vi "Results_file_Plotter.vi"(2 "flushAll":bool) -> ()   [LabVIEW 2022 SP3]
uses:
  Anemometry/Anemometry Sub Vis/Data_plotting_vis/Plotter_Mode.ctl
  Anemometry/Anemometry Sub Vis/Data_plotting_vis/Data_File_Type.ctl
  subVIs/PlotProperty.ctl
  <vilib>/Math Plots/3D Math Plots/3D Surface/3D Surface XCtrl/3D Surface.xctl
  <vilib>/Math Plots/3D Math Plots/3D Stem/3D Stem XCtrl/3D Stem.xctl
  Anemometry/Anemometry Sub Vis/File/Setup_Filetype.ctl
  Anemometry/Anemometry Sub Vis/Controls/Global_mode.ctl
  Anemometry/Anemometry Sub Vis/Data_plotting_vis/Error_bars_index.ctl
  Anemometry/Anemometry Sub Vis/Data_plotting_vis/All_Setup.ctl
  <vilib>/Utility/miscctls.llb/LVBoundsTypeDef.ctl
  35570bf4-7d7d-495b-8c89-e9310c8e2c93.vi
  f4d116b7-bb04-d342-9616-30c9bd5cd225.vi
  50b9f45c-b768-454c-9e58-04e6880f7924.vi
  443f2c7a-355d-e746-9bc2-19f18202945d.vi
  c22539af-4616-b947-8dc9-59d74accf1f9.vi
  <vilib>/Utility/error.llb/Trim Whitespace One-Sided.vi
  Anemometry/Anemometry Sub Vis/Globals/Constants_global.vi
  Anemometry/Anemometry Sub Vis/Data_plotting_vis/Results_plotter_Global.vi
  <vilib>/picture/3D Picture Control/Helpers/Set Light (no reference).vi
  <vilib>/picture/3D Picture Control/Object/Add Object (reference).vi
  subVIs/Plot_Values_Global.vi
  <vilib>/Math Plots/3D Math Plots/3D Stem/3D Stem Datatype/Public/Plot Helper (Matrix).vi
  <vilib>/Analysis/1siggen.llb/Ramp Pattern by Delta.vi
  <vilib>/Math Plots/3D Math Plots/3D Surface/3D Surface Datatype/Public/Plot Helper (Matrix).vi
  Instance           1 28Saved   Results_file_Plotter .vi
  subVIs/RFP_Table_Global.vi
  Anemometry/Anemometry Sub Vis/Globals/Meas_global.vi
  Anemometry/Anemometry Sub Vis/Globals/Plug_in_data_global.vi
  Anemometry/Anemometry Sub Vis/Globals/Trav_pos_global.vi
  <vilib>/picture/3D Picture Control/NI_3D Picture Control.lvlib
  <vilib>/Math Plots/3D Math Plots/3D Surface/3D Surface Datatype/3D Surface Datatype.lvclass
  <vilib>/Math Plots/3D Math Plots/3D Stem/3D Stem Datatype/3D Stem Datatype.lvclass
  f03f3b4b-6808-4e33-b687-4131ee4846c6.vi
  <vilib>/Analysis/NI_AALBase.lvlib
  <vilib>/Analysis/NI_AALPro.lvlib
panel:
  out "whereNext 3":string="Time to save setup?"
  out "whereNext 2":string="Time to save setup?"
  out "Time to Save Setup?":bool
  out "closePressed":bool=TRUE
  out "Template Last Mod":timestamp
  out "Index when last displayed":i32
  in  "Tab Control":T1(tab)
  in  "revealDataFiles":bool
  in  "Template":path=path ""
  in  "flushFiles":bool
  in  "Result files to read":path[](array[path])
  in  "Add results file":bool
  in  "File Types to Read":T2
  in  "SearchX":string
  in  "SearchY":string
  in  "Show Results Space Analysis":bool
  in  "Show Plot Space Analysis":bool
  in  "Multi Ordinate":i32[](listbox)
  in  "Absisca":u16(ring) items=["3818592258.491 3818596078.981 3818596814.909", "Camserver Camserver Camserver", "2025-01-01 09 04 2025-01-01 10", "Current File", "Current File 1st Folder level", "Current File 2nd Folder level", "Current File 3rd Folder level", "Current File 4th Folder level", "Current File Number", "Current Filepath", "Template File Used"]
  in  "revealOutputFile":bool
  in  "openJobDir":bool
  in  "Job Directory":path
  in  "Save Averaged rows":bool
  in  "Save Surface Fit":bool
  in  "Output Filename":path
  in  "Save Data in Rows":bool
  in  "Save Plot data":bool
  in  "Header":string
  in  "Process Point":bool
  in  "Kill Point":bool
  out "dataTable":string[][](table)
  in  "ShowPix":bool
  in  "picMode":enum32{"Scrub", "Jump"}(radio)=enum."Jump"
  in  "Post Process Plotted Data":bool
  in  "...using routine":string(combo)
  in  "Calculate new metadata":bool
  in  "Add /Edit metadata":bool
  in  "Delete Plotted data from file":bool
  in  "Raw DF in Orig Pos?":bool
  in  "Edit Raw Data Files?":bool
  in  "Point ID":u16(ring) items=["None", "3818592258.491 3818596078.981 3818596814.909", "Camserver Camserver Camserver", "2025-01-01 09 04 2025-01-01 10", "Current File", "Current File 1st Folder level", "Current File 2nd Folder level", "Current File 3rd Folder level", "Current File 4th Folder level", "Current File Number", "Current Filepath", "Template File Used"]
  in  "Won":bool=TRUE
  in  "Von":bool=TRUE
  in  "Uon":bool=TRUE
  in  "Zon":bool=TRUE
  in  "Yon":bool=TRUE
  in  "Xon":bool=TRUE
  in  "W Ch Name":u16(ring) items=["None", "3818592258.491 3818596078.981 3818596814.909", "Camserver Camserver Camserver", "2025-01-01 09 04 2025-01-01 10", "Current File", "Current File 1st Folder level", "Current File 2nd Folder level", "Current File 3rd Folder level", "Current File 4th Folder level", "Current File Number", "Current Filepath", "Template File Used"]
  in  "V Ch Name":u16(ring) items=["None", "3818592258.491 3818596078.981 3818596814.909", "Camserver Camserver Camserver", "2025-01-01 09 04 2025-01-01 10", "Current File", "Current File 1st Folder level", "Current File 2nd Folder level", "Current File 3rd Folder level", "Current File 4th Folder level", "Current File Number", "Current Filepath", "Template File Used"]
  in  "U Ch Name":u16(ring) items=["None", "3818592258.491 3818596078.981 3818596814.909", "Camserver Camserver Camserver", "2025-01-01 09 04 2025-01-01 10", "Current File", "Current File 1st Folder level", "Current File 2nd Folder level", "Current File 3rd Folder level", "Current File 4th Folder level", "Current File Number", "Current Filepath", "Template File Used"]
  in  "stl Filename":u16(ring) items=["None", "3818592258.491 3818596078.981 3818596814.909", "Camserver Camserver Camserver", "2025-01-01 09 04 2025-01-01 10", "Current File", "Current File 1st Folder level", "Current File 2nd Folder level", "Current File 3rd Folder level", "Current File 4th Folder level", "Current File Number", "Current Filepath", "Template File Used"]
  in  "Coord System":u16(ring) items=["None", "3818592258.491 3818596078.981 3818596814.909", "Camserver Camserver Camserver", "2025-01-01 09 04 2025-01-01 10", "Current File", "Current File 1st Folder level", "Current File 2nd Folder level", "Current File 3rd Folder level", "Current File 4th Folder level", "Current File Number", "Current Filepath", "Template File Used"]
  in  "Wind Direction":u16(ring) items=["None", "3818592258.491 3818596078.981 3818596814.909", "Camserver Camserver Camserver", "2025-01-01 09 04 2025-01-01 10", "Current File", "Current File 1st Folder level", "Current File 2nd Folder level", "Current File 3rd Folder level", "Current File 4th Folder level", "Current File Number", "Current Filepath", "Template File Used"]
  in  "X Ch Name":u16(ring) items=["None", "3818592258.491 3818596078.981 3818596814.909", "Camserver Camserver Camserver", "2025-01-01 09 04 2025-01-01 10", "Current File", "Current File 1st Folder level", "Current File 2nd Folder level", "Current File 3rd Folder level", "Current File 4th Folder level", "Current File Number", "Current Filepath", "Template File Used"]
  in  "Y Ch Name":u16(ring) items=["None", "3818592258.491 3818596078.981 3818596814.909", "Camserver Camserver Camserver", "2025-01-01 09 04 2025-01-01 10", "Current File", "Current File 1st Folder level", "Current File 2nd Folder level", "Current File 3rd Folder level", "Current File 4th Folder level", "Current File Number", "Current Filepath", "Template File Used"]
  in  "Z Ch Name":u16(ring) items=["None", "3818592258.491 3818596078.981 3818596814.909", "Camserver Camserver Camserver", "2025-01-01 09 04 2025-01-01 10", "Current File", "Current File 1st Folder level", "Current File 2nd Folder level", "Current File 3rd Folder level", "Current File 4th Folder level", "Current File Number", "Current Filepath", "Template File Used"]
  in  "exportSetup":bool
  in  "importSetup":bool
  in  "Save Setup":bool
  in  "loadSetup":bool
  out "setupOrINI":path
  out "loadingSetup":bool
  out "importingSetup":bool
  in  "Add Inlet Temperature offset":bool
  in  "Plot EnFlo Tunnel Display":bool
  in  "Choose\nPlug ins":bool
  in  "Reload Interval (s)":dbl=200.0 min=10.0 step=20.0
  in  "Save Setup Interval (s)":dbl=600.0
  out "Uadvec":dbl
  in  "Per Block Plug Ins Extra":string[](array[string])
  in  "Max no of filter options":i32=2000
  in  "Additional Y Values":dbl[](array[numeric]) format="%.2f"
  in  "Additional X Values":dbl[](array[numeric]) format="%.2f"
  in  "notSelectors?":bool
  in  "graphBackground":u32(colorbox)=16777222
  in  "axes":T3(ring)
  in  "brewSelect":i32 min=0 max=3 step=1
  in  "seriesColours":enum32{"Item 0", "Item 1"}(radio)
  in  "SeriesColouring":T5={"PlotVariable"=enum."Symbol", "YellowSelector"=enum."Colour", "RedSelector"=enum."Shade"}
  in  "InterpolationStyle":T6(ring)=enum."Line"
  in  "TinyPoints?":bool
  out "-4":string="Graph Scales"
  out "-3":string="Graph Scales"
  in  "printFP":bool
  out "-2":string="Graph Scales"
  out "loop":i32
  out "-1":string="Graph Scales"
  out "reloadPending":bool
  out "nRows":i32
  out "loadTime(s)":dbl format="Load: %#_3g s"
  in  "stop":bool
  out "Current":string="Graph Scales"
  in  "Single Series":i32[](listbox)=[0]
  in  "Edit Template File":bool
  in  "Filter Bins 2":i32[](listbox)=[0]
  in  "Filter 5":u16(ring)
  in  "Filter 4":u16(ring)
  in  "Filter 3":u16(ring)
  in  "Filter Array":u16[](array[ring])=[0, 0, 0, 0, 0, 0] items=["Don't Filter", "Data Plane", "3818592258.491 3818596078.981 3818596814.909", "Camserver Camserver Camserver", "2025-01-01 09 04 2025-01-01 10", "Current File", "Current File 1st Folder level", "Current File 2nd Folder level", "Current File 3rd Folder level", "Current File 4th Folder level", "Current File Number", "Current Filepath", "Template File Used"]
  in  "Filter Bins 1":i32[](listbox)=[0]
  in  "Create picture Vi Name":string(combo) caption="Picture VI:"
  in  "passToPictureVI":bool
  in  "Reload Files":bool
  out "underCursor":string
  in  "FOV":u8(slide)=4 min=4 max=100 scale=100.0..4.0
  in  "graphPaneTab":T7(tab)
  in  "histOn":bool
  in  "color and symbol":bool
  in  "forceX0":bool
  in  "forceY0":bool
  in  "Transpose":bool
  in  "refresh":bool
  out "Histogram":cluster{"Histogram":i32[], "Axis":dbl[]}[](graph)
  out "XY Plot":cluster{"Array":dbl[], "Array":dbl[]}[](graph)
  in  "Bkgnd Value":dbl
  out "Surface Integral":dbl format="%^_4g"
  out "Surface Average":dbl format="%^#.4g"
  in  "Plot Resolution":bool
  in  "Resolution":dbl=1.0 min=0.0 format="%.4f"
  in  "Point Size":i32(slide)=1 scale=0.0..5.0
  in  "No of Contours":i32(slide)=20 scale=0.0..20.0
  out "Surface Area":dbl format="%^_6g"
  out "Warning!":string
  out "Intensity Graph":dbl[][](graph)
  out "3D Surface":refnum<class "3D Plot Datatype.lvclass">[](xcontrol)
  out "3D Stem":refnum<class "3D Plot Datatype.lvclass">[](xcontrol)
  in  "3Dcontrols":enum32{"Vectors", "STL", "Cam"}(tab)
  in  "Key":dbl(ramp)
  out "scalar":string
  in  "vectorDims":cluster{"vectorSize":sgl, "vectorScale":dbl}={"vectorSize"=3.0, "vectorScale"=5.0} {"vectorScale" min=1.0 max=1000.0; "vectorSize" min=1 max=50 format="%#_3g"}
  in  "keySettings":T8 {"clipPercentile" min=0.0 max=100.0 step=0.1 format="%#_g%%"}
  in  "Tunnel":cluster{"colour":u32, "Alpha":sgl}={"colour"=16630148, "Alpha"=1.0} {"Alpha" min=0.2 max=1 step=0.02}
  in  "axesLength":dbl=150.0
  in  "BGcolour":u32(colorbox)=2829099
  in  "TTshift":T9={"STLscale"=1.0, "STLdTheta"=0.0, "Translation"={"dX"=0.0, "dY"=0.0, "dZ"=0.0}} {"STLdTheta" min=0.0 max=360.0 step=1.0}
  in  "Turntable":cluster{"colour":u32, "Alpha":sgl}={"colour"=32639, "Alpha"=1.0} {"Alpha" min=0.2 max=1 step=0.02}
  in  "Light State":bool
  in  "lightPos":cluster{"X":dbl, "Y":dbl, "Z":dbl}={"X"=-15000.0, "Y"=2000.0, "Z"=2000.0}
  in  "depthClipping":cluster{sgl, sgl}(slide)={0.001, 10.0} scale=0.001..20.0 scale format="%.0pm"
  in  "3D Picture":refnum<vi>(3d-picture)
  out "error out":errorcluster
  out "Array":errorcluster[](array[cluster])
  in  "Vector Plot?":bool
  in  "Dot Plot?":bool
  in  "Intensity Plot?":bool
  in  "MakeMovie":bool
  in  "3Dplotter":bool
  out "3DrawDataPath":path
  out "cursorDrag":bool
  out "RD_Folders":path[](array[path])
  out "whereNext":string="Time to save setup?"
  out "Template Changed?":bool
  in  "Results files chosen":path[](array[path])
  out "File Index":i32
  in  "Filter Bins 2 Strings":string[](array[string])
  in  "Filter Bins 1 Strings":string[](array[string])
  in  "Filters 3 onwards":string[](array[string])
  out "Edit Raw Data Header Info":bool
  out "Non-Blank Rows":bool[](array[boolean])
  out "Plotted rows only?":bool
  in  "type specifier":refnum<vi>
  in  "type specifier2":refnum<vi>
  out "Filetype":string[](array[string])
  out "Plotted Series":bool[][](array[boolean])
  out "Accept Array":bool[][](array[boolean])
  out "Chosen Path":path
  out "Cursor index":i32
  out "Selected Row":i32
  out "justCursorPt":bool
  out "Template Single Values":string[](array[string])
  out "Tolerances":dbl[](array[numeric]) format="%.2f"
  out "Mode":T10
  in  "Full_Res_Results_Folder":path
  in  "VI Refnum Calculation":refnum<vi>
  out "Index when last plotted":i32
  out "tunnelSTLbits":refnum<vi>[](array[refnum])
  out "tunnelRef":refnum<vi>
  out "TTstlBits":refnum<vi>[](array[refnum])
  out "axesRef":refnum<vi>
  out "TTref":refnum<vi>
  out "worldRef":refnum<vi>
  in  "modelColours":u32[](array[colorbox])=[8636267, 16545852, 3381759, 16761088]
  # "Space to put spare indicators for testing"
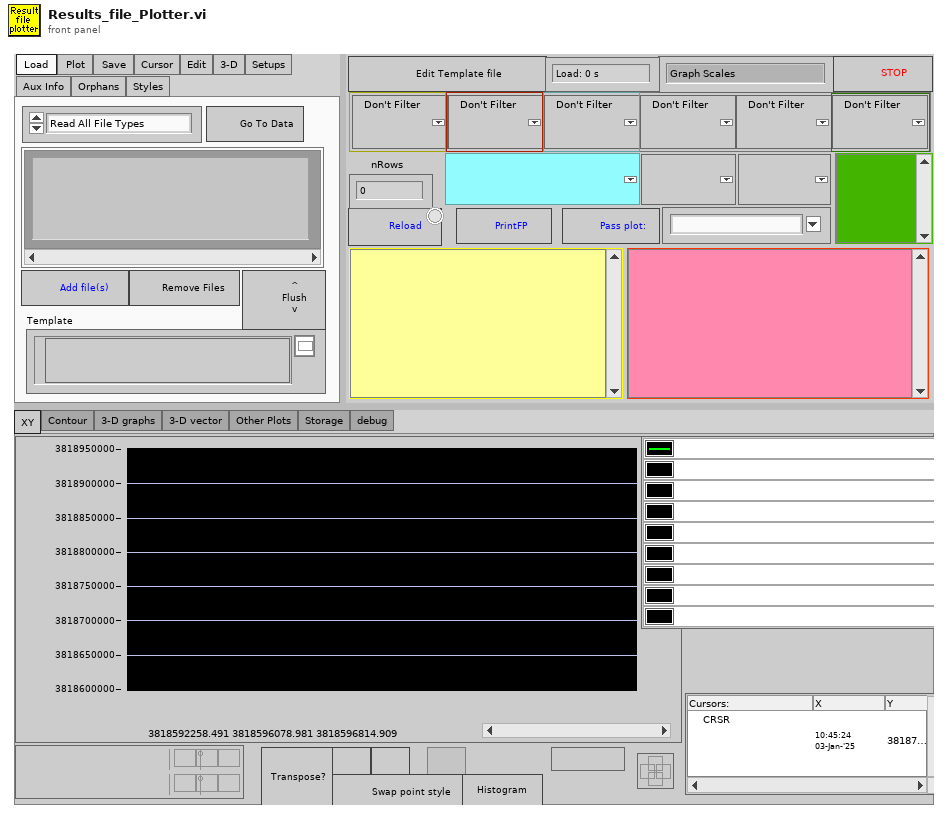
[diagram p1: front panel]
types:
  T1 = enum32{"Load ", "Plot ", "Save ", "Cursor", "Edit", "3-D", "Setups", "Aux Info", "Orphans", "Styles"}
  T2 = typedef "Data_File_Type.ctl" = enum16{"Read All File Types", "Results Files Only", "Raw Data Files Only", "Calibration Files Only", "Gas Desk Files Only", "Old Results Files Only", "Tabulated Data Files Only"}
  T3 = enum16{"X lin Y lin", "X log Y log", "X log Y lin", "X lin Y log"}
  T4 = typedef "PlotProperty.ctl" = enum16{"Colour", "Symbol", "Shade", "Size"}
  T5 = cluster{"PlotVariable":T4, "YellowSelector":T4, "RedSelector":T4}
  T6 = enum16{"Points", "StepLeft", "Line", "StepRight", "StepCentre", "StepEdge"}
  T7 = enum32{"XY", "Contour", "3-D graphs", "3-D vector", "Other Plots", "Storage", "debug"}
  T8 = cluster{"Centre Value":enum16{"Median", "Zero"}, "clipPercentile":dbl}
  T9 = cluster{"STLscale":dbl, "STLdTheta":dbl, "Translation":cluster{"dX":sgl, "dY":sgl, "dZ":sgl}}
  T10 = typedef "Plotter_Mode.ctl" = enum16{"Save file", "Delete unwanted rows", "Edit Values with constants", "Edit values per row", "Edit Raw Data file header", "Post Process Plotted Rows", "Plot EnFlo Tunnel Display", "Add Inlet Temperature Offset"}
  T11 = enum32{"XY", "Contour", "3-D graphs", "3-D vector", "Other Plots", "Storage"}
  T12 = enum16{"Zero or one", "One", "Zero or more", "One or more"}
  T13 = typedef "Global_mode.ctl" = enum16{"Read Global", "Load Global From File", "Write Global to File"}
  T14 = enum32{"Invalid", "Standard", "Closed", "Hidden", "Minimized", "Maximized"}
  T15 = enum16{"Edit Existing Template File", "Create New Template File"}
  T16 = enum16{"Show only data summary", "Show data summary", "No data summary"}
  T17 = typedef "All_Setup.ctl" = cluster{"Result files to read":path[], "Template":path, "Transpose":bool, "Additional X Values":dbl[], "Additional Y Values":dbl[], "Output Filename":path, "Create Picture Vi Name":string, "Intensity Plot?":bool, "Multi Ordinate":string[], "Abscissa String":string, "Filter Array":string[], "Filter Bins 1 Strings":string[], "Filter Bins 2 Strings":string[], "Filters 3 onwards":string[], "nRows":i32}
  T18 = typedef "Setup_Filetype.ctl" = enum16{"Measurement Setups", "Calibration Setups", "General", "Results File Plotter Setups", "Speed Calib Tweaks"}
  T19 = enum16{"Left Button", "Center Button", "Right Button", "Window Close"}
  T20 = cluster{"Filter Bins 2":i32[], "Filter Bins 1":i32[], "Point Size":i32, "color and symbol":bool, "No of Contours":i32, "Resolution":dbl, "Transpose":bool, "Absisca":u16, "Multi Ordinate":i32[], "Accept Array":bool[][], "Intensity Plot?":bool, "Additional X Values":dbl[], "Additional Y Values":dbl[], "3D Ch Selectors":i32[]}
  T21 = typedef "Error_bars_index.ctl" = cluster{"Upper":i32, "Lower":i32, "St Error":i32}
  T22 = typedef "LVPointTypeDef.ctl" = cluster{"Horizontal":i16, "Vertical":i16}
  T23 = typedef "LVRectTypeDef.ctl" = cluster{"Left":i16, "Top":i16, "Right":i16, "Bottom":i16}
  T24 = cluster{"X Max":dbl, "Y Max ":dbl, "X Scale":cluster{"Xo":dbl, "delta X":dbl}, "Y Scale":cluster{"Xo":dbl, "delta X":dbl}, "X Values":dbl[], "Y Values":dbl[], "Z Max":dbl, "Z Min":dbl}
  T25 = typedef "coordSys.ctl" = enum16{"Tunnel", "Model"}
  T26 = cluster{"coordSys":T25, "WD":dbl, "STL":string}[]
  T27 = typedef "Group_Binning.ctl" = cluster{"Index":i32, "Tolerance":dbl, "Precision":string}
  T28 = typedef "LVBoundsTypeDef.ctl" = cluster{"Width":u32, "Height":u32}
  T29 = enum8{"Enabled", "Disabled", "Disabled and Grayed Out"}
  T30 = enum16{"Normal Bin", "Opaque Bin", "Transparent Bin"}
  T31 = typedef "RFP_Plot_Metadata.ctl" = cluster{"Row Number":i32[], "Error Bars":T21, "X Label":string, "Y Label":string, "Blanks NaNs":i32[]}
  T32 = typedef "LVPoint32TypeDef.ctl" = cluster{"Horizontal":i32, "Vertical":i32}
  T33 = typedef "LVRGBAColorTypeDef.ctl" = cluster{"Red":sgl, "Green":sgl, "Blue":sgl, "Alpha":sgl}
  T34 = cluster{"Shift":bool, "Ctrl":bool, "Alt":bool, "Cmd":bool, "Opt":bool}
  T35 = enum16{"Inherit Material", "Use entire Material", "Ignore Ambient", "Ignore Diffuse", "Ignore Specular", "Ignore Emission", "Ignore Ambient and Diffuse"}
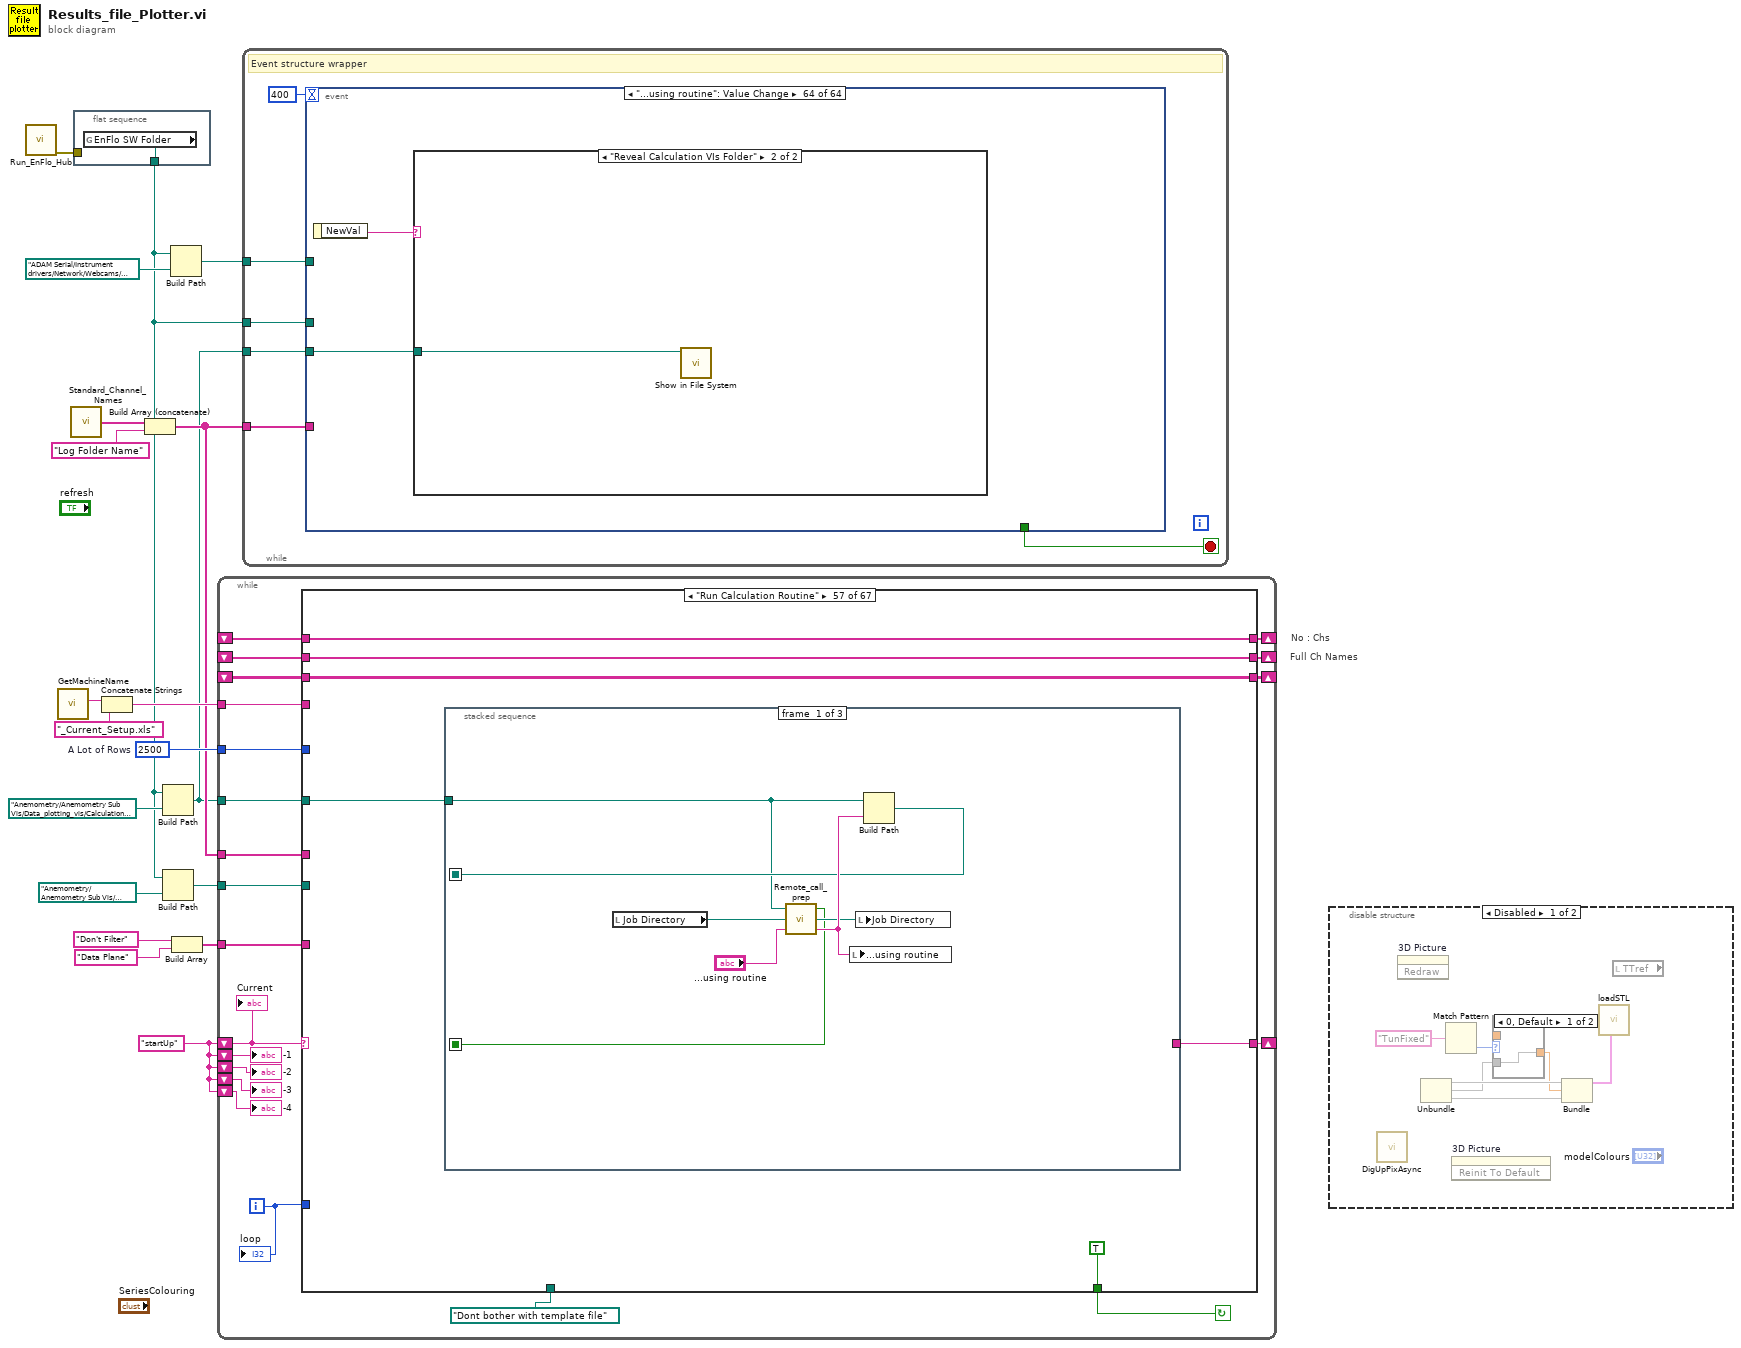
[diagram p0: block diagram]
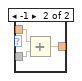
[diagram p2: hidden frame]
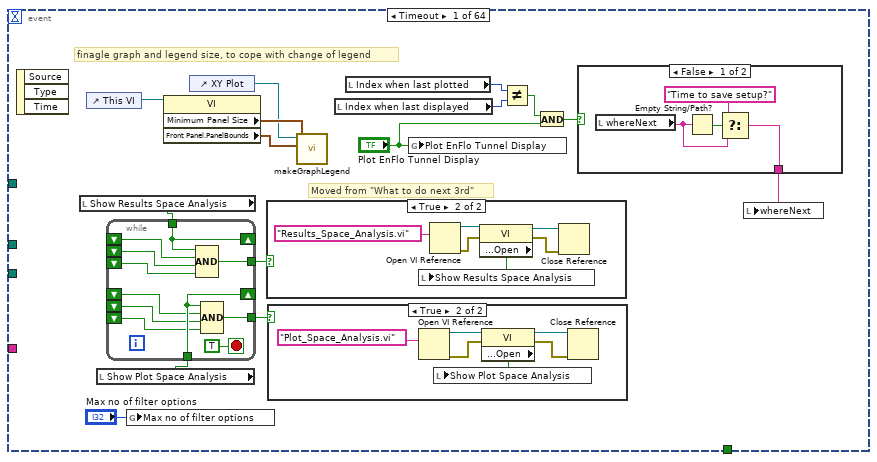
[diagram p4: hidden frame]
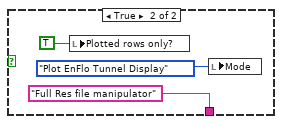
[diagram p5: hidden frame]
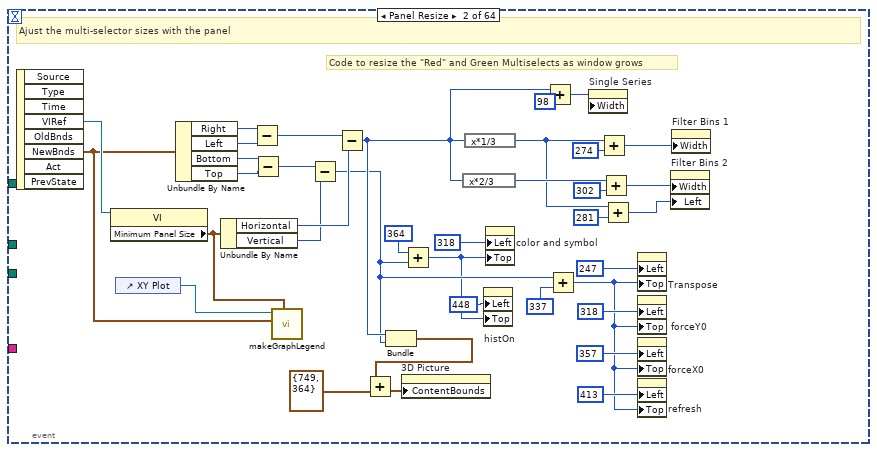
[diagram p8: hidden frame]
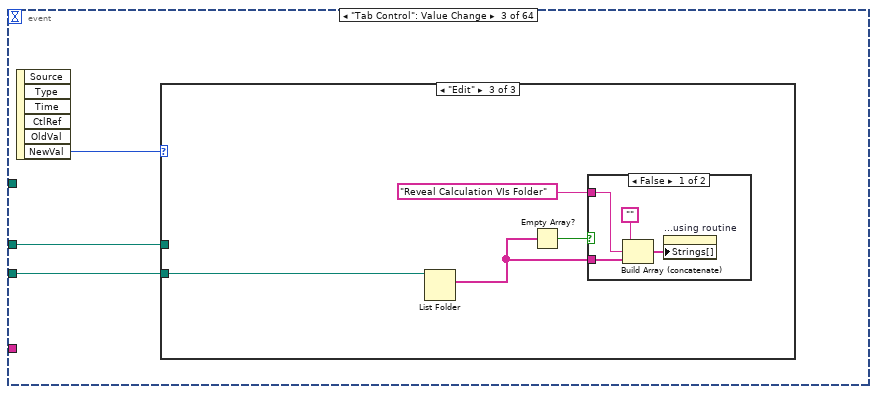
[diagram p9: hidden frame]
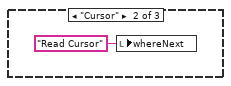
[diagram p11: hidden frame]
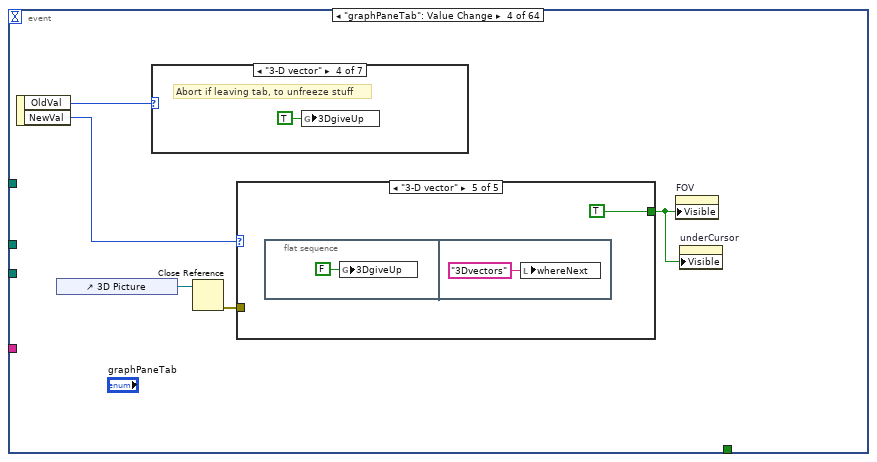
[diagram p13: hidden frame]
diagram:
  w19 = 2500  # A Lot of Rows
  w3 = "startUp"
  # "No : Chs"
  # "Full Ch Names"
  n1 = call "Run_EnFlo_Hub.vi"() -> ("Error Out"=w6:errorcluster)  [unwired: 1 in, 6 out]
  n2 = call "GetMachineName.vi"() -> ("ComputerName"=w16:string)  [unwired: 11 in]
  n3 = call "Standard_Channel_Names.vi"() -> ("Standard Ch Names"=w15:string[])  [unwired: 1 in]
  n4 = flat-sequence {
    tunnel: [w20] -> w2
    tunnel: w6 -> [_]
    frame #0 {
      n5 = global read "Constants_global.vi" "EnFlo SW Folder"() -> (w20:path)
    }
  }
  n6 = Concatenate Strings(w16, "_Current_Setup.xls" ("Setup filename")) -> (w17:string)
  n7 = Build Array (concatenate)(w15, "Log Folder Name") -> (w13:string[])
  n8 = Build Path(base path=w2, name or relative path=path "Anemometry/Anemometry Sub Vis/Data_plotting_vis/Calculation Vis") -> (appended path=w1:path)
  n9 = Build Path(base path=w2, name or relative path=path "Anemometry/Anemometry Sub Vis/Data_plotting_vis/XY Plot Vis") -> (appended path=w8:path)
  n10 = Build Path(base path=w2, name or relative path=path "ADAM Serial/Instrument drivers/Network/Webcams/RetrievePix.vi") -> (appended path=w4:path)
  n11 = Build Array("Don't Filter" ("Input Element"), "Data Plane" ("Input Element")) -> (w10:string[])
  n12 = while {
    shift-left: _ -> [w35]
    shift-right: [w36] -> _
    shift-left: w3 -> [w39]
    shift-right: [w34] -> _
    shift-left: _ -> [w37]
    shift-right: [w41] -> _
    tunnel: w19 -> [w33]
    tunnel: w17 -> [w32]
    tunnel: w13 -> [w29]
    shift-right: [w31] -> _
    shift-left: _ -> [w30]
    shift-left: w3 -> [w28]
    shift-left: w3 -> [w26]
    tunnel: w10 -> [w25]
    tunnel: w8 -> [w24]
    tunnel: w1 -> [w23]
    shift-left: w3 -> [w22]
    shift-left: w3 -> [w21]
    i -> [w27]
    stop <- w40 continue-if-true
    n13 = case shown="\"Run Calculation Routine\"" w39 {
      selector: w39 -> [_ _ _ _ _ _ _ _ _ _ _ _ _ _ _ _ _ _ _ _ _ _ _ _ _ _ _ _ _ _ _ _ _ _ _ _ _ _ _ _ _ _ _ _ _ _ _ _ _ _ _ _ _ _ _ _ _ _ _ _ _ _ _ _ _ _ w3667]
      tunnel: w37 -> [w63 w98 _ w147 w179 w217 w245 w266 w319 w335 w352 w412 w464 w497 w559 w600 w621 w642 w654 w714 w729 w776 w1079 w1151 w1200 w1227 w1240 w1275 w1303 w1450 w1478 w1563 w1895 w1912 w1919 w1937 w1947 w1953 w1973 w2040 w2122 w2145 w2169 w2219 w2266 w2285 w2305 w2519 w2535 w2556 w2637 w2781 w2829 w2842 w2851 w2909 w2927 w2968 w3072 w3123 w3544 w3554 w3616 w3632 w3637 w3658 w3672]
      tunnel: [w63 w98 w119 w147 w179 w217 w245 w263 w319 w335 w365 w423 w464 w497 w559 w600 w621 w642 w654 w714 w729 w776 w1079 w1151 w1200 w1227 w1240 w1275 w1303 w1450 w1478 w1562 w1895 w1912 w1919 w1937 w1947 w1953 w1973 w2040 w2122 w2145 w2169 w2219 w2266 w2285 w2304 w2519 w2535 w2555 w2631 w2781 w2829 w2842 w2851 w2909 w2927 w2968 w3072 w3124 w3544 w3555 w3616 w3632 w3637 w3658 w3672] -> w41
      tunnel: [w52 w72 w110 w136 w174 "Template Required?" "More files options" w267 "Load Data" "Load Data" w363 w421 w466 w495 "Load Selectors" "Perform Global Concatenate" "What is present?" "Ordinate Selector Type" "Which rows are Non-Blank?" w698 "Create Selectors" w764 w1078 w1150 "Re Plot Data?" w1225 "Prepare Filter2 strings" "Plot Data" w1301 "Add Axis names" "Analyse Plot Space" w1564 "What to do next?" ("t") "What to do next?" ("t") "What to do next?" "What to do next?" ("t") "What to do next?" ("t") w1954 w1976 "Check modification dates?" w2118 w2142 "Ordinate Selector Type" w2222 "Initialise" ("t") w2273 w2306 w2511 "Create Selectors" w2557 w2638 w2779 w2822 w2833 w2855 "Create Selectors" w2925 w2971 w3060 w3137 "Initialise" ("t") w3553 "Time to save setup?" "initialise" "Initialise" "" "Initialise"] -> w34
      tunnel: [TRUE TRUE TRUE TRUE TRUE ("T button?") TRUE TRUE TRUE TRUE TRUE w378 TRUE ("OK?") TRUE ("OK?") TRUE ("OK?") TRUE ("OK?") TRUE TRUE TRUE TRUE TRUE TRUE TRUE w1077 w1149 TRUE TRUE TRUE TRUE w1302 TRUE TRUE ("OK?") TRUE TRUE ("OK?") TRUE ("OK?") TRUE TRUE ("OK?") TRUE ("OK?") TRUE ("OK?") TRUE ("OK?") TRUE ("OK?") TRUE TRUE TRUE TRUE TRUE TRUE TRUE TRUE ("OK?") TRUE ("OK?") TRUE TRUE TRUE TRUE TRUE TRUE TRUE TRUE TRUE TRUE TRUE TRUE w3551 TRUE ("OK?") TRUE ("OK?") TRUE ("OK?") FALSE FALSE] -> w40
      tunnel: path "Dont bother with template file" ("Template File") -> [_ _ _ _ _ w212 _ _ _ _ _ _ _ _ _ _ _ _ _ _ _ _ _ _ _ _ _ _ _ _ _ _ _ _ _ _ _ _ _ _ _ _ _ _ _ _ _ _ _ _ _ _ _ _ _ _ _ _ _ _ w3539 _ _ _ _ w3657 _]
      tunnel: [w62 w97 w119 w146 w180 w216 w244 w265 w317 w333 w366 w422 w463 w498 w552 w597 w624 w643 w683 w707 w728 w770 w1080 w1152 w1199 w1224 w1233 w1270 w1300 w1447 w1465 w1559 w1896 w1913 w1917 w1938 w1948 w1970 w1977 w2042 w2121 w2144 w2168 w2220 w2267 w2284 w2299 w2520 w2537 w2551 w2634 w2789 w2830 w2843 w2866 w2910 w2928 w2972 w3073 w3125 w3545 w3557 w3617 w3633 w3638 w3659 w3669] -> w36
      tunnel: w35 -> [w62 w97 _ w146 w180 w216 w244 w264 w317 w333 w353 w410 w463 w498 w552 w597 w624 w643 w683 w707 w728 w770 w1080 w1152 w1199 w1224 w1233 w1270 w1300 w1447 w1465 w1558 w1896 w1913 w1917 w1938 w1948 w1970 w1977 w2042 w2121 w2144 w2168 w2220 w2267 w2284 w2298 w2520 w2537 w2553 w2633 w2789 w2830 w2843 w2866 w2910 w2928 w2972 w3073 w3126 w3545 w3556 w3617 w3633 w3638 w3659 w3669]
      tunnel: w27 -> [_ _ _ w135 _ _ _ _ _ _ _ _ _ _ _ _ _ _ _ _ _ w759 _ _ _ _ _ _ w1299 _ _ _ _ _ _ _ _ _ w1975 _ _ _ _ _ _ _ _ _ _ _ _ _ _ _ _ _ _ _ _ _ _ _ _ _ _ _ _]
      tunnel: w33 -> [_ _ _ _ _ _ _ _ _ _ _ _ _ _ _ _ _ _ _ _ _ _ _ _ _ _ _ _ _ _ _ _ _ _ _ _ _ _ _ _ _ w2141 _ _ _ _ _ _ _ _ _ _ _ _ _ _ _ w2967 _ w3132 _ _ _ _ _ _ _]
      tunnel: w32 -> [_ w96 _ _ _ _ _ _ _ _ _ _ _ _ _ _ _ _ _ _ _ _ _ _ _ _ _ _ _ _ _ _ _ _ _ _ _ _ _ _ _ _ _ _ _ _ _ _ _ _ _ _ _ _ _ _ _ _ _ _ _ w3552 _ _ _ _ _]
      tunnel: w29 -> [_ _ _ _ _ _ _ _ _ _ _ _ w458 _ _ _ _ _ _ _ _ _ _ _ _ _ _ _ _ _ _ _ _ _ _ _ _ _ _ _ _ _ _ _ _ _ _ _ _ _ _ _ _ _ _ _ _ _ _ _ _ _ _ _ _ _ _]
      tunnel: [w56 w95 string[][] [] w132 w171 w208 w240 w256 w315 w325 w364 w416 w461 w494 w558 w596 w616 w639 w681 w702 w724 w752 w1076 w1148 w1189 w1221 w1230 w1267 w1298 w1446 w1459 w1555 w1884 w1909 w1915 w1934 w1944 w1971 w1972 w2031 w2110 w2138 w2165 w2218 w2261 w2282 w2294 w2510 w2525 w2545 w2628 w2777 w2825 w2832 w2849 w2896 w2924 w2965 w3059 w3122 w3536 w3550 w3613 w3635 w3641 w3651 w3668] -> w31
      tunnel: w30 -> [w56 w95 _ w132 w171 w208 w240 w257 w315 w325 w367 w417 w461 w494 w558 w596 w617 w639 w681 w702 w724 w752 w1076 w1148 w1189 w1221 w1230 w1267 w1298 w1446 w1459 w1554 w1884 w1909 w1915 w1934 w1944 w1971 w1972 w2031 w2110 w2138 w2165 w2218 w2261 w2282 w2296 w2510 w2525 w2548 w2629 w2777 w2825 w2832 w2849 w2896 w2924 w2965 w3059 w3121 w3536 w3549 w3613 w3635 w3641 w3651 w3668]
      tunnel: w25 -> [_ _ _ _ _ _ _ _ _ _ _ _ _ w493 w550 w595 _ _ _ _ _ _ _ _ _ _ w1229 w1266 _ _ _ _ _ _ _ _ _ _ _ _ _ _ _ _ _ _ _ _ _ _ _ _ _ _ _ _ _ _ _ _ _ w3548 _ _ _ _ _]
      tunnel: w24 -> [_ w91 _ _ _ _ _ _ _ _ _ _ _ _ _ _ _ _ _ _ _ _ _ _ _ _ _ _ _ _ _ _ _ _ _ _ _ _ _ _ _ _ _ _ _ _ _ _ _ _ _ _ _ _ _ _ _ _ w3058 _ _ _ _ _ _ _ _]
      tunnel: w23 -> [_ w90 _ _ _ _ _ _ _ _ _ _ _ _ _ _ _ _ _ _ _ _ _ _ _ _ _ _ _ _ _ _ _ _ _ _ _ _ _ _ _ _ _ _ _ _ _ _ _ _ _ _ _ _ _ _ w2923 _ _ _ _ _ _ _ _ _ _]
      frame "What to do next?" {
        # "Should probably be Event-ified"
        n14 = local read "cursorDrag"() -> (w48:bool)
        n15 = Wait For Front Panel Activity(1:1000 ("timeout ms (-1 never timeout)"), 3:w48) -> ()  [unwired: 1 in, 1 out]
        n16 = Wait (ms)(milliseconds to wait=u32 10) -> ()  [unwired: 1 out]
        n17 = property on="XY Plot" class="XYGraph (strict)"() -> ("YScale.Maximum"=w43:dbl, "YScale.Minimum"=w42:dbl, "XScale.Maximum"=w55:dbl, "XScale.Minimum"=w54:dbl)  [unwired: 2 in, 2 out]
        n18 = call <vilib>:"Unset Busy.vi"() -> ()  [unwired: 11 in, 1 out]
        n19 = local read "whereNext"() -> (w46:string)
        n20 = global write "Results_plotter_Global.vi" "Y plot max"(w43) -> ()
        n21 = global write "Results_plotter_Global.vi" "Y plot min"(w42) -> ()
        n22 = global write "Results_plotter_Global.vi" "X plot max"(w55) -> ()
        n23 = global write "Results_plotter_Global.vi" "X plot min"(w54) -> ()
        n24 = Empty String/Path?(string/path=w46) -> (empty?=w45:bool)
        n25 = Select(t="Create Selectors", s=w45, f=w46) -> (s? t:f=w47:string)
        n26 = property on="Histogram" class="XYGraph (strict)"("YScale.Maximum"=w43, "YScale.Minimum"=w42) -> ()  [unwired: 2 in, 2 out]
        n27 = local read "Warning!"() -> (w60:string)
        n28 = global write "Results_plotter_Global.vi" "First Loop"(FALSE) -> ()
        n29 = Empty String/Path?(string/path=w60) -> (empty?=w59:bool)
        n30 = call "Synchronize Data Flow.vim"("input 4"=w47, "input 1"="") -> ("output 4"=w52:string, "output 1"=→"whereNext":string)  [unwired: 2 in, 2 out]
        n31 = Not(x=w59) -> (.not. x?=w58:bool)
        n32 = property on="Warning!" class="Str"("Blinking"=w58) -> ()  [unwired: 2 in, 2 out]
      }
      frame "startUp" {
        w92 = FALSE ("Save Plot data")
        n33 = List Folder(path=w91) -> (filenames=w89:string[])  [unwired: 3 in, 3 out]
        n34 = List Folder(path=w90) -> (filenames=w86:string[])  [unwired: 3 in, 3 out]
        n35 = Empty Array?(array=w86) -> (empty?=w87:bool)
        n36 = Empty Array?(array=w89) -> (empty?=w88:bool)
        n37 = global write "Results_plotter_Global.vi" "Setup Filename"(w96) -> ()
        n38 = case shown="False" w87 {
          tunnel: w86 -> [w102 _]
          frame False {
            n39 = Build Array (concatenate)("", w102) -> (w101:string[])
            n40 = property on="...using routine" class="CmbBox"("Strings[]"=w101) -> ()  [unwired: 2 in, 2 out]
          }
          frame True {
          }
        }
        n41 = case shown="False" w88 {
          tunnel: w89 -> [w104 _]
          frame False {
            n42 = Build Array (concatenate)("", w104) -> (w103:string[])
            n43 = property on="Create picture Vi Name" class="CmbBox"("Strings[]"=w103) -> ()  [unwired: 2 in, 2 out]
          }
          frame True {
          }
        }
        n44 = local read "Result files to read"() -> (w71:path[])
        n45 = local read "Template"() -> (w67:path)
        n46 = local write "color and symbol"(w92) -> ()
        n47 = local write "Reload Files"(w92) -> ()
        n48 = local write "Save Setup"(w92) -> ()
        n49 = local write "Vector Plot?"(w92) -> ()
        n50 = local write "Add results file"(w92) -> ()
        n51 = local write "Save Plot data"(w92) -> ()
        n52 = local write "Kill Point"(w92) -> ()
        n53 = local write "Save Data in Rows"(w92) -> ()
        n54 = local write "Process Point"(w92) -> ()
        n55 = local write "stop"(w92) -> ()
        n56 = local write "Post Process Plotted Data"(w92) -> ()
        n57 = local write "Save Averaged rows"(w92) -> ()
        n58 = local write "Delete Plotted data from file"(w92) -> ()
        n59 = local write "Add /Edit metadata"(w92) -> ()
        n60 = local write "Choose\nPlug ins"(w92) -> ()
        n61 = local read "importSetup"() -> (w79:bool)
        n62 = local read "loadSetup"() -> (w80:bool)
        n63 = Not A Number/Path/Refnum?(number/path/refnum=w67) -> (NaN/Path/Refnum?=w65:bool)
        n64 = call "Is Value Changed.vim"("value"=w67) -> ("changed or first call?"=w66:bool)
        n65 = Empty Array?(array=w71) -> (empty?=w68:bool)
        n66 = call "Is Value Changed.vim"("value"=w71) -> ("changed or first call?"=w70:bool)
        n67 = Compound Arithmetic op=AND(w66, invert w65) -> (w64:bool)
        n68 = Or(x=w79, y=w80) -> (x .or. y?=w76:bool)
        n69 = Compound Arithmetic op=AND(w70, invert w68) -> (w69:bool)
        n70 = Select(t="importSetup", s=w79, f="Choose Setup file" ("t")) -> (s? t:f=w75:string)
        n71 = local read "flushFiles"() -> (w84:bool)
        n72 = local read "flushAll"() -> (w83:bool)
        n73 = global write "Results_plotter_Global.vi" "Skip Dialog on these Channels"(string[] [] ("Skip Dialog on these Channels")) -> ()
        n74 = Select(t=w75, s=w76, f="Load setup") -> (s? t:f=w73:string)
        n75 = Compound Arithmetic op=OR(w83, w84, w69, w64) -> (w82:bool)
        n76 = Select(t="Initialise", s=w82, f=w73) -> (s? t:f=w72:string)
        n77 = global write "Results_plotter_Global.vi" "Tolerances"(dbl[] [] ("Tolerances")) -> ()
        n78 = property on="graphPaneTab" class="TabCtl (strict)"("Val(Sgnl)"=T11."XY" ("Value (Signaling)")) -> ()  [unwired: 2 in, 2 out]
      }
      frame "Initialise" {
        w108 = FALSE
        w119 = string[] [] ("Channel names")
        n79 = local read "flushAll"() -> (w106:bool)
        n80 = case shown="True" "flushFiles" {
          frame False {
          }
          frame True {
            n81 = local write "Result files to read"(path[] [] ("Result files to read")) -> ()
            n82 = local write "flushFiles"(FALSE ("Empty")) -> ()
          }
        }
        n83 = local write "closePressed"(w108) -> ()
        n84 = local write "stop"(w108) -> ()
        n85 = case shown="True" w106 {
          frame False {
          }
          frame True {
            n86 = local write "Result files to read"(path[] [] ("Result files to read")) -> ()
            n87 = local write "flushAll"(FALSE ("flush")) -> ()
            n88 = local write "Template"(path "") -> ()
          }
        }
        n89 = local write "Results files chosen"(path[] [] ("Results file choosen")) -> ()
        n90 = File/Directory Info(path="Template") -> (last mod=w114:timestamp)  [unwired: 1 in, 6 out]
        n91 = call "Load_Template_Globals.vi"("Non Blank Channels"=i32[] [] ("initialized array"), "Template-read"="Template") -> ()  [unwired: 1 in, 1 out]
        n92 = global write "Results_plotter_Global.vi" "Template"("Template") -> ()
        n93 = local write "Template Last Mod"(w114) -> ()
        n94 = call <vilib>:"Set Busy.vi"() -> ()  [unwired: 10 in, 2 out]
        n95 = local read "Edit Template File"() -> (w109:bool)
        n96 = Select(t="Edit template file", s=w109, f="Check Results file array" ("t")) -> (s? t:f=w110:string)
        "File Index" <- 0
        "reloadPending" <- w108
      }
      frame "Choose Setup file" {
        w139 = Setup_Filetype."Results File Plotter Setups" ("Setup File Type")
        n97 = local read "Job Directory"() -> (w130:path)
        n98 = Build Path(base path=w130, name or relative path=path "RFPsetups") -> (appended path=w128:path)
        n99 = call "Setup_Filepath.vi"("Setup File Type"=w139, "Filename in"="Test") -> ("Directory"=w141:path)  [unwired: 1 out]
        n100 = call "Last_Years_Setups.vi"("Setup File Type"=w139) -> ("Directory"=w140:path)
        n101 = call "List_files_in_order_of_age.vi"("Files to Hide"=string[] ["*.INI"], "wildcardPattern"="*.xls", "Folder"=w128) -> ("file names"=w129:string[])  [unwired: 8 in]
        n102 = call "List_files_in_order_of_age.vi"("Folder"=w141) -> ("file names"=w142:string[])  [unwired: 10 in]
        n103 = call "List_files_in_order_of_age.vi"("Folder"=w140) -> ("file names"=w143:string[])  [unwired: 10 in]
        n104 = Build Array (concatenate)(w129, w142, w143) -> (w145:string[])
        n105 = call "Analyse_string_array.vi"("String array"=w145) -> ("Unique strings"=w138:string[])  [unwired: 1 in, 1 out]
        n106 = Array Size(array=w138) -> (size(s)=w137:i32)
        n107 = case shown="1, Default" w137 {
          tunnel: w138 -> [_ w155]
          tunnel: [w149 w153] -> w136
          tunnel: w135 -> [_ w152]
          tunnel: "Initialise" ("t") -> [w149 w151]
          frame 0 {
          }
          frame 1, Default {
            n108 = call "Select_Strings.vi"("Available Ch names"=w155, "Message"="Please Choose a setup file", "Selector mode"=T12."One") -> ("Cancel"=w154:bool, "Selected Channel Names"=w150:string[])  [unwired: 2 in, 2 out]
            n109 = case shown="False" w154 {
              tunnel: ["Load setup" w167] -> w153
              tunnel: w152 -> [_ w165]
              tunnel: w151 -> [_ w162]
              tunnel: w150 -> [w158 _]
              frame False {
                n110 = Index Array(array=w158, index=0) -> (element=w160:string)
                n111 = global write "Results_plotter_Global.vi" "Setup Filename"(w160) -> ()
              }
              frame True {
                n112 = Less?(x=w165, y=3) -> (x < y?=w164:bool)
                n113 = Select(t=w162, s=w164, f="Time to save setup?") -> (s? t:f=w167:string)
              }
            }
          }
        }
        n114 = local write "loadSetup"(FALSE ("Load Setup")) -> ()
      }
      frame "Load setup" {
        n115 = global read "Results_plotter_Global.vi" "Setup Filename"() -> (w176:string)
        n116 = local read "Job Directory"() -> (w170:path)
        n117 = call "Read_Write_Plot_Setup.vi"("jobDirectory"=w170, "Mode"=enum16{"Load", "Save"}."Load", "Setup filename"=w176) -> ("OK?"=w175:bool, "setupLoaded"=w168:path, "Cluster 2"=w177:T17)  [unwired: 6 in]
        n118 = case shown="True" w175 {
          tunnel: w177 -> [_ w198]
          tunnel: ["Initialise" ("t") w185] -> w174
          tunnel: w168 -> [_ w182]
          frame False {
          }
          frame True {
            n119 = local write "setupOrINI"(w182) -> ()
            n120 = Unbundle By Name(w198) -> ("Result files to read"=w190:path[], "Template"=w183:path, "Transpose"=w192:bool, "Additional X Values"=w193:dbl[], "Additional Y Values"=w194:dbl[], "Output Filename"=w195:path, "Create Picture Vi Name"=w196:string, "Intensity Plot?"=w197:bool, "nRows"=w186:i32)
            n121 = Greater?(x=w186, y=8000) -> (0:w187:bool)
            n122 = Index Array(array=w190, index=0) -> (element=w189:path)
            n123 = case shown="False" w187 {
              tunnel: w186 -> [_ w206]
              tunnel: [w199 w201] -> w185
              tunnel: "Initialise" ("t") -> [w199 w200]
              frame False {
              }
              frame True {
                n124 = Format Into String(format string="Do you want to Load %d rows?", w206) -> (resulting string=w204:string)  [unwired: 2 in, 1 out]
                n125 = Two Button Dialog(message=w204) -> (T button?=w203:bool)  [unwired: 2 in]
                n126 = Select(t=w200, s=w203, f="Empty Results file array") -> (s? t:f=w201:string)
              }
            }
            n127 = local write "Chosen Path"(w189) -> ()
            n128 = local write "Result files to read"(w190) -> ()
            n129 = local write "Template"(w183) -> ()
            n130 = local write "Transpose"(w192) -> ()
            n131 = local write "Additional X Values"(w193) -> ()
            n132 = local write "Additional Y Values"(w194) -> ()
            n133 = local write "Output Filename"(w195) -> ()
            n134 = local write "Create picture Vi Name"(w196) -> ()
            n135 = local write "Intensity Plot?"(w197) -> ()
            n136 = global write "Results_plotter_Global.vi" "Template"(w183) -> ()
          }
        }
        n137 = local write "Tab Control"(T1."Load " ("Tab Control")) -> ()
        "loadingSetup" <- TRUE ("Load Setup")
      }
      frame "Check Results file array" {
        n138 = local read "Result files to read"() -> (w215:path[])
        n139 = local read "Template"() -> (w207:path)
        n140 = for {
          shift-right: [w228] -> w213
          shift-left: path[] [] -> [w227]
          tunnel: w215 -> [w226] mode=indexing
          shift-right: [w221] -> _
          shift-left: TRUE -> [w220]
          n141 = case shown="False" w220 {
            tunnel: w226 -> [w230 w232]
            tunnel: [w229 w231] -> w223
            frame False {
              n142 = call "Does_file_exist_(simple).vi"("Pathname"=w230) -> ("exists?"=w229:bool)
            }
            frame True {
              n143 = call "Check_Vol_Mounted.vi"("Filename"=w232) -> ("exists?"=w231:bool)  [unwired: 1 out]
            }
          }
          n144 = Search 1D Array(1D array=w227, element=w226) -> (index of element=w225:i32)  [unwired: 1 out]
          n145 = Less Than 0?(x=w225) -> (x < 0?=w222:bool)
          n146 = And(x=w222, y=w223) -> (x .and. y?=w224:bool)
          n147 = case shown="True" w224 {
            tunnel: w227 -> [w234 w238]
            tunnel: w226 -> [_ w237]
            tunnel: [w234 w236] -> w228
            tunnel: [FALSE w235] -> w221
            tunnel: w220 -> [_ w235]
            frame False {
            }
            frame True {
              n148 = Build Array (concatenate)(w238, w237) -> (w236:path[])
            }
          }
        }
        n149 = Equal?(x=w207, y=w212) -> (x = y?=w211:bool)
        n150 = global write "Results_plotter_Global.vi" "Template"(w207) -> ()
        n151 = case shown="True" w211 {
          frame False {
          }
          frame True {
            n152 = local write "Template"(path "") -> ()
          }
        }
        n153 = local write "Result files to read"(w213) -> ()
      }
      frame "Template Required?" {
        n154 = local read "Template"() -> (w243:path)
        n155 = call "Check_Vol_Mounted.vi"("Filename"=w243) -> ("Filename Out"=w242:path, "exists?"=w241:bool)
        n156 = case shown="True" w241 {
          tunnel: w242 -> [_ w250]
          tunnel: [path "" w249] -> w239
          frame False {
          }
          frame True {
            n157 = call "File_checker_and_finder.vi"("Promp if not found"="Please select Template file", "Filename In"=w250) -> ("Filename Out"=w249:path)  [unwired: 1 out]
          }
        }
        n158 = local write "Template"(w239) -> ()
        n159 = global write "Results_plotter_Global.vi" "Template"(w239) -> ()
      }
      frame "More files options" {
        n160 = global read "Results_plotter_Global.vi" "All Template Ch Names"() -> (w253:string[])
        n161 = local read "Result files to read"() -> (w262:path[])
        n162 = local read "Add results file"() -> (w259:bool)
        n163 = Array Size(array=w262) -> (size(s)=w261:i32)
        n164 = Equal To 0?(x=w261) -> (x = 0?=w260:bool)
        n165 = Empty Array?(array=w253) -> (empty?=w252:bool)
        n166 = Or(x=w260, y=w259) -> (x .or. y?=w258:bool)
        n167 = case shown="False" w258 {
          tunnel: ["Load Data" w270] -> w267
          frame False {
          }
          frame True {
            n168 = call <vilib>:"Three Button Dialog.vi"("Right Button Text (\"Cancel\")"="Import a Setup" ("Right Button Text (\"Cancel\")"), "Center Button Text (\"No\")"="An entire Folder" ("F button name (\"Cancel\")"), "Left Button Text (\"Yes\")"="One or more Files" ("T button name (\"OK\")"), "message"="Where is the data to come from?") -> ("Which Button?"=w275:T19)  [unwired: 7 in]
            n169 = case shown="\"Window Close\"" w275 {
              tunnel: ["Choose a Folder" "Choose Results File(s)" "importSetup" "What to do next?"] -> w270
              frame "Center Button" {
              }
              frame "Left Button", Default {
              }
              frame "Right Button" {
              }
              frame "Window Close" {
              }
            }
            n170 = local write "Add results file"(FALSE) -> ()
          }
        }
        n171 = case shown="False" w252 {
          tunnel: w266 -> [w286 w309]
          tunnel: [w285 w310] -> w265
          tunnel: w264 -> [_ w310]
          tunnel: [w281 w309] -> w263
          tunnel: w257 -> [w283 w308]
          tunnel: [w282 w308] -> w256
          tunnel: w253 -> [w281 _]
          frame False {
            n172 = for {
              tunnel: w286 -> [w307]
              tunnel: w281 -> [w306] mode=indexing
              tunnel: [w305] -> w284 mode=indexing
              n173 = Search 1D Array(1D array=w307, element=w306) -> (index of element=w305:i32)  [unwired: 1 in]
            }
            n174 = for {
              tunnel: w284 -> [w289]
              tunnel: w283 -> [w288] mode=indexing
              tunnel: [w287] -> w282 mode=indexing
              n175 = for {
                tunnel: w289 -> [w291] mode=indexing
                tunnel: w288 -> [w292]
                tunnel: [w290] -> w287 mode=indexing
                n176 = case shown="-1" w291 {
                  selector: w291 -> [w294 _]
                  tunnel: w292 -> [w295 _]
                  tunnel: [w293 ""] -> w290
                  frame Default {
                    n177 = Index Array(array=w295, index=w294) -> (element=w293:string)
                  }
                  frame -1 {
                  }
                }
              }
            }
            n178 = for {
              tunnel: w281 -> [w304] mode=indexing
              tunnel: [w301] -> w285 mode=indexing
              n179 = call "Fast_string_Replace.vi"("Replace match with:"=" ", "Input String"=w304, "matchThis"=":" ("regular expression")) -> ("Output String"=w300:string)  [unwired: 1 in, 1 out]
              n180 = call "Fast_string_Replace.vi"("Replace match with:"=" ", "Input String"=w300, "matchThis"="  " ("regular expression")) -> ("Output String"=w299:string)  [unwired: 1 in, 1 out]
              n181 = call <vilib>:"Trim Whitespace.vi"("string"=w299) -> ("trimmed string"=w301:string)  [unwired: 1 in]
            }
          }
          frame True {
          }
        }
        n182 = global read "Results_plotter_Global.vi" "Load number"() -> (w255:i32)
        n183 = Increment(x=w255) -> (x+1=w254:i32)
        n184 = global write "Results_plotter_Global.vi" "Load number"(w254) -> ()
      }
      frame "Choose Results File(s)" {
        n185 = local read "Chosen Path"() -> (w313:path)
        n186 = call "File Dialog2"("start path"=w313, "prompt"="Please Choose a one or more Results Files" ("Promp if not found")) -> ("selected paths"=w311:path[], "cancelled"=w312:bool)  [unwired: 10 in, 2 out]
        n187 = case shown="False" w312 {
          tunnel: w311 -> [w322 _]
          frame False {
            n188 = local read "Result files to read"() -> (w323:path[])
            n189 = Index Array(array=w322) -> (element=w321:path)  [unwired: 1 in]
            n190 = Build Array (concatenate)(w323, w322) -> (w324:path[])
            n191 = Strip Path(path=w321) -> (stripped path=→"Chosen Path":path)  [unwired: 1 out]
            n192 = local write "Result files to read"(w324) -> ()
          }
          frame True {
          }
        }
      }
      frame "Choose a Folder" {
        n193 = local read "Chosen Path"() -> (w327:path)
        n194 = File Dialog(7:"Please Choose the folder that contains the Results files to be plotted" ("prompt"), 11:w327) -> (3:w326:path)  [unwired: 1 in, 7 out]
        n195 = call "Get_folder_and_filenames.vi"("file path (dialog if empty)"=w326) -> ("Files"=w328:path[])  [unwired: 1 out]
        n196 = for {
          shift-right: [w346] -> w329
          shift-left: "Result files to read" -> [w345]
          tunnel: w328 -> [w343] mode=indexing
          n197 = Search 1D Array(1D array=w345, element=w343) -> (index of element=w344:i32)  [unwired: 1 out]
          n198 = Strip Path(path=w343) -> (name=w342:string)  [unwired: 1 out]
          n199 = Less Than 0?(x=w344) -> (x < 0?=w341:bool)
          n200 = call "Add_filename_suffix.vi"("Filename"=w342) -> ("Original Suffix"=w339:string)  [unwired: 1 in, 3 out]
          n201 = call "Match_Pat_Case_In.vi"("String to match"=".jpg" ("x"), "String"=w339) -> ("offset past match"=w337:i32)  [unwired: 1 in, 3 out]
          n202 = Less Than 0?(x=w337) -> (x < 0?=w336:bool)
          n203 = And(x=w341, y=w336) -> (x .and. y?=w340:bool)
          n204 = case shown="True" w340 {
            tunnel: w345 -> [w347 w350]
            tunnel: w343 -> [_ w349]
            tunnel: [w347 w348] -> w346
            frame False {
            }
            frame True {
              n205 = Build Array (concatenate)(w350, w349) -> (w348:path[])
            }
          }
        }
        n206 = local write "Chosen Path"(w326) -> ()
        n207 = local write "Result files to read"(w329) -> ()
      }
      frame "Load Data" {
        n208 = local read "Result files to read"() -> (w360:path[])
        n209 = local read "File Index"() -> (w361:i32)
        n210 = Array Subset(array=w360, index=w361) -> (w373:path[])  [unwired: 1 in]
        n211 = for {
          tunnel: "Results files chosen" -> [w408]
          tunnel: w373 -> [w406] mode=indexing
          tunnel: [w406] -> w355 mode=indexing if=w405
          n212 = Search 1D Array(1D array=w408, element=w406) -> (index of element=w407:i32)  [unwired: 1 out]
          n213 = Less Than 0?(x=w407) -> (x < 0?=w405:bool)
        }
        n214 = Array Size(array=w367) -> (size(s)=w374:i32[])
        n215 = Index Array(array=w374, index=0 ("Index")) -> (element=w377:i32)
        n216 = Array Subset(array=w360, length=w361) -> (w359:path[])  [unwired: 1 in]
        n217 = Array Size(array=w355) -> (size(s)=w354:i32)
        n218 = Build Array (concatenate)("Results files chosen", w355) -> (w357:path[])
        n219 = Build Array (concatenate)(w359, w355) -> (w351:path[])
        n220 = Greater Than 0?(x=w354) -> (x > 0?=w356:bool)
        n221 = case shown="True" w356 {
          tunnel: w377 -> [_ w396]
          tunnel: "File Types to Read" -> [_ w392]
          tunnel: w367 -> [w380 w390]
          tunnel: [w382 w389] -> w366
          tunnel: [w381 w388] -> w365
          tunnel: [w380 w387] -> w364
          tunnel: w361 -> [_ w386]
          tunnel: w355 -> [_ w385]
          tunnel: w353 -> [w382 _]
          tunnel: w352 -> [w381 _]
          frame False {
          }
          frame True {
            n222 = local read "Template"() -> (w391:path)
            n223 = local read "Filetype"() -> (w384:string[])
            n224 = call "Load RFP Data FilesPLL.vi"("File Index"=w386, "Current Row Number"=w396, "Template"=w391, "Filetype In"=w384, "File Types to Read"=w392, "Files"=w385) -> ("Filetype Out"=→"Filetype":string[], "Channel Values Out"=w395:string[][], "Ch names Out"=w388:string[], "File Index Out"=w393:i32)  [unwired: 2 in]
            n225 = for {
              tunnel: w388 -> [w404] mode=indexing
              tunnel: [w401] -> w389 mode=indexing
              n226 = call "Fast_string_Replace.vi"("Replace match with:"=" ", "Input String"=w404, "matchThis"=":" ("regular expression")) -> ("Output String"=w400:string)  [unwired: 1 in, 1 out]
              n227 = call "Fast_string_Replace.vi"("Replace match with:"=" ", "Input String"=w400, "matchThis"="  " ("regular expression")) -> ("Output String"=w399:string)  [unwired: 1 in, 1 out]
              n228 = call <vilib>:"Trim Whitespace.vi"("string"=w399) -> ("trimmed string"=w401:string)  [unwired: 1 in]
            }
            n229 = Increment(x=w393) -> (x+1=w394:i32)
            n230 = Build Array (concatenate)(w390, w395) -> (w387:string[][])
            n231 = local write "File Index"(w394) -> ()
          }
        }
        n232 = local write "Results files chosen"(w357) -> ()
        n233 = global write "Results_plotter_Global.vi" "Results files Loaded"(w351) -> ()
        n234 = local write "Result files to read"(w351) -> ()
        n235 = Array Size(array=w364) -> (size(s)=w376:i32[])
        n236 = Index Array(array=w376, index=0 ("Index")) -> (element=w362:i32)
        "nRows" <- w362
        n237 = Greater Than 0?(x=w362) -> (x > 0?=w369:bool)
        n238 = local read "stop"() -> (w379:bool)
        n239 = Select(t="Remove Empty Channels", s=w369, f="What to do next?") -> (s? t:f=w363:string)
        n240 = Not(x=w379) -> (.not. x?=w378:bool)
      }
      frame "Remove Empty Channels" {
        n241 = Array Size(array=w412) -> (size(s)=w426:i32)
        n242 = Build Array (concatenate)("None" ("Input Element"), w410) -> (w409:string[])
        n243 = for {
          N: w426 -> [_]
          tunnel: w417 -> [w450]
          tunnel: [w447] -> w425 mode=indexing if=w446
          i -> [w447]
          n244 = Index Array(array=w450, index (col)=w447) -> (element=w449:string[])  [unwired: 1 in]
          n245 = Empty String/Path?(string/path=w449) -> (empty?=w448:bool[])
          n246 = And Array Elements(Boolean array=w448) -> (logical AND=w445:bool)
          n247 = Not(x=w445) -> (.not. x?=w446:bool)
        }
        n248 = property on="Wind Direction" class="Ring (strict)"("Strings []"=w409) -> ()  [unwired: 2 in, 2 out]
        n249 = property on="Z Ch Name" class="Ring (strict)"("Strings []"=w409) -> ()  [unwired: 2 in, 2 out]
        n250 = property on="X Ch Name" class="Ring (strict)"("Strings []"=w409) -> ()  [unwired: 2 in, 2 out]
        n251 = property on="Y Ch Name" class="Ring (strict)"("Strings []"=w409) -> ()  [unwired: 2 in, 2 out]
        n252 = property on="Coord System" class="Ring (strict)"("Strings []"=w409) -> ()  [unwired: 2 in, 2 out]
        n253 = property on="stl Filename" class="Ring (strict)"("Strings []"=w409) -> ()  [unwired: 2 in, 2 out]
        n254 = property on="U Ch Name" class="Ring (strict)"("Strings []"=w409) -> ()  [unwired: 2 in, 2 out]
        n255 = property on="V Ch Name" class="Ring (strict)"("Strings []"=w409) -> ()  [unwired: 2 in, 2 out]
        n256 = property on="W Ch Name" class="Ring (strict)"("Strings []"=w409) -> ()  [unwired: 2 in, 2 out]
        n257 = property on="Point ID" class="Ring (strict)"("Strings []"=w409) -> ()  [unwired: 2 in, 2 out]
        n258 = for {
          tunnel: w410 -> [w438]
          tunnel: [w437] -> w422 mode=indexing
          tunnel: w425 -> [w436] mode=indexing
          tunnel: w412 -> [w435]
          tunnel: [w434] -> w423 mode=indexing
          n259 = Index Array(array=w438, index=w436) -> (element=w437:string)
          n260 = Index Array(array=w435, index=w436) -> (element=w434:string)
        }
        n261 = for {
          tunnel: w417 -> [w441] mode=indexing
          tunnel: w425 -> [w440]
          tunnel: [w439] -> w416 mode=indexing
          n262 = for {
            tunnel: w441 -> [w443]
            tunnel: w440 -> [w444] mode=indexing
            tunnel: [w442] -> w439 mode=indexing
            n263 = Index Array(array=w443, index=w444) -> (element=w442:string)
          }
        }
        n264 = local read "Template"() -> (w414:path)
        n265 = global write "Results_plotter_Global.vi" "Channel names"(w422) -> ()
        n266 = global write "Results_plotter_Global.vi" "Full Ch Names"(w423) -> ()
        n267 = call "Load_Template_Globals.vi"("Non Blank Channels"=w425, "Template-read"=w414) -> ("Valid Template File?"=w420:bool)  [unwired: 1 in]
        n268 = global read "Results_plotter_Global.vi" "loadStartTime"() -> (w415:timestamp)
        n269 = Get Date/Time In Seconds() -> (seconds since 1Jan1904=w419:timestamp)
        n270 = case shown="True" w420 {
          tunnel: [w429 "Load Template File"] -> w421
          tunnel: [string[] [] ("Ch names Out") w432] -> w413
          tunnel: w412 -> [_ w432]
          frame False {
            n271 = local read "loadingSetup"() -> (w428:bool)
            n272 = Select(t="Update Selectors from File", s=w428, f="Update Selectors") -> (s? t:f=w429:string)
          }
          frame True {
          }
        }
        n273 = Subtract(x=w419, y=w415) -> (x-y=→"loadTime(s)":dbl)
        n274 = global write "Results_plotter_Global.vi" "All Template Ch Names"(w413) -> ()
      }
      frame "Load Template File" {
        n275 = global read "Results_plotter_Global.vi" "All Template Ch Names"() -> (w453:string[])
        n276 = local read "Template"() -> (w457:path)
        n277 = for {
          tunnel: w457 -> [w490]
          tunnel: Global_mode."Read Global" ("Mode") -> [w489]
          tunnel: w458 -> [w488] mode=indexing
          tunnel: [w487] -> w460 mode=indexing
          tunnel: [w486] -> w455
          n278 = call "Read_Write_Template.vi"("Template File"=w490, "Mode"=w489, "Data type"=w488) -> ("Template File Out"=w486:path, "Single Value Out"=w487:string)  [unwired: 5 in, 6 out]
        }
        "Template Single Values" <- w460
        n279 = Build Array (concatenate)("None", w453) -> (w452:string[])
        n280 = global write "Results_plotter_Global.vi" "Template"(w455) -> ()
        n281 = for {
          tunnel: w452 -> [w470]
          tunnel: w460 -> [w468] mode=indexing
          i -> [w469]
          n282 = Search 1D Array(1D array=w470, element=w468) -> (index of element=w473:i32)  [unwired: 1 in]
          n283 = Greater Or Equal To 0?(x=w473) -> (x >= 0?=w474:bool)
          n284 = Select(t=w473, s=w474, f=0) -> (s? t:f=w472:i32)
          n285 = case shown="9" w469 {
            tunnel: w472 -> [w475 w476 w477 w478 w479 w480 w481 w482 w483 _]
            tunnel: w468 -> [_ _ _ _ _ _ _ _ _ w484]
            frame 0, Default {
              n286 = local write "X Ch Name"(w475) -> ()
            }
            frame 1 {
              n287 = local write "Y Ch Name"(w476) -> ()
            }
            frame 2 {
              n288 = local write "Z Ch Name"(w477) -> ()
            }
            frame 3 {
              n289 = local write "Wind Direction"(w478) -> ()
            }
            frame 4 {
              n290 = local write "Coord System"(w479) -> ()
            }
            frame 5 {
              n291 = local write "stl Filename"(w480) -> ()
            }
            frame 6 {
              n292 = local write "U Ch Name"(w481) -> ()
            }
            frame 7 {
              n293 = local write "V Ch Name"(w482) -> ()
            }
            frame 8 {
              n294 = local write "W Ch Name"(w483) -> ()
            }
            frame 9 {
              n295 = call "String_to_Pathname.vi"("Input String"=w484) -> ("path"=w485:path)
              n296 = local write "Job Directory"(w485) -> ()
            }
          }
        }
        n297 = global read "Results_plotter_Global.vi" "Tolerances"() -> (→"Tolerances":dbl[])
        n298 = local read "loadingSetup"() -> (w462:bool)
        n299 = Select(t="Update Selectors from File", s=w462, f="Update Selectors") -> (s? t:f=w466:string)
      }
      frame "Update Selectors from File" {
        n300 = local read "importingSetup"() -> (w492:bool)
        n301 = case shown="False" w492 {
          tunnel: w498 -> [w502 _]
          tunnel: [w501 "Load Selectors"] -> w495
          tunnel: w493 -> [w500 _]
          tunnel: [FALSE ("Save Setup") FALSE ("Save Setup")] -> w491
          frame False {
            n302 = global read "Results_plotter_Global.vi" "Setup Filename"() -> (w506:string)
            n303 = call "Read_Write_Plot_Setup.vi"("Mode"=enum16{"Load", "Save"}."Load", "Setup filename"=w506) -> ("OK?"=w504:bool, "Cluster 2"=w503:T17)  [unwired: 7 in, 1 out]
            n304 = case shown="True" w504 {
              tunnel: w503 -> [_ w510]
              tunnel: w502 -> [_ w511]
              tunnel: ["Update Selectors" w509] -> w501
              tunnel: w500 -> [_ w508]
              frame False {
              }
              frame True {
                n305 = stacked-sequence {
                  seq-local: [w514 _] -> [_ w534]
                  tunnel: w511 -> [w513 _]
                  tunnel: w510 -> [w515 w537]
                  tunnel: [_ "Load Selectors"] -> w509
                  tunnel: w508 -> [w512 _]
                  frame #0 {
                    n306 = Unbundle By Name(w515) -> ("Multi Ordinate"=w517:string[], "Abscissa String"=w516:string)
                    n307 = for {
                      tunnel: w513 -> [w528]
                      tunnel: [w524] -> w518 mode=indexing
                      tunnel: w517 -> [w523] mode=indexing
                      n308 = Search 1D Array(1D array=w528, element=w523) -> (index of element=w526:i32)  [unwired: 1 in]
                      n309 = Greater Or Equal To 0?(x=w526) -> (x >= 0?=w527:bool)
                      n310 = Select(t=w526, s=w527, f=0) -> (s? t:f=w524:i32)
                    }
                    n311 = Search 1D Array(1D array=w513, element=w516) -> (index of element=w521:i32)  [unwired: 1 in]
                    n312 = Greater Or Equal To 0?(x=w521) -> (x >= 0?=w522:bool)
                    n313 = Build Array (concatenate)(w512, w513) -> (w514:string[])
                    n314 = Select(t=w521, s=w522, f=0) -> (s? t:f=w519:i32)
                    n315 = local write "Absisca"(w519) -> ()
                    n316 = local write "Multi Ordinate"(w518) -> ()
                  }
                  frame #1 {
                    # "Offset for fixed first elements"
                    # "To prevent erroneous numbers of filters being loaded.\nLimited to 6, as only 6 are handled in selector case"
                    n317 = Unbundle By Name(w537) -> ("Filter Array"=w535:string[], "Filter Bins 1 Strings"=w531:string[], "Filter Bins 2 Strings"=w530:string[], "Filters 3 onwards"=w529:string[])
                    n318 = local write "Filter Bins 1 Strings"(w531) -> ()
                    n319 = local write "Filter Bins 2 Strings"(w530) -> ()
                    n320 = local write "Filters 3 onwards"(w529) -> ()
                    n321 = for {
                      N: 6 -> [_]
                      tunnel: [w540] -> w536 mode=indexing
                      tunnel: w535 -> [w539] mode=indexing
                      tunnel: w534 -> [w538]
                      n322 = Search 1D Array(1D array=w538, element=w539) -> (index of element=w542:i32)  [unwired: 1 in]
                      n323 = Greater Or Equal To 0?(x=w542) -> (x >= 0?=w543:bool)
                      n324 = Select(t=w542, s=w543, f=0) -> (s? t:f=w540:i32)
                    }
                    n325 = local write "Filter Array"(w536) -> ()
                  }
                }
              }
            }
          }
          frame True {
            n326 = local read "setupOrINI"() -> (w547:path)
            n327 = control-ref of="This VI"() -> (w546:refnum<vi>)
            n328 = call "INI-FP.vi"("Mode"=enum16{"Read", "Write"}."Read", "prompt"="", "VIreference"=w546, "INIfilepathIn"=w547) -> ()  [unwired: 6 in, 2 out]
          }
        }
        n329 = local write "loadingSetup"(w491) -> ()
        n330 = local write "importingSetup"(w491) -> ()
      }
      frame "Update Selectors" {
        n331 = Array Size(array=w552) -> (size(s)=w553:i32)
        n332 = property on="Absisca" class="Ring (strict)"() -> ("Strings []"=w551:string[])  [unwired: 2 in, 2 out]
        n333 = local read "Absisca"() -> (w554:u16)
        n334 = local read "Multi Ordinate"() -> (w567:i32[])
        n335 = local read "Filter Array"() -> (w564:u16[])
        n336 = Build Array (concatenate)(w550, w552) -> (w561:string[])
        n337 = Build Array (concatenate)(w550, w551) -> (w565:string[])
        n338 = Increment(x=w553) -> (x+1=w560:i32)
        n339 = Index Array(array=w551, index=w554) -> (element=w556:string)
        n340 = Search 1D Array(1D array=w552, element=w556) -> (index of element=w557:i32)  [unwired: 1 in]
        n341 = for {
          tunnel: w567 -> [w592] mode=indexing
          tunnel: [w590] -> w566 mode=indexing if=w591
          tunnel: w551 -> [w589]
          tunnel: w552 -> [w588]
          n342 = Index Array(array=w589, index=w592) -> (element=w593:string)
          n343 = Search 1D Array(1D array=w588, element=w593) -> (index of element=w590:i32)  [unwired: 1 in]
          n344 = Greater Or Equal To 0?(x=w590) -> (x >= 0?=w591:bool)
        }
        n345 = for {
          tunnel: w565 -> [w580]
          tunnel: w561 -> [w579]
          tunnel: w564 -> [w575] mode=indexing
          tunnel: [w578] -> w563 mode=indexing
          tunnel: w560 -> [w576]
          n346 = Index Array(array=w580, index=w575) -> (element=w581:string)
          n347 = Search 1D Array(1D array=w579, element=w581) -> (index of element=w577:i32)  [unwired: 1 in]
          n348 = case shown="Default" w577 {
            selector: w577 -> [w582 _]
            tunnel: [w582 w587] -> w578
            tunnel: w575 -> [_ w584]
            tunnel: w576 -> [_ w585]
            frame Default {
            }
            frame -1 {
              n349 = Less?(x=w584, y=w585) -> (x < y?=w586:bool)
              n350 = Select(t=w584, s=w586, f=0) -> (s? t:f=w587:i32)
            }
          }
        }
        n351 = case shown="-1" w557 {
          selector: w557 -> [w569 _]
          tunnel: [w569 w574] -> w555
          tunnel: w554 -> [_ w571]
          tunnel: w553 -> [_ w572]
          frame Default {
          }
          frame -1 {
            n352 = Less?(x=w571, y=w572) -> (x < y?=w573:bool)
            n353 = Select(t=w571, s=w573, f=0) -> (s? t:f=w574:i32)
          }
        }
        n354 = local write "Absisca"(w555) -> ()
        n355 = local write "Multi Ordinate"(w566) -> ()
        n356 = local write "Filter Array"(w563) -> ()
      }
      frame "Load Selectors" {
        n357 = Build Array (concatenate)(w595, w597) -> (w607:string[])
        n358 = local read "Tolerances"() -> (w603:dbl[])
        n359 = Search 1D Array(1D array=w600, element="Raw:Data:Filename") -> (index of element=w598:i32)  [unwired: 1 in]
        n360 = global write "Results_plotter_Global.vi" "Raw Data Filename index"(w598) -> ()
        n361 = property on="Filter on column 1:" class="Ring (strict)"("Strings []"=w607) -> ()  [unwired: 2 in, 2 out]
        n362 = property on="Multi Ordinate" class="LstBox (strict)"("Item Names"=w597) -> ()  [unwired: 2 in, 2 out]
        n363 = property on="Absisca" class="Ring (strict)"("Strings []"=w597) -> ()  [unwired: 2 in, 2 out]
        n364 = Array Size(array=w597) -> (size(s)=w605:i32)
        n365 = Array Size(array=w603) -> (size(s)=w604:i32)
        n366 = Not Equal?(x=w605, y=w604) -> (x != y?=w606:bool)
        n367 = case shown="True" w606 {
          tunnel: w605 -> [_ w615]
          tunnel: w604 -> [_ w614]
          tunnel: w603 -> [_ w611]
          frame False {
          }
          frame True {
            n368 = Subtract(x=w615, y=w614) -> (x-y=w613:i32)
            n369 = Initialize Array(1.0 ("Element Data"), w613) -> (w610:dbl[])
            n370 = Build Array (concatenate)(w611, w610) -> (w609:dbl[])
            n371 = local write "Tolerances"(w609) -> ()
          }
        }
        n372 = local write "Reload Files"(FALSE ("Reload Files")) -> ()
        n373 = global write "Results_plotter_Global.vi" "First Loop"(TRUE) -> ()
      }
      frame "Perform Global Concatenate" {
        n374 = global read "Results_plotter_Global.vi" "Maths"() -> (w623:string[])
        n375 = for {
          tunnel: w623 -> [w630] mode=indexing
          tunnel: "Concatenate" ("regular expression") -> [w632]
          tunnel: w621 -> [w629]
          shift-right: [w626] -> w616
          shift-left: w617 -> [w627]
          i -> [w628]
          n376 = Match Pattern(string=w630, regular expression=w632) -> (offset past match=w631:i32)  [unwired: 1 in, 3 out]
          n377 = case shown="Default" w631 {
            tunnel: w630 -> [w637 _]
            tunnel: w629 -> [w636 _]
            tunnel: w628 -> [w635 _]
            tunnel: w627 -> [w634 w638]
            tunnel: [w633 w638] -> w626
            frame Default {
              n378 = call "RFP_Concatenate.vi"("Output Index"=w635, "Channel Values In"=w634, "Channel Names"=w636, "Maths Equation"=w637) -> ("Channel Values Out"=w633:string[][])  [unwired: 2 in, 1 out]
            }
            frame -1 {
            }
          }
        }
        n379 = local read "Template"() -> (w619:path)
        n380 = File/Directory Info(path=w619) -> (last mod=→"Template Last Mod":timestamp)  [unwired: 1 in, 6 out]
      }
      frame "What is present?" {
        n381 = case shown="True" "Show Results Space Analysis" {
          tunnel: w643 -> [_ w647]
          tunnel: w639 -> [_ w646]
          frame False {
          }
          frame True {
            n382 = stacked-sequence {
              tunnel: w647 -> [w651]
              tunnel: w646 -> [w648]
              frame #0 {
                w649 = FALSE  # Summarise All
                n383 = call "Summarise.vi"("Channel Names"=w651, "Data"=w648, "Summarise All"=w649) -> ("Summary"=w650:string[][])  [unwired: 2 in]
                n384 = call "Results_Space_Analysis.vi"("Table"=w650) -> ()
              }
            }
          }
        }
        n385 = global write "Results_plotter_Global.vi" "New Values Row index"(i32[] [] ("New Values Row Number")) -> ()
      }
      frame "Ordinate Selector Type" {
        w655 = "Raw:Data:Filename" ("element")
        w659 = TRUE ("element")
        n386 = global read "Results_plotter_Global.vi" "All Template Ch Names"() -> (w657:string[])
        n387 = Build Array("Xon", "Yon", "Zon", w659, w659, w659, "Uon", "Von", "Won", w659) -> (w662:bool[])
        n388 = Build Array("X Ch Name", "Y Ch Name", "Z Ch Name", "Wind Direction", "Coord System", "stl Filename", "U Ch Name", "V Ch Name", "W Ch Name", "Point ID") -> (w675:u16[])
        n389 = Boolean To (0,1)(Boolean=w662) -> (0, 1=w660:i16[])
        n390 = Multiply(x=w675, y=w660) -> (x*y=w661:u16[])
        n391 = for {
          tunnel: w657 -> [w689]
          tunnel: [w687] -> w682 mode=indexing
          tunnel: w661 -> [w685] mode=indexing
          tunnel: w654 -> [w688]
          tunnel: [w686] -> w676 mode=indexing
          n392 = case shown="Default" w685 {
            selector: w685 -> [_ w692]
            tunnel: w689 -> [_ w697]
            tunnel: w688 -> [_ w696]
            tunnel: ["None" ("X Ch Name String") w695] -> w687
            tunnel: [-1 ("index of element") w694] -> w686
            frame 0 {
            }
            frame Default {
              n393 = Decrement(x=w692) -> (x-1=w693:u16)
              n394 = Index Array(array=w697, index=w693) -> (element=w695:string)
              n395 = Search 1D Array(1D array=w696, element=w695) -> (index of element=w694:i32)  [unwired: 1 in]
            }
          }
        }
        n396 = Search 1D Array(1D array=w654, element=w655) -> (index of element=w652:i32)  [unwired: 1 in]
        n397 = Build Array (concatenate)(w682, w655) -> (w656:string[])
        n398 = Build Array (concatenate)(w676, w652) -> (w653:i32[])
        n399 = global write "Results_plotter_Global.vi" "3D Ch Names"(w656) -> ()
        n400 = global write "Results_plotter_Global.vi" "3D Ch Selectors"(w653) -> ()
      }
      frame "Which rows are Non-Blank?" {
        n401 = while {
          tunnel: [w717] -> w712
          tunnel: [w718] -> w713
          shift-left: _ -> [w719]
          shift-right: [w720] -> w706
          shift-left: _ -> [w722]
          shift-right: [w721] -> _
          stop <- FALSE continue-if-true
          n402 = local read "Multi Ordinate"() -> (w720:i32[])
          n403 = local read "Absisca"() -> (w721:u16)
          n404 = Equal?(x=w721, y=w722) -> (x = y?=w718:bool)
          n405 = Equal?(x=w720, y=w719) -> (x = y?=w717:bool)
        }
        n406 = global read "Results_plotter_Global.vi" "First Loop"() -> (w708:bool)
        n407 = Compound Arithmetic op=AND(invert w708, w713, w712) -> (w711:bool)
        n408 = Array Size(array=w706) -> (size(s)=w705:i32)
        n409 = Greater?(x=w705, y=1) -> (0:w703:bool)
        n410 = global write "Results_plotter_Global.vi" "Multi Ordinate?"(w703) -> ()
        n411 = local read "Edit Template File"() -> (w701:bool)
        n412 = Select(t="Create Selectors", s=w711, f="Evaluate Blank Rows") -> (s? t:f=w699:string)
        n413 = Select(t="Edit template file", s=w701, f=w699) -> (s? t:f=w698:string)
      }
      frame "Evaluate Blank Rows" {
        n414 = local read "Multi Ordinate"() -> (w726:i32[])
        n415 = local read "Absisca"() -> (w727:u16)
        n416 = for {
          tunnel: w724 -> [w732] mode=indexing
          tunnel: w727 -> [w735]
          tunnel: w726 -> [w734]
          tunnel: [w731] -> w725 mode=indexing
          n417 = Index Array(array=w732, index=w735) -> (element=w736:string)
          n418 = call "Convert_to_number.vi"("string"=w736) -> ("Number"=w737:dbl)  [unwired: 1 out]
          n419 = Not A Number/Path/Refnum?(number/path/refnum=w737) -> (NaN/Path/Refnum?=w733:bool)
          n420 = case shown="False" w733 {
            tunnel: w734 -> [w741 _]
            tunnel: w732 -> [w740 _]
            tunnel: [w738 FALSE] -> w731
            frame False {
              n421 = for {
                tunnel: w741 -> [w747] mode=indexing
                tunnel: w740 -> [w745]
                tunnel: [w742] -> w739 mode=indexing
                n422 = Index Array(array=w745, index=w747) -> (element=w746:string)
                n423 = call "Convert_to_number.vi"("string"=w746) -> ("Number"=w744:dbl)  [unwired: 1 out]
                n424 = Not A Number/Path/Refnum?(number/path/refnum=w744) -> (NaN/Path/Refnum?=w743:bool)
                n425 = Not(x=w743) -> (.not. x?=w742:bool)
              }
              n426 = Or Array Elements(Boolean array=w739) -> (logical OR=w738:bool)
            }
            frame True {
            }
          }
        }
        "Non-Blank Rows" <- w725
      }
      frame "Create Selectors" {
        n427 = local read "Non-Blank Rows"() -> (w768:bool[])
        n428 = local read "Tolerances"() -> (w766:dbl[])
        n429 = Array Size(array=w752) -> (size(s)=w771:i32[])
        n430 = global read "Results_plotter_Global.vi" "Precision"() -> (w765:string[])
        n431 = Index Array(array=w771, index=0 ("Index")) -> (element=w773:i32)
        n432 = while {
          shift-right: [w778] -> w755
          shift-left: _ -> [_]
          shift-left: _ -> [w777]
          tunnel: w759 -> [w778]
          tunnel: [w777] -> w758
          stop <- TRUE stop-if-true
        }
        n433 = global read "Results_plotter_Global.vi" "First Loop"() -> (w762:bool)
        n434 = for {
          tunnel: w752 -> [w795]
          tunnel: "Filter Array" -> [w783] mode=indexing
          shift-right: [w794] -> w767
          shift-left: _ -> [w792]
          tunnel: w773 -> [w793]
          tunnel: [w790] -> w769 mode=indexing
          tunnel: w768 -> [w789]
          tunnel: w766 -> [w788]
          tunnel: w765 -> [w786]
          tunnel: w762 -> [w784]
          tunnel: "notSelectors?" -> [w780]
          i -> [w791]
          n435 = Subtract(x=w783, y=u16 2) -> (x-y=w782:u16)
          n436 = Index Array(array=w788, index=w782) -> (element=w787:dbl)
          n437 = Index Array(array=w786, index=w782) -> (element=w785:string)
          n438 = case shown="6, Default" w791 {
            selector: w791 -> [w797 w837 w885 w933 w979 w1027 _]
            tunnel: w795 -> [w811 w852 w897 w944 w991 w1041 _]
            tunnel: w783 -> [w810 w851 w896 w932 w990 w1026 _]
            tunnel: w787 -> [w809 w850 w895 w943 w989 w1040 _]
            tunnel: [w808 w849 w894 w942 w988 w1039 w1074] -> w794
            tunnel: w793 -> [w806 w848 w893 w941 w987 w1038 _]
            tunnel: w792 -> [_ w847 w892 w940 w986 w1037 w1074]
            tunnel: [w803 w843 w889 w937 w983 w1033 TRUE ("Unchanged?")] -> w790
            tunnel: w789 -> [w802 w842 w888 w936 w982 w1032 _]
            tunnel: w785 -> [w801 w841 w887 w935 w981 w1031 _]
            tunnel: w784 -> [w799 w839 w886 w934 w980 w1028 _]
            tunnel: w780 -> [w796 w836 w884 w931 w978 w1025 _]
            frame 0 {
              n439 = case shown="0" w810 {
                selector: w810 -> [w814 w825]
                tunnel: w811 -> [w819 w829]
                tunnel: w809 -> [_ w835]
                tunnel: [w815 w832] -> w808
                tunnel: "Filter Bins 1" -> [_ w833]
                tunnel: [string[] [] ("Write Attribute") w834] -> w807
                tunnel: w806 -> [w817 _]
                tunnel: w797 -> [w822 w831]
                tunnel: [i32[] [0] ("Filter Bins Out") w830] -> w804
                tunnel: [TRUE ("Unchanged?") w828] -> w803
                tunnel: w802 -> [_ w827]
                tunnel: w801 -> [_ w826]
                tunnel: w796 -> [w813 w824]
                frame 0 {
                  n440 = call "Create_filter_points.vi"("notSelectors?"=w813, "Index"=w822, "Channel to Filter On"=w814, "Ch Values In"=w819) -> ()  [unwired: 4 in, 4 out]
                  n441 = Initialize Array(TRUE, w817) -> (w816:bool[])
                  n442 = Build Array(w816) -> (w815:bool[][])
                }
                frame 1, Default {
                  n443 = call "Create_filter_points.vi"("Precision"=w826, "Non-Blank Rows"=w827, "notSelectors?"=w824, "Index"=w831, "Channel to Filter On"=w825, "Tolerance"=w835, "Filter Bins 1"=w833, "Ch Values In"=w829) -> ("Unchanged?"=w828:bool, "Accept array"=w832:bool[][], "Filter Bins Out"=w830:i32[], "Bin Names"=w834:string[])
                }
              }
              n444 = Equal?(x="Filter Bins 1", y=w804) -> (x = y?=w800:bool)
              n445 = Or(x=w799, y=w800) -> (x .or. y?=w798:bool)
              n446 = case shown="False" w798 {
                tunnel: w804 -> [w812 _]
                frame False {
                  n447 = local write "Filter Bins 1"(w812) -> ()
                }
                frame True {
                }
              }
              n448 = property on="Filter bins 1" class="LstBox (strict)"("Item Names"=w807) -> ()  [unwired: 2 in, 2 out]
            }
            frame 1 {
              n449 = case shown="1, Default" w851 {
                tunnel: w852 -> [_ w866]
                tunnel: w851 -> [w856 w865]
                tunnel: w850 -> [_ w873]
                tunnel: [w860 w869] -> w849
                tunnel: "Filter Bins 2" -> [_ w871]
                tunnel: [string[] [] ("Write Attribute") w875] -> w846
                tunnel: w848 -> [_ _]
                tunnel: w847 -> [w860 w874]
                tunnel: w837 -> [w859 w872]
                tunnel: [i32[] [0] ("Filter Bins Out") w867] -> w845
                tunnel: [TRUE ("Unchanged?") w864] -> w843
                tunnel: w842 -> [_ w863]
                tunnel: w841 -> [_ w862]
                tunnel: w836 -> [w854 w861]
                frame 0 {
                  n450 = call "Create_filter_points.vi"("notSelectors?"=w854, "Index"=w859, "Channel to Filter On"=w856) -> ()  [unwired: 5 in, 4 out]
                }
                frame 1, Default {
                  n451 = call "Create_filter_points.vi"("Precision"=w862, "Non-Blank Rows"=w863, "notSelectors?"=w861, "Index"=w872, "Channel to Filter On"=w865, "Tolerance"=w873, "Filter Bins 1"=w871, "Ch Values In"=w866) -> ("Unchanged?"=w864:bool, "Accept array"=w870:bool[][], "Filter Bins Out"=w867:i32[], "Bin Names"=w875:string[])
                  n452 = for {
                    tunnel: w874 -> [w880]
                    tunnel: w870 -> [w879] mode=indexing
                    shift-right: [w876] -> w869
                    shift-left: bool[][] [] -> [w878]
                    n453 = for {
                      tunnel: w879 -> [w883]
                      tunnel: w880 -> [w882] mode=indexing
                      tunnel: [w881] -> _ mode=indexing
                      tunnel: [w881] -> w877 mode=indexing
                      n454 = And(x=w883, y=w882) -> (x .and. y?=w881:bool[])
                    }
                    n455 = Build Array (concatenate)(w878, w877) -> (w876:bool[][])
                  }
                }
              }
              n456 = Equal?(x="Filter Bins 2", y=w845) -> (x = y?=w840:bool)
              n457 = Or(x=w839, y=w840) -> (x .or. y?=w838:bool)
              n458 = case shown="True" w838 {
                tunnel: w845 -> [w853 _]
                frame False {
                  n459 = local write "Filter Bins 2"(w853) -> ()
                }
                frame True {
                }
              }
              n460 = property on="Filter Bins 2" class="LstBox (strict)"("Item Names"=w846) -> ()  [unwired: 2 in, 2 out]
            }
            frame 2 {
              n461 = case shown="0" w896 {
                selector: w896 -> [w899 w906]
                tunnel: w897 -> [_ w913]
                tunnel: w895 -> [_ w923]
                tunnel: [w904 w924] -> w894
                tunnel: "Filter 3" -> [_ w915]
                tunnel: [string[] [] ("Write Attribute") w926] -> w890
                tunnel: w893 -> [_ _]
                tunnel: w892 -> [w904 w925]
                tunnel: w885 -> [w903 w918]
                tunnel: [TRUE ("Unchanged?") w912] -> w889
                tunnel: w888 -> [_ w911]
                tunnel: w887 -> [_ w910]
                tunnel: w886 -> [_ w907]
                tunnel: w884 -> [w898 w905]
                frame 0 {
                  n462 = call "Create_filter_points.vi"("notSelectors?"=w898, "Index"=w903, "Channel to Filter On"=w899) -> ()  [unwired: 5 in, 4 out]
                  n463 = local write "Filter 3"(0) -> ()
                }
                frame 1, Default {
                  n464 = Build Array(w915) -> (w922:u16[])
                  n465 = call "Create_filter_points.vi"("Precision"=w910, "Non-Blank Rows"=w911, "notSelectors?"=w905, "Index"=w918, "Channel to Filter On"=w906, "Tolerance"=w923, "Filter Bins 1"=w922, "Ch Values In"=w913) -> ("Unchanged?"=w912:bool, "Accept array"=w920:bool[][], "Filter Bins Out"=w916:i32[], "Bin Names"=w926:string[])
                  n466 = Index Array(array=w916, index=0 ("Index")) -> (element=w914:i32)
                  n467 = Equal?(x=w915, y=w914) -> (x = y?=w909:bool)
                  n468 = Index Array(array=w920, index (row)=0 ("Index")) -> (element=w919:bool[])  [unwired: 1 in]
                  n469 = Or(x=w907, y=w909) -> (x .or. y?=w908:bool)
                  n470 = case shown="False" w908 {
                    tunnel: w914 -> [w927 _]
                    frame False {
                      n471 = local write "Filter 3"(w927) -> ()
                    }
                    frame True {
                    }
                  }
                  n472 = for {
                    tunnel: w919 -> [w930]
                    tunnel: w925 -> [w929] mode=indexing
                    tunnel: [w928] -> w924 mode=indexing
                    n473 = And(x=w930, y=w929) -> (x .and. y?=w928:bool[])
                  }
                }
              }
              n474 = property on="Filter 3" class="Ring (strict)"("Strings []"=w890) -> ()  [unwired: 2 in, 2 out]
            }
            frame 3 {
              n475 = case shown="0" w932 {
                selector: w932 -> [w946 w953]
                tunnel: w944 -> [_ w960]
                tunnel: w943 -> [_ w970]
                tunnel: [w951 w971] -> w942
                tunnel: "Filter 4" -> [_ w962]
                tunnel: [string[] [] ("Write Attribute") w973] -> w938
                tunnel: w941 -> [_ _]
                tunnel: w940 -> [w951 w972]
                tunnel: w933 -> [w950 w965]
                tunnel: [TRUE ("Unchanged?") w959] -> w937
                tunnel: w936 -> [_ w958]
                tunnel: w935 -> [_ w957]
                tunnel: w934 -> [_ w955]
                tunnel: w931 -> [w945 w952]
                frame 0 {
                  n476 = call "Create_filter_points.vi"("notSelectors?"=w945, "Index"=w950, "Channel to Filter On"=w946) -> ()  [unwired: 5 in, 4 out]
                  n477 = local write "Filter 4"(0) -> ()
                }
                frame 1, Default {
                  n478 = Build Array(w962) -> (w969:u16[])
                  n479 = call "Create_filter_points.vi"("Precision"=w957, "Non-Blank Rows"=w958, "notSelectors?"=w952, "Index"=w965, "Channel to Filter On"=w953, "Tolerance"=w970, "Filter Bins 1"=w969, "Ch Values In"=w960) -> ("Unchanged?"=w959:bool, "Accept array"=w967:bool[][], "Filter Bins Out"=w963:i32[], "Bin Names"=w973:string[])
                  n480 = Index Array(array=w963, index=0 ("Index")) -> (element=w961:i32)
                  n481 = Equal?(x=w962, y=w961) -> (x = y?=w956:bool)
                  n482 = Index Array(array=w967, index (row)=0 ("Index")) -> (element=w966:bool[])  [unwired: 1 in]
                  n483 = Or(x=w955, y=w956) -> (x .or. y?=w954:bool)
                  n484 = case shown="False" w954 {
                    tunnel: w961 -> [w974 _]
                    frame False {
                      n485 = local write "Filter 4"(w974) -> ()
                    }
                    frame True {
                    }
                  }
                  n486 = for {
                    tunnel: w966 -> [w977]
                    tunnel: w972 -> [w976] mode=indexing
                    tunnel: [w975] -> w971 mode=indexing
                    n487 = And(x=w977, y=w976) -> (x .and. y?=w975:bool[])
                  }
                }
              }
              n488 = property on="Filter 4" class="Ring (strict)"("Strings []"=w938) -> ()  [unwired: 2 in, 2 out]
            }
            frame 4 {
              n489 = case shown="1, Default" w990 {
                selector: w990 -> [w993 w1000]
                tunnel: w991 -> [_ w1007]
                tunnel: w989 -> [_ w1017]
                tunnel: [w998 w1018] -> w988
                tunnel: "Filter 5" -> [_ w1008]
                tunnel: [string[] [] ("Write Attribute") w1020] -> w984
                tunnel: w987 -> [_ _]
                tunnel: w986 -> [w998 w1019]
                tunnel: w979 -> [w997 w1012]
                tunnel: [TRUE ("Unchanged?") w1006] -> w983
                tunnel: w982 -> [_ w1005]
                tunnel: w981 -> [_ w1004]
                tunnel: w980 -> [_ w1001]
                tunnel: w978 -> [w992 w999]
                frame 0 {
                  n490 = call "Create_filter_points.vi"("notSelectors?"=w992, "Index"=w997, "Channel to Filter On"=w993) -> ()  [unwired: 5 in, 4 out]
                  n491 = local write "Filter 5"(0) -> ()
                }
                frame 1, Default {
                  n492 = Build Array(w1008) -> (w1016:u16[])
                  n493 = call "Create_filter_points.vi"("Precision"=w1004, "Non-Blank Rows"=w1005, "notSelectors?"=w999, "Index"=w1012, "Channel to Filter On"=w1000, "Tolerance"=w1017, "Filter Bins 1"=w1016, "Ch Values In"=w1007) -> ("Unchanged?"=w1006:bool, "Accept array"=w1014:bool[][], "Filter Bins Out"=w1010:i32[], "Bin Names"=w1020:string[])
                  n494 = Index Array(array=w1010, index=0 ("Index")) -> (element=w1009:i32)
                  n495 = Equal?(x=w1008, y=w1009) -> (x = y?=w1003:bool)
                  n496 = Index Array(array=w1014, index (row)=0 ("Index")) -> (element=w1013:bool[])  [unwired: 1 in]
                  n497 = Or(x=w1001, y=w1003) -> (x .or. y?=w1002:bool)
                  n498 = case shown="False" w1002 {
                    tunnel: w1009 -> [w1021 _]
                    frame False {
                      n499 = local write "Filter 5"(w1021) -> ()
                    }
                    frame True {
                    }
                  }
                  n500 = for {
                    tunnel: w1013 -> [w1024]
                    tunnel: w1019 -> [w1023] mode=indexing
                    tunnel: [w1022] -> w1018 mode=indexing
                    n501 = And(x=w1024, y=w1023) -> (x .and. y?=w1022:bool[])
                  }
                }
              }
              n502 = property on="Filter 5" class="Ring (strict)"("Strings []"=w984) -> ()  [unwired: 2 in, 2 out]
            }
            frame 5 {
              n503 = case shown="0" w1026 {
                selector: w1026 -> [w1044 w1051]
                tunnel: w1041 -> [_ w1060]
                tunnel: w1040 -> [_ w1064]
                tunnel: [w1049 w1052] -> w1039
                tunnel: "Single Series" -> [_ w1062]
                tunnel: [string[] [] ("Write Attribute") w1066] -> w1036
                tunnel: w1038 -> [_ _]
                tunnel: w1037 -> [w1049 w1065]
                tunnel: w1027 -> [w1048 w1063]
                tunnel: [i32[] [0] ("Filter Bins Out") w1061] -> w1035
                tunnel: [TRUE ("Unchanged?") w1059] -> w1033
                tunnel: w1032 -> [_ w1058]
                tunnel: w1031 -> [_ w1057]
                tunnel: w1025 -> [w1043 w1050]
                frame 0 {
                  n504 = call "Create_filter_points.vi"("notSelectors?"=w1043, "Index"=w1048, "Channel to Filter On"=w1044) -> ()  [unwired: 5 in, 4 out]
                }
                frame 1, Default {
                  n505 = call "Create_filter_points.vi"("Precision"=w1057, "Non-Blank Rows"=w1058, "notSelectors?"=w1050, "Index"=w1063, "Channel to Filter On"=w1051, "Tolerance"=w1064, "Filter Bins 1"=w1062, "Ch Values In"=w1060) -> ("Unchanged?"=w1059:bool, "Accept array"=w1054:bool[][], "Filter Bins Out"=w1061:i32[], "Bin Names"=w1066:string[])
                  n506 = Index Array(array=w1054, index (row)=0 ("Index")) -> (element=w1055:bool[])  [unwired: 1 in]
                  n507 = for {
                    shift-right: [w1067] -> w1053
                    shift-left: w1055 -> [w1069]
                    tunnel: w1054 -> [w1068] mode=indexing
                    n508 = Or(x=w1068, y=w1069) -> (x .or. y?=w1067:bool[])
                  }
                  n509 = for {
                    tunnel: w1053 -> [w1072]
                    tunnel: w1065 -> [w1071] mode=indexing
                    tunnel: [w1070] -> w1052 mode=indexing
                    n510 = And(x=w1072, y=w1071) -> (x .and. y?=w1070:bool[])
                  }
                }
              }
              n511 = Equal?(x="Single Series", y=w1035) -> (x = y?=w1030:bool)
              n512 = Or(x=w1028, y=w1030) -> (x .or. y?=w1029:bool)
              n513 = case shown="False" w1029 {
                tunnel: w1035 -> [w1042 _]
                frame False {
                  n514 = local write "Single Series"(w1042) -> ()
                }
                frame True {
                }
              }
              n515 = property on="Single Series" class="LstBox (strict)"("Item Names"=w1036) -> ()  [unwired: 2 in, 2 out]
            }
            frame 6, Default {
              n516 = One Button Dialog(message="Warning- rogue filters found; ignoring!") -> ()  [unwired: 1 in, 1 out]
            }
          }
        }
        "Accept Array" <- w767
        n517 = Add(x=w758, y=2) -> (x+y=w756:i32)
        n518 = Equal?(x=w755, y=w756) -> (x = y?=w750:bool)
        n519 = And Array Elements(Boolean array=w769) -> (logical AND=w754:bool)
        n520 = Or(x=w754, y=w750) -> (x .or. y?=w753:bool)
        n521 = Select(t="First Loop True", s=w762, f="First Loop False") -> (s? t:f=w760:string)
        n522 = Select(t=w760, s=w753, f="Create Selectors") -> (s? t:f=w764:string)
      }
      frame "First Loop True" {
        n523 = stacked-sequence {
          tunnel: ["Select all for Filter 2" _] -> w1078
          tunnel: [TRUE ("OK?") _] -> w1077
          frame #0 {
            n524 = property on="Filter bins 1" class="LstBox (strict)"() -> ("Item Names"=w1084:string[])  [unwired: 2 in, 2 out]
            n525 = property on="Filter Bins 2" class="LstBox (strict)"() -> ("Item Names"=w1082:string[])  [unwired: 2 in, 2 out]
            n526 = local read "Filter Bins 2 Strings"() -> (w1085:string[])
            n527 = local read "Filter Bins 1 Strings"() -> (w1087:string[])
            n528 = for {
              tunnel: w1082 -> [w1092] mode=indexing
              tunnel: [w1091] -> w1081 mode=indexing
              n529 = call "Get_Options_without_numbers.vi"("String in"=w1092) -> ("after substring"=w1091:string)
            }
            n530 = for {
              tunnel: w1084 -> [w1094] mode=indexing
              tunnel: [w1093] -> w1083 mode=indexing
              n531 = call "Get_Options_without_numbers.vi"("String in"=w1094) -> ("after substring"=w1093:string)
            }
            n532 = for {
              tunnel: w1081 -> [w1100]
              tunnel: [w1096] -> w1086 mode=indexing
              tunnel: w1085 -> [w1095] mode=indexing
              n533 = Search 1D Array(1D array=w1100, element=w1095) -> (index of element=w1098:i32)  [unwired: 1 in]
              n534 = Greater Or Equal To 0?(x=w1098) -> (x >= 0?=w1099:bool)
              n535 = Select(t=w1098, s=w1099, f=0) -> (s? t:f=w1096:i32)
            }
            n536 = for {
              tunnel: w1083 -> [w1106]
              tunnel: [w1102] -> w1088 mode=indexing
              tunnel: w1087 -> [w1101] mode=indexing
              n537 = Search 1D Array(1D array=w1106, element=w1101) -> (index of element=w1104:i32)  [unwired: 1 in]
              n538 = Greater Or Equal To 0?(x=w1104) -> (x >= 0?=w1105:bool)
              n539 = Select(t=w1104, s=w1105, f=0) -> (s? t:f=w1102:i32)
            }
            n540 = local write "Filter Bins 2"(w1086) -> ()
            n541 = local write "Filter Bins 1"(w1088) -> ()
          }
          frame #1 {
            n542 = local read "Filters 3 onwards"() -> (w1132:string[])
            n543 = Index Array(array=w1132) -> (element #1=w1126:string, element #2=w1118:string, element #3=w1117:string)  [unwired: 3 in]
            n544 = Array Subset(array=w1132, index=3) -> (w1130:string[])  [unwired: 1 in]
            n545 = property on="Filter 3" class="Ring (strict)"() -> ("Strings []"=w1114:string[])  [unwired: 2 in, 2 out]
            n546 = property on="Single Series" class="LstBox (strict)"() -> ("Item Names"=w1112:string[])  [unwired: 2 in, 2 out]
            n547 = property on="Filter 4" class="Ring (strict)"() -> ("Strings []"=w1110:string[])  [unwired: 2 in, 2 out]
            n548 = property on="Filter 5" class="Ring (strict)"() -> ("Strings []"=w1109:string[])  [unwired: 2 in, 2 out]
            n549 = for {
              tunnel: w1110 -> [w1139] mode=indexing
              tunnel: [w1138] -> w1107 mode=indexing
              n550 = call "Get_Options_without_numbers.vi"("String in"=w1139) -> ("after substring"=w1138:string)
            }
            n551 = for {
              tunnel: w1112 -> [w1135] mode=indexing
              tunnel: [w1134] -> w1111 mode=indexing
              n552 = call "Get_Options_without_numbers.vi"("String in"=w1135) -> ("after substring"=w1134:string)
            }
            n553 = for {
              tunnel: w1114 -> [w1141] mode=indexing
              tunnel: [w1140] -> w1113 mode=indexing
              n554 = call "Get_Options_without_numbers.vi"("String in"=w1141) -> ("after substring"=w1140:string)
            }
            n555 = for {
              tunnel: w1109 -> [w1137] mode=indexing
              tunnel: [w1136] -> w1108 mode=indexing
              n556 = call "Get_Options_without_numbers.vi"("String in"=w1137) -> ("after substring"=w1136:string)
            }
            n557 = for {
              tunnel: w1111 -> [w1147]
              tunnel: [w1143] -> w1131 mode=indexing
              tunnel: w1130 -> [w1142] mode=indexing
              n558 = Search 1D Array(1D array=w1147, element=w1142) -> (index of element=w1145:i32)  [unwired: 1 in]
              n559 = Greater Or Equal To 0?(x=w1145) -> (x >= 0?=w1146:bool)
              n560 = Select(t=w1145, s=w1146, f=0) -> (s? t:f=w1143:i32)
            }
            n561 = Search 1D Array(1D array=w1113, element=w1126) -> (index of element=w1128:i32)  [unwired: 1 in]
            n562 = Search 1D Array(1D array=w1107, element=w1118) -> (index of element=w1123:i32)  [unwired: 1 in]
            n563 = Search 1D Array(1D array=w1108, element=w1117) -> (index of element=w1120:i32)  [unwired: 1 in]
            n564 = Greater Or Equal To 0?(x=w1128) -> (x >= 0?=w1127:bool)
            n565 = Greater Or Equal To 0?(x=w1123) -> (x >= 0?=w1124:bool)
            n566 = Greater Or Equal To 0?(x=w1120) -> (x >= 0?=w1119:bool)
            n567 = Select(t=w1128, s=w1127, f=0) -> (s? t:f=w1125:i32)
            n568 = Select(t=w1123, s=w1124, f=0) -> (s? t:f=w1115:i32)
            n569 = local write "Single Series"(w1131) -> ()
            n570 = Select(t=w1120, s=w1119, f=0) -> (s? t:f=w1116:i32)
            n571 = local write "Filter 3"(w1125) -> ()
            n572 = local write "Filter 5"(w1116) -> ()
            n573 = local write "Filter 4"(w1115) -> ()
          }
        }
      }
      frame "First Loop False" {
        n574 = stacked-sequence {
          tunnel: ["Select all for Filter 2" _] -> w1150
          tunnel: [TRUE ("OK?") _] -> w1149
          frame #0 {
            n575 = local read "Filter Bins 2"() -> (w1155:i32[])
            n576 = local read "Filter Bins 1"() -> (w1158:i32[])
            n577 = property on="Filter Bins 2" class="LstBox (strict)"() -> ("Item Names"=w1156:string[])  [unwired: 2 in, 2 out]
            n578 = property on="Filter bins 1" class="LstBox (strict)"() -> ("Item Names"=w1157:string[])  [unwired: 2 in, 2 out]
            n579 = for {
              tunnel: w1156 -> [w1164]
              tunnel: w1155 -> [w1163] mode=indexing
              tunnel: [w1161] -> w1154 mode=indexing
              n580 = Index Array(array=w1164, index=w1163) -> (element=w1162:string)
              n581 = call "Get_Options_without_numbers.vi"("String in"=w1162) -> ("after substring"=w1161:string)
            }
            n582 = for {
              tunnel: w1157 -> [w1168]
              tunnel: w1158 -> [w1167] mode=indexing
              tunnel: [w1165] -> w1153 mode=indexing
              n583 = Index Array(array=w1168, index=w1167) -> (element=w1166:string)
              n584 = call "Get_Options_without_numbers.vi"("String in"=w1166) -> ("after substring"=w1165:string)
            }
            n585 = local write "Filter Bins 2 Strings"(w1154) -> ()
            n586 = local write "Filter Bins 1 Strings"(w1153) -> ()
          }
          frame #1 {
            n587 = local read "Single Series"() -> (w1182:i32[])
            n588 = property on="Filter 5" class="Ring (strict)"() -> ("Strings []"=w1178:string[])  [unwired: 2 in, 2 out]
            n589 = property on="Filter 3" class="Ring (strict)"() -> ("Strings []"=w1184:string[])  [unwired: 2 in, 2 out]
            n590 = property on="Filter 4" class="Ring (strict)"() -> ("Strings []"=w1180:string[])  [unwired: 2 in, 2 out]
            n591 = property on="Single Series" class="LstBox (strict)"() -> ("Item Names"=w1181:string[])  [unwired: 2 in, 2 out]
            n592 = local read "Filter 5"() -> (w1177:u16)
            n593 = local read "Filter 4"() -> (w1179:u16)
            n594 = local read "Filter 3"() -> (w1183:u16)
            n595 = for {
              tunnel: w1182 -> [w1188] mode=indexing
              tunnel: w1181 -> [w1187]
              tunnel: [w1185] -> w1176 mode=indexing
              n596 = Index Array(array=w1187, index=w1188) -> (element=w1186:string)
              n597 = call "Get_Options_without_numbers.vi"("String in"=w1186) -> ("after substring"=w1185:string)
            }
            n598 = Index Array(array=w1184, index=w1183) -> (element=w1175:string)
            n599 = Index Array(array=w1180, index=w1179) -> (element=w1170:string)
            n600 = Index Array(array=w1178, index=w1177) -> (element=w1173:string)
            n601 = call "Get_Options_without_numbers.vi"("String in"=w1173) -> ("after substring"=w1172:string)
            n602 = call "Get_Options_without_numbers.vi"("String in"=w1170) -> ("after substring"=w1171:string)
            n603 = call "Get_Options_without_numbers.vi"("String in"=w1175) -> ("after substring"=w1174:string)
            n604 = Build Array (concatenate)(w1174, w1171, w1172, w1176) -> (w1169:string[])
            n605 = local write "Filters 3 onwards"(w1169) -> ()
            n606 = global write "Results_plotter_Global.vi" "Filters 3 onwards"(w1169) -> ()
          }
        }
      }
      frame "Select all for Filter 2" {
        n607 = property on="Filter Bins 2" class="LstBox (strict)"() -> ("Item Names"=w1193:string[], "Top Row"=w1191:i32)  [unwired: 2 in, 2 out]
        n608 = property on="Filter bins 1" class="LstBox (strict)"() -> ("Item Names"=w1195:string[], "Top Row"=w1194:i32)  [unwired: 2 in, 2 out]
        n609 = Array Size(array=w1195) -> (size(s)=w1196:i32)
        n610 = Array Size(array=w1193) -> (size(s)=w1192:i32)
        n611 = Less?(x=w1196, y=w1194) -> (x < y?=w1197:bool)
        n612 = Less?(x=w1192, y=w1191) -> (x < y?=w1190:bool)
        n613 = case shown="True" w1197 {
          frame False {
          }
          frame True {
            n614 = property on="Filter bins 1" class="LstBox (strict)"("Top Row"=0 ("Active Row:Active Row Number")) -> ()  [unwired: 2 in, 2 out]
          }
        }
        n615 = case shown="True" w1190 {
          frame False {
          }
          frame True {
            n616 = property on="Filter Bins 2" class="LstBox (strict)"("Top Row"=0 ("Active Row:Active Row Number")) -> ()  [unwired: 2 in, 2 out]
          }
        }
      }
      frame "Re Plot Data?" {
        n617 = global read "Results_plotter_Global.vi" "3D Ch Selectors"() -> (w1207:i32[])
        n618 = local read "Additional X Values"() -> (w1209:dbl[])
        n619 = local read "Additional Y Values"() -> (w1208:dbl[])
        n620 = local read "color and symbol"() -> (w1217:bool)
        n621 = local read "No of Contours"() -> (w1216:i32)
        n622 = local read "Multi Ordinate"() -> (w1212:i32[])
        n623 = local read "Intensity Plot?"() -> (w1210:bool)
        n624 = local read "Accept Array"() -> (w1211:bool[][])
        n625 = local read "Filter Bins 2"() -> (w1220:i32[])
        n626 = local read "Filter Bins 1"() -> (w1219:i32[])
        n627 = local read "Resolution"() -> (w1215:dbl)
        n628 = local read "Transpose"() -> (w1214:bool)
        n629 = local read "Point Size"() -> (w1218:i32)
        n630 = local read "Absisca"() -> (w1213:u16)
        n631 = Bundle("Filter Bins 2"=w1220, "Filter Bins 1"=w1219, "Point Size"=w1218, "color and symbol"=w1217, "No of Contours"=w1216, "Resolution"=w1215, "Transpose"=w1214, "Absisca"=w1213, "Multi Ordinate"=w1212, "Accept Array"=w1211, "Intensity Plot?"=w1210, "Additional X Values"=w1209, "Additional Y Values"=w1208, "3D Ch Selectors"=w1207) -> (w1206:T20)  [unwired: 1 in]
        n632 = global read "Results_plotter_Global.vi" "First Loop"() -> (w1204:bool)
        n633 = call "Is Value Changed.vim"("value"=w1206) -> ("changed or first call?"=w1205:bool)
        n634 = Compound Arithmetic op=OR(w1205, w1204) -> (w1222:bool)
        n635 = Select(t="Prepare for Plotting", s=w1222, f="What to do next?") -> (s? t:f=w1225:string)
      }
      frame "Prepare for Plotting" {
        n636 = local read "Multi Ordinate"() -> (w1234:i32[])
        n637 = local read "Filter Array"() -> (w1239:u16[])
        n638 = for {
          tunnel: w1234 -> [w1244] mode=indexing
          tunnel: [w1243] -> w1232 mode=indexing
          tunnel: w1233 -> [w1242]
          n639 = Index Array(array=w1242, index=w1244) -> (element=w1243:string)
        }
        n640 = Index Array(array=w1239, index=0 ("Index")) -> (element=w1236:u16)
        n641 = Equal To 0?(x=w1236) -> (x = 0?=w1237:bool)
        n642 = global write "Results_plotter_Global.vi" "Ordinate Strings"(w1232) -> ()
        n643 = case shown="False" w1237 {
          tunnel: w1236 -> [w1247 _]
          tunnel: w1233 -> [w1251 _]
          tunnel: [w1248 string[] ["None", "None (100)"]] -> w1231
          tunnel: w1229 -> [w1246 _]
          frame False {
            n644 = Array Size(array=w1246) -> (size(s)=w1245:i32)
            n645 = local read "Filter Bins 1"() -> (w1253:i32[])
            n646 = property on="Filter bins 1" class="LstBox (strict)"() -> ("Item Names"=w1252:string[])  [unwired: 2 in, 2 out]
            n647 = case shown="1" w1247 {
              selector: w1247 -> [w1254 w1260]
              tunnel: w1251 -> [_ w1261]
              tunnel: [w1255 w1257] -> w1249
              tunnel: w1246 -> [w1256 _]
              tunnel: w1245 -> [_ w1258]
              frame 1 {
                n648 = Index Array(array=w1256, index=w1254) -> (element=w1255:string)
              }
              frame Default {
                n649 = Subtract(x=w1260, y=w1258) -> (x-y=w1259:i32)
                n650 = Index Array(array=w1261, index=w1259) -> (element=w1257:string)
              }
            }
            n651 = for {
              tunnel: w1253 -> [w1264] mode=indexing
              tunnel: w1252 -> [w1263]
              tunnel: [w1262] -> w1250 mode=indexing
              n652 = Index Array(array=w1263, index=w1264) -> (element=w1262:string)
            }
            n653 = Build Array (concatenate)(w1249, w1250) -> (w1248:string[])
          }
          frame True {
          }
        }
        n654 = global write "Results_plotter_Global.vi" "Filter 1 Strings"(w1231) -> ()
      }
      frame "Prepare Filter2 strings" {
        n655 = local read "Filter Array"() -> (w1274:u16[])
        n656 = Index Array(array=w1274, index=1 ("Index")) -> (element=w1271:u16)
        n657 = Equal To 0?(x=w1271) -> (x = 0?=w1272:bool)
        n658 = case shown="False" w1272 {
          tunnel: w1271 -> [w1279 _]
          tunnel: w1270 -> [w1280 _]
          tunnel: [w1282 string[] ["None", "None (100)"]] -> w1268
          tunnel: w1266 -> [w1278 _]
          frame False {
            n659 = Array Size(array=w1278) -> (size(s)=w1277:i32)
            n660 = local read "Filter Bins 2"() -> (w1285:i32[])
            n661 = property on="Filter Bins 2" class="LstBox (strict)"() -> ("Item Names"=w1284:string[])  [unwired: 2 in, 2 out]
            n662 = case shown="1" w1279 {
              selector: w1279 -> [w1286 w1290]
              tunnel: w1280 -> [_ w1292]
              tunnel: [w1287 w1291] -> w1281
              tunnel: w1278 -> [w1288 _]
              tunnel: w1277 -> [_ w1289]
              frame 1 {
                n663 = Index Array(array=w1288, index=w1286) -> (element=w1287:string)
              }
              frame Default {
                n664 = Subtract(x=w1290, y=w1289) -> (x-y=w1293:i32)
                n665 = Index Array(array=w1292, index=w1293) -> (element=w1291:string)
              }
            }
            n666 = for {
              tunnel: w1285 -> [w1296] mode=indexing
              tunnel: w1284 -> [w1295]
              tunnel: [w1294] -> w1283 mode=indexing
              n667 = Index Array(array=w1295, index=w1296) -> (element=w1294:string)
            }
            n668 = Build Array (concatenate)(w1281, w1283) -> (w1282:string[])
          }
          frame True {
          }
        }
        n669 = global write "Results_plotter_Global.vi" "Filter 2 Strings"(w1268) -> ()
      }
      frame "Plot Data" {
        n670 = stacked-sequence {
          seq-local: [w1308 _ _] -> [_ w1394 _]
          seq-local: [w1307 _ _] -> [_ w1393 _]
          tunnel: [_ TRUE _] -> w1302
          tunnel: [_ _ w1428] -> w1301
          tunnel: w1300 -> [w1309 _ _]
          tunnel: w1298 -> [_ w1387 w1433]
          frame #0 {
            w1304 = T21 {"Upper"=0, "Lower"=0, "St Error"=0}  # Error_bars_index
            w1305 = -1 ("Upper")
            n671 = global read "Results_plotter_Global.vi" "Ordinate Strings"() -> (w1308:string[])
            n672 = Bundle By Name(cluster=w1304, "Upper"=w1305, "Lower"=w1305, "St Error"=w1305) -> (w1306:T21)
            n673 = for {
              tunnel: w1308 -> [w1312] mode=indexing
              tunnel: w1309 -> [w1314]
              tunnel: [w1313] -> w1307 mode=indexing
              tunnel: w1306 -> [w1310]
              n674 = String Length(string=w1312) -> (length=w1311:i32)
              n675 = for {
                tunnel: w1312 -> [w1319]
                tunnel: w1314 -> [w1316] mode=indexing
                shift-right: [w1322] -> w1313
                shift-left: w1310 -> [w1321]
                tunnel: w1311 -> [w1317]
                i -> [w1315]
                n676 = String Subset(string=w1316, length (rest)=w1317) -> (substring=w1318:string)  [unwired: 1 out]
                n677 = Equal?(x=w1318, y=w1319) -> (x = y?=w1320:bool)
                n678 = case shown="True" w1320 {
                  tunnel: [w1327 w1380] -> w1322
                  tunnel: w1315 -> [w1326 _]
                  tunnel: w1321 -> [w1325 w1380]
                  tunnel: w1317 -> [w1324 _]
                  tunnel: w1316 -> [w1323 _]
                  frame True {
                    n679 = stacked-sequence {
                      seq-local: [w1335 _ _] -> [_ w1353 _]
                      seq-local: [_ w1352 _] -> [_ _ w1367]
                      tunnel: [_ _ w1366] -> w1327
                      tunnel: w1326 -> [w1347 w1361 w1375]
                      tunnel: w1325 -> [w1346 _ _]
                      tunnel: w1324 -> [w1345 w1360 w1374]
                      tunnel: w1323 -> [w1344 w1359 w1373]
                      frame #0 {
                        n680 = String Subset(string=w1344, offset (0)=w1345) -> (substring=w1339:string)  [unwired: 1 out]
                        n681 = call <vilib>:"Trim Whitespace.vi"("string"=w1339) -> ("trimmed string"=w1330:string)  [unwired: 1 in]
                        n682 = Equal?(x=w1330, y="Err") -> (x = y?=w1341:bool)
                        n683 = Equal?(x=w1330, y="err") -> (x = y?=w1338:bool)
                        n684 = Equal?(x=w1330, y="St Error") -> (x = y?=w1336:bool)
                        n685 = Equal?(x=w1330, y="Std Error") -> (x = y?=w1333:bool)
                        n686 = Equal?(x=w1330, y="St Err") -> (x = y?=w1332:bool)
                        n687 = Equal?(x=w1330, y="Std Err") -> (x = y?=w1328:bool)
                        n688 = Compound Arithmetic op=OR(w1341, w1338, w1336, w1333, w1332, w1328) -> (w1340:bool)
                        n689 = case shown="True" w1340 {
                          tunnel: [w1348 w1351] -> w1335
                          tunnel: w1347 -> [w1349 _]
                          tunnel: w1346 -> [w1350 w1351]
                          frame True {
                            n690 = Bundle By Name(cluster=w1350, "St Error"=w1349) -> (w1348:T21)
                          }
                          frame False {
                          }
                        }
                      }
                      frame #1 {
                        n691 = String Subset(string=w1359, offset (0)=w1360) -> (substring=w1358:string)  [unwired: 1 out]
                        n692 = call <vilib>:"Trim Whitespace.vi"("string"=w1358) -> ("trimmed string"=w1357:string)  [unwired: 1 in]
                        n693 = To Lower Case(string=w1357) -> (all lower case string=w1355:string)
                        n694 = Match Pattern(string=w1355, regular expression="upper") -> (offset past match=w1354:i32)  [unwired: 1 in, 3 out]
                        n695 = case shown="Default" w1354 {
                          tunnel: [w1362 w1365] -> w1352
                          tunnel: w1361 -> [w1363 _]
                          tunnel: w1353 -> [w1364 w1365]
                          frame Default {
                            n696 = Bundle By Name(cluster=w1364, "Upper"=w1363) -> (w1362:T21)
                          }
                          frame -1 {
                          }
                        }
                      }
                      frame #2 {
                        n697 = String Subset(string=w1373, offset (0)=w1374) -> (substring=w1372:string)  [unwired: 1 out]
                        n698 = call <vilib>:"Trim Whitespace.vi"("string"=w1372) -> ("trimmed string"=w1371:string)  [unwired: 1 in]
                        n699 = To Lower Case(string=w1371) -> (all lower case string=w1369:string)
                        n700 = Match Pattern(string=w1369, regular expression="lower") -> (offset past match=w1368:i32)  [unwired: 1 in, 3 out]
                        n701 = case shown="Default" w1368 {
                          tunnel: [w1376 w1379] -> w1366
                          tunnel: w1375 -> [w1377 _]
                          tunnel: w1367 -> [w1378 w1379]
                          frame Default {
                            n702 = Bundle By Name(cluster=w1378, "Lower"=w1377) -> (w1376:T21)
                          }
                          frame -1 {
                          }
                        }
                      }
                    }
                  }
                  frame False {
                  }
                }
              }
            }
          }
          frame #1 {
            n703 = case shown="\"Item 0\", Default" "seriesColours" {
              tunnel: [u32[][] [[65280, 26112, 65433, 721135, 14417921], [65525, 153, 65535, 14872320, 65316], [16711680, 10027008, 16751103, 16737894, 16711884], [16776960, 16777215, 16777113, 16777164, 16777062], [10053120, 13408614, 10066176, 13408563, 16764057], [13369599, 16738047, 10040217, 16751103, 10040268], [13421772, 5000268, 13421772, 10066329, 16777215], [65535, 6750207, 10092543, 52479, 10092543]] ("Output Array 2") w1411] -> w1385
              frame "Item 0", Default {
              }
              frame "Item 1" {
                # "From ColorBrewerMaps.vi"
                n704 = Array Subset(array=u32[][] [[8374655, 1810039, 10931939, 16495790, 11789005, 14948892, 6734501, 9294791, 0, 0, 0, 0], [12496596, 14245634, 2062516, 11783651, 16633260, 3636920, 16551266, 16777139, 0, 0, 0, 0], [16629894, 7696563, 11722634, 13429701, 13358568, 5091146, 9281739, 12499674, 0, 0, 0, 0], [16777113, 15149450, 3383340, 14601188, 16042724, 9981603, 15174339, 16482418, 10053120, 13369599, 13421772, 65535], [3697840, 6727198, 16489113, 16701862, 15136201, 16744192, 10934356, 8434131, 13408614, 16738047, 5000268, 6750207], [15729279, 15117058, 14883356, 16777164, 16773806, 16777011, 16767279, 16626786, 10066176, 10040217, 13421772, 10092543], [12540695, 10909213, 16629615, 15063229, 15852236, 10901032, 15058068, 11787881, 13408563, 16751103, 10066329, 52479], [9466226, 6710886, 16744192, 16636652, 13421772, 16220607, 11776947, 16567781, 16764057, 10040268, 16777215, 10092543]] ("Output Array 2"), index (col)="brewSelect") -> (w1411:u32[][])  [unwired: 3 in]
              }
            }
            n705 = Array Size(array="Multi Ordinate") -> (size(s)=w1392:i32)
            n706 = global write "Results_plotter_Global.vi" "Ordinate"("Multi Ordinate") -> ()
            n707 = Greater?(x=w1392, y=1) -> (0:w1389:bool)
            n708 = Select(t=5, s=w1389, f=2 ("y")) -> (s? t:f=w1397:i32)
            n709 = while {
              shift-right: [w1415] -> w1401
              shift-left: _ -> [w1416]
              tunnel: "color and symbol" -> [w1417]
              tunnel: w1397 -> [w1413]
              stop <- FALSE continue-if-true
              n710 = case shown="True" w1417 {
                tunnel: w1416 -> [w1424 w1426]
                tunnel: [w1423 w1426] -> w1415
                tunnel: w1413 -> [w1418 _]
                frame True {
                  n711 = Add(x=w1424, y=1) -> (x+y=w1421:i32)
                  n712 = local write "color and symbol"(FALSE ("color and symbol")) -> ()
                  n713 = Greater?(x=w1421, y=w1418) -> (0:w1422:bool)
                  n714 = Select(t=0, s=w1422, f=w1421) -> (s? t:f=w1423:i32)
                }
                frame False {
                }
              }
            }
            n715 = local read "Accept Array"() -> (w1403:bool[][])
            n716 = call "Plot_XY_data.vi"("All Data In"=w1387, "Ordinate Strings"=w1394, "Swap color and symbol"=w1401, "Error bar ch index"=w1393, "Accept Array"=w1403, "Colour Array"=w1385, "Ordinate"="Multi Ordinate", "Absisca"="Absisca", "Transpose"="Transpose") -> ("X Scale.Format & Precision:Precision"=w1383:u8, "Accept Array Out"=→"Plotted Series":bool[][])  [unwired: 1 in, 4 out]
            n717 = global write "Results_plotter_Global.vi" "Transpose"("Transpose") -> ()
            n718 = global write "Results_plotter_Global.vi" "Absisca"("Absisca") -> ()
            n719 = case shown="\"X lin Y lin\", Default" "axes" {
              tunnel: [w1405 u8 1 ("X Scale.Format & Precision:Precision") u8 1 ("X Scale.Format & Precision:Precision") w1408] -> w1382
              tunnel: w1383 -> [w1405 _ _ w1408]
              frame "X lin Y lin", Default {
              }
              frame "X log Y log" {
              }
              frame "X log Y lin" {
              }
              frame "X lin Y log" {
              }
            }
            n720 = case shown="7" w1382 {
              tunnel: "%<%H:%M:%S\n%d-%b-'%y>T" -> [_ w1404]
              frame 0, Default {
              }
              frame 7 {
                n721 = property on="XY Plot" class="XYGraph (strict)"("XScale.FormatString"=w1404) -> ()  [unwired: 2 in, 2 out]
              }
            }
            n722 = property on="XY Plot" class="XYGraph (strict)"("X Scale.Format & Precision:Format"=w1382) -> ()  [unwired: 2 in, 2 out]
          }
          frame #2 {
            n723 = global read "Results_plotter_Global.vi" "Raw Data Filename index"() -> (w1434:i32)
            n724 = global read "Results_plotter_Global.vi" "Plotted Row Numbers"() -> (w1432:i32[])
            n725 = Index Array(array=w1433, index (col)=w1434) -> (element=w1431:string[])  [unwired: 1 in]
            n726 = for {
              tunnel: w1432 -> [w1441] mode=indexing
              tunnel: w1431 -> [w1440]
              tunnel: [w1439] -> w1430 mode=indexing
              n727 = Index Array(array=w1440, index=w1441) -> (element=w1439:string)
            }
            n728 = local read "graphPaneTab"() -> (w1429:T7)
            n729 = call "Analyse_string_array.vi"("String array"=w1430) -> ("Unique strings"=w1427:string[])  [unwired: 1 in, 1 out]
            n730 = case shown="\"3-D vector\"" w1429 {
              tunnel: ["Add Legend and scales" "Intensity plot" "Intensity plot" "3Dvectors" ("whereNext")] -> w1428
              frame "XY", Default {
              }
              frame "Contour" {
              }
              frame "3-D graphs" {
              }
              frame "3-D vector" {
              }
            }
            n731 = global write "Results_plotter_Global.vi" "Plotted Raw data Filenames"(w1427) -> ()
          }
        }
        "Index when last plotted" <- w1299
      }
      frame "Add Legend and scales" {
        # "finagle graph and legend size, to cope with change of legend"
        n732 = control-ref of="This VI"() -> (w1444:refnum<vi>)
        n733 = property class="VI"(reference=w1444) -> ("Minimum Panel Size"=w1443:T22, "Front Panel.PanelBounds"=w1442:T23)  [unwired: 1 in, 2 out]
        n734 = control-ref of="XY Plot"() -> (w1445:refnum<vi>)
        n735 = call "makeGraphLegend.vi"("Point"=w1443, "Rect"=w1442, "XYGraph in"=w1445) -> ()  [unwired: 9 in]
        n736 = local write "Warning!"("") -> ()
      }
      frame "Add Axis names" {
        (unwired) ""
        n737 = global read "Plot_Values_Global.vi" "XY Graph Cluster"() -> (w1456:cluster{dbl[], dbl[]}[])
        n738 = global read "Results_plotter_Global.vi" "Ordinate Strings"() -> (w1460:string[])
        n739 = for {
          shift-right: [w1543] -> w1467
          shift-left: "" -> [w1542]
          tunnel: [w1538] -> w1466
          tunnel: w1460 -> [w1537] mode=indexing
          i -> [w1538]
          n740 = String Length(string=w1542) -> (length=w1541:i32)
          n741 = Less?(x=w1541, y=40) -> (x < y?=w1539:bool)
          n742 = case shown="True" w1539 {
            tunnel: w1537 -> [_ w1548]
            tunnel: [w1544 w1547] -> w1543
            tunnel: w1542 -> [w1544 w1545]
            frame False {
            }
            frame True {
              n743 = Concatenate Strings(w1545, w1548, "   ") -> (w1547:string)
            }
          }
        }
        n744 = call "forceIncludeZeroes.vi"("forceX0"="forceX0", "forceY0"="forceY0", "XY Graph Cluster"=w1456) -> ("appended array"=w1455:cluster{"Array":dbl[], "Array":dbl[]}[])  [unwired: 8 in]
        n745 = Index Array(array=w1460) -> (element=w1463:string)  [unwired: 1 in]
        n746 = Greater Than 0?(x=w1466) -> (x > 0?=w1464:bool)
        n747 = String Length(string=w1467) -> (length=w1470:i32)
        n748 = Select(t="Multiple", s=w1464, f=w1463) -> (s? t:f=w1462:string)
        n749 = local read "Absisca"() -> (w1476:u16)
        n750 = local read "Transpose"() -> (w1475:bool)
        n751 = Subtract(x=w1470, y=3) -> (x-y=w1468:i32)
        n752 = Index Array(array=w1465, index=w1476) -> (element=w1474:string)
        n753 = String Subset(string=w1467, length (rest)=w1468) -> (substring=w1461:string)  [unwired: 1 out]
        n754 = case shown="False" w1475 {
          tunnel: [w1550 w1551] -> w1473
          tunnel: [w1549 w1552] -> w1472
          tunnel: w1474 -> [w1550 w1552]
          tunnel: w1462 -> [w1549 w1551]
          frame False {
          }
          frame True {
          }
        }
        n755 = global write "Results_plotter_Global.vi" "Value plotted Name"(w1461) -> ()
        n756 = local read "axes"() -> (w1452:T3)
        n757 = stacked-sequence {
          tunnel: w1455 -> [w1484 w1523]
          tunnel: w1452 -> [w1483 _]
          frame #0 {
            w1490 = u8 0 ("f")
            n758 = for {
              tunnel: [w1519] -> w1505 mode=indexing
              tunnel: [w1518] -> w1507 mode=indexing
              tunnel: [w1517] -> w1506 mode=indexing
              tunnel: [w1516] -> w1504 mode=indexing
              tunnel: w1484 -> [w1515] mode=indexing
              n759 = Unbundle(w1515) -> ("Array"=w1521:dbl[], "Array"=w1520:dbl[])
              n760 = Array Max & Min(array=w1521) -> (max value=w1519:dbl, min value=w1516:dbl)  [unwired: 2 out]
              n761 = Array Max & Min(array=w1520) -> (max value=w1517:dbl, min value=w1518:dbl)  [unwired: 2 out]
            }
            n762 = Array Max & Min(array=w1505) -> (max value=w1496:dbl)  [unwired: 3 out]
            n763 = Array Max & Min(array=w1504) -> (min value=w1495:dbl)  [unwired: 3 out]
            n764 = Array Max & Min(array=w1506) -> (max value=w1494:dbl)  [unwired: 3 out]
            n765 = Array Max & Min(array=w1507) -> (min value=w1493:dbl)  [unwired: 3 out]
            n766 = Subtract(x=w1496, y=w1495) -> (x-y=w1503:dbl)
            n767 = Subtract(x=w1494, y=w1493) -> (x-y=w1498:dbl)
            n768 = Logarithm Base 10(1:w1503) -> (0:w1502:dbl)
            n769 = Logarithm Base 10(1:w1498) -> (0:w1499:dbl)
            n770 = Negate(x=w1502) -> (-x=w1491:dbl)
            n771 = Negate(x=w1499) -> (-x=w1492:dbl)
            n772 = Increment(x=w1491) -> (x+1=w1489:dbl)
            n773 = Increment(x=w1492) -> (x+1=w1488:dbl)
            n774 = To Unsigned Byte Integer(number=w1488) -> (unsigned 8bit integer=w1487:u8)
            n775 = To Unsigned Byte Integer(number=w1489) -> (unsigned 8bit integer=w1486:u8)
            n776 = Increment(x=w1486) -> (x+1=w1485:u8)
            n777 = Greater Than 0?(x=w1486) -> (x > 0?=w1501:bool)
            n778 = Greater Than 0?(x=w1487) -> (x > 0?=w1500:bool)
            n779 = Increment(x=w1487) -> (x+1=w1497:u8)
            n780 = Select(t=w1485, s=w1501, f=w1490) -> (s? t:f=w1479:u8)
            n781 = Select(t=w1497, s=w1500, f=w1490) -> (s? t:f=w1480:u8)
            n782 = case shown="\"X lin Y lin\", Default" w1483 {
              tunnel: [w1509 w1510 1 w1513] -> w1482
              tunnel: [w1508 w1510 w1511 1] -> w1481
              tunnel: w1480 -> [w1508 _ w1511 _]
              tunnel: w1479 -> [w1509 _ _ w1513]
              frame "X lin Y lin", Default {
              }
              frame "X log Y log" {
                w1510 = 1
              }
              frame "X log Y lin" {
              }
              frame "X lin Y log" {
              }
            }
            n783 = property on="XY Plot" class="XYGraph (strict)"("XScale.Precision"=w1482, "YScale.Precision"=w1481) -> ()  [unwired: 2 in, 2 out]
          }
          frame #1 {
            n784 = property on="XY Plot" class="XYGraph (strict)"("Val(Sgnl)"=w1523) -> ()  [unwired: 2 in, 2 out]
            n785 = property on="Histogram" class="XYGraph (strict)"("Visible"="histOn") -> ()  [unwired: 2 in, 2 out]
            n786 = case shown="True" "histOn" {
              tunnel: w1523 -> [_ w1525]
              frame False {
              }
              frame True {
                n787 = for {
                  tunnel: w1525 -> [w1536] mode=indexing
                  tunnel: [w1532] -> w1524 mode=indexing
                  i -> [w1529]
                  n788 = property on="XY Plot" class="XYGraph (strict)"("Active Plot"=w1529) -> ("Plot.Plot Color"=w1531:u32)  [unwired: 2 in, 2 out]
                  n789 = Unbundle By Name(w1536) -> ("Array"=w1533:dbl[])
                  n790 = call <vilib>:"General Histogram.vi"("X"=w1533) -> ("Histogram"=w1534:i32[], "Axis"=w1535:dbl[])  [unwired: 10 in, 3 out]
                  n791 = property on="Histogram" class="XYGraph (strict)"("Active Plot"=w1529, "Plot.Plot Color"=w1531, "Plot.Line Style"=u8 2, "Plot.Plot Interpolation"=u8 0, "Plot.Bar Plot Style"=u8 10 ("Plot.Plot Interpolation"), "Plot.Line Width"=u8 3) -> ()  [unwired: 2 in, 2 out]
                  n792 = Bundle("Histogram"=w1534, "Axis"=w1535) -> (w1532:cluster{"Histogram":i32[], "Axis":dbl[]})  [unwired: 1 in]
                }
                "Histogram" <- w1524
              }
            }
            "XY Plot" <- w1523
          }
        }
        n793 = property on="XY Plot" class="XYGraph (strict)"("X Scale.Name Label.Text"=w1473, "Y Scale.Name Label.Text"=w1472) -> ()  [unwired: 2 in, 2 out]
        n794 = global write "Results_plotter_Global.vi" "X Axis Name"(w1473) -> ()
        n795 = global write "Results_plotter_Global.vi" "Y Axis Name"(w1472) -> ()
      }
      frame "Intensity plot" {
        # "Max"
        # "Min"
        n796 = global read "Plot_Values_Global.vi" "XY Graph Cluster"() -> (w1556:cluster{dbl[], dbl[]}[])
        n797 = local read "Tolerances"() -> (w1561:dbl[])
        n798 = local read "Transpose"() -> (w1557:bool)
        n799 = local read "Absisca"() -> (w1560:u16)
        n800 = stacked-sequence {
          seq-local: [w1572 _ _ _ _ _ _ _ _ _ _ _ _ _] -> [_ _ _ w1627 w1633 _ w1678 _ _ _ _ _ _ _]
          seq-local: [_ w1588 _ _ _ _ _ _ _ _ _ _ _ _] -> [_ _ _ _ w1632 _ w1677 _ _ _ _ _ _ _]
          seq-local: [_ _ w1623 _ _ _ _ _ _ _ _ _ _ _] -> [_ _ _ _ _ _ w1683 _ _ _ _ _ _ _]
          seq-local: [_ _ _ _ _ _ w1685 _ _ _ _ _ _ _] -> [_ _ _ _ _ _ _ _ _ w1724 _ _ _ _]
          seq-local: [_ _ _ _ _ _ w1684 _ _ _ _ _ _ _] -> [_ _ _ _ _ _ _ _ _ w1725 _ _ _ _]
          seq-local: [_ w1584 _ _ _ _ _ _ _ _ _ _ _ _] -> [_ _ _ _ _ _ _ _ _ _ w1792 _ _ _]
          seq-local: [_ _ _ w1625 _ _ _ _ _ _ _ _ _ _] -> [_ _ _ _ w1631 _ w1679 _ w1701 _ _ _ _ _]
          seq-local: [_ _ _ _ _ _ _ _ _ _ _ _ w1812 _] -> [_ _ _ _ _ _ _ _ _ _ _ _ _ w1858]
          seq-local: [_ _ _ _ _ _ _ _ _ _ _ _ w1811 _] -> [_ _ _ _ _ _ _ _ _ _ _ _ _ w1859]
          seq-local: [_ _ _ w1624 _ _ _ _ _ _ _ _ _ _] -> [_ _ _ _ _ w1646 _ _ _ _ _ _ _ _]
          seq-local: [_ _ _ _ _ _ w1671 _ _ _ _ _ _ _] -> [_ _ _ _ _ _ _ w1698 _ _ _ _ _ _]
          tunnel: [_ _ _ _ _ _ _ _ _ _ _ _ _ "Analyse Plot Space"] -> w1564
          tunnel: w1563 -> [w1570 _ _ _ _ _ _ _ _ _ w1782 _ _ _]
          tunnel: [w1570 _ _ _ _ _ _ _ _ _ _ _ _ _] -> w1562
          tunnel: w1561 -> [w1574 _ _ _ _ _ _ _ _ _ _ _ _ _]
          tunnel: w1556 -> [w1573 _ _ w1628 _ _ _ _ _ _ _ _ _ _]
          tunnel: w1560 -> [w1571 _ _ _ _ _ _ _ _ _ w1789 _ _ _]
          tunnel: w1557 -> [w1569 _ _ w1626 _ _ w1653 _ _ _ w1773 _ _ _]
          tunnel: [w1567 _ _ _ _ _ _ _ _ _ _ _ _ _] -> w1559
          tunnel: w1558 -> [w1567 _ _ _ _ _ _ _ _ _ w1783 _ _ _]
          tunnel: [w1566 _ _ _ _ _ _ _ _ _ _ _ _ _] -> w1555
          tunnel: w1554 -> [w1566 _ _ _ _ _ _ _ _ _ _ _ _ _]
          frame #0 {
            n801 = Not(x=w1569) -> (.not. x?=w1565:bool)
            n802 = Index Array(array=w1574, index=w1571) -> (element=w1568:dbl)
            n803 = for {
              tunnel: w1573 -> [w1583] mode=indexing
              tunnel: w1565 -> [w1580]
              shift-right: [w1578] -> w1575
              shift-left: dbl[] [] -> [w1579]
              n804 = Unbundle(w1583) -> (w1582:dbl[], w1581:dbl[])
              n805 = Select(t=w1582, s=w1580, f=w1581) -> (s? t:f=w1577:dbl[])
              n806 = Build Array (concatenate)(w1579, w1577) -> (w1578:dbl[])
            }
            n807 = call "Numeric_bins.vi"("Values"=w1575, "Tolerance"=w1568) -> ("Bin Centres"=w1572:dbl[])  [unwired: 2 out]
          }
          frame #1 {
            n808 = local read "Filter Bins 2"() -> (w1589:i32[])
            n809 = local read "Filter Bins 1"() -> (w1591:i32[])
            n810 = Array Size(array=w1589) -> (size(s)=w1593:i32)
            n811 = Array Size(array=w1591) -> (size(s)=w1594:i32)
            n812 = Greater Or Equal?(x=w1594, y=w1593) -> (x >= y?=w1592:bool)
            n813 = case shown="False" w1592 {
              tunnel: w1591 -> [_ w1616]
              tunnel: [w1612 w1616] -> w1590
              tunnel: [w1613 w1615] -> w1586
              tunnel: w1589 -> [w1612 _]
              tunnel: [1 0] -> w1584
              frame False {
                n814 = property on="Filter Bins 2" class="LstBox (strict)"() -> ("Item Names"=w1613:string[])  [unwired: 2 in, 2 out]
              }
              frame True {
                n815 = property on="Filter Bins 1" class="LstBox (strict)"() -> ("Item Names"=w1615:string[])  [unwired: 2 in, 2 out]
              }
            }
            n816 = Array Size(array=w1586) -> (size(s)=w1585:i32)
            n817 = for {
              tunnel: w1590 -> [w1599] mode=indexing
              tunnel: w1586 -> [w1605]
              shift-right: [w1602] -> w1588
              shift-left: dbl[] [] -> [w1603]
              tunnel: w1585 -> [w1598]
              n818 = Index Array(array=w1605, index=w1599) -> (element=w1601:string)
              n819 = Less?(x=w1599, y=w1598) -> (x < y?=w1597:bool)
              n820 = Match Pattern(string=w1601, regular expression=" (0)") -> (offset past match=w1600:i32)  [unwired: 4 out]
              n821 = Less Than 0?(x=w1600) -> (x < 0?=w1596:bool)
              n822 = And(x=w1596, y=w1597) -> (x .and. y?=w1595:bool)
              n823 = case shown="True" w1595 {
                tunnel: w1603 -> [w1606 w1610]
                tunnel: [w1606 w1609] -> w1602
                tunnel: w1601 -> [_ w1608]
                frame False {
                }
                frame True {
                  n824 = Fract/Exp String To Number(string=w1608) -> (number=w1607:dbl)  [unwired: 4 out]
                  n825 = Build Array (concatenate)(w1610, w1607) -> (w1609:dbl[])
                }
              }
            }
          }
          frame #2 {
            n826 = local read "Multi Ordinate"() -> (w1621:i32[])
            n827 = global read "Results_plotter_Global.vi" "Min Values"() -> (w1617:string[])
            n828 = Index Array(array=w1621, index=0 ("Index")) -> (element=w1620:i32)
            n829 = Index Array(array=w1617, index=w1620) -> (element=w1622:string)
            n830 = Fract/Exp String To Number(string=w1622, default (0 dbl)=nan) -> (number=w1623:dbl)  [unwired: 3 out]
          }
          frame #3 {
            n831 = call "Grid_Data.vi"("Transpose"=w1626, "XY Graph"=w1628, "Bin Centres"=w1627) -> ("No of Duplicates"=w1624:i32, "Grided data"=w1625:dbl[][])
          }
          frame #4 {
            n832 = for {
              tunnel: w1633 -> [w1638]
              tunnel: w1632 -> [w1637] mode=indexing
              tunnel: w1631 -> [w1636] mode=indexing
              shift-right: [w1634] -> w1629
              shift-left: dbl[][] [] -> [w1635]
              n833 = for {
                tunnel: w1638 -> [w1644] mode=indexing
                tunnel: w1637 -> [w1639]
                tunnel: w1636 -> [w1643] mode=indexing
                shift-right: [w1640] -> w1634
                shift-left: w1635 -> [w1642]
                n834 = Build Array(w1644, w1639, w1643) -> (w1641:dbl[])
                n835 = Build Array (concatenate)(w1642, w1641) -> (w1640:dbl[][])
              }
            }
            n836 = global write "Results_plotter_Global.vi" "Intensity Plot data in rows"(w1629) -> ()
          }
          frame #5 {
            n837 = case shown="1, Default" w1646 {
              selector: w1646 -> [_ w1648]
              tunnel: ["" w1649] -> w1645
              frame 0 {
              }
              frame 1, Default {
                n838 = Format Into String(format string="%d duplicate points have been averaged together!", w1648) -> (resulting string=w1649:string)  [unwired: 2 in, 1 out]
              }
            }
            "Warning!" <- w1645
          }
          frame #6 {
            n839 = call "Insert_extra_rows_and_col.vi"("Row Values In"=w1677, "Additional Row Values"="Additional X Values", "Column Values In"=w1678, "Data In"=w1679, "Additional Column Values"="Additional Y Values") -> ("Row Values Out"=w1657:dbl[], "Column Values Out"=w1656:dbl[], "Data Out"=w1652:dbl[][])  [unwired: 2 out]
            n840 = Swap Values(12:w1657, 13:w1653, 14:w1656) -> (1:w1655:dbl[], 3:w1654:dbl[])
            n841 = case shown="True" w1653 {
              tunnel: w1652 -> [w1687 w1689]
              tunnel: [w1687 w1688] -> w1651
              frame False {
              }
              frame True {
                n842 = Transpose 2D Array(2D array=w1689) -> (transposed array=w1688:dbl[][])
              }
            }
            n843 = Select(t="Resolution", s="Plot Resolution", f=0.0) -> (s? t:f=w1673:dbl)
            n844 = Array Max & Min(array=w1655) -> (max value=w1666:dbl, min value=w1665:dbl)  [unwired: 2 out]
            n845 = Array Max & Min(array=w1654) -> (max value=w1662:dbl, min value=w1663:dbl)  [unwired: 2 out]
            n846 = call "2D_interpolation.vi"("X Axis Current"=w1656, "Min Z Value In"=w1683, "Y axis Current"=w1657, "Bkgnd Value"="Bkgnd Value", "Plot In"=w1652, "Increment Value"=w1673, "Transpose"=w1653, "Point Size"="Point Size") -> ("min Z value"=w1685:dbl, "max Z value"=w1684:dbl, "Increment Value Out"=w1661:dbl, "Axis info"=w1671:T24, "Plot Out"=w1686:dbl[][], "Raw Interpolation"=w1658:dbl[][])  [unwired: 2 out]
            n847 = call-poly <vilib>:"Plot Helper.vi"("z matrix"=w1651, "y vector"=w1654, "x vector"=w1655) -> ("3D Plot lvclass Array out"=→"3D Stem":refnum<class "3D Plot Datatype.lvclass">[])  [unwired: 3 in, 5 out]
            n848 = call-poly <vilib>:"Ramp Pattern.vi"("start"=w1665, "end"=w1666, "delta"=w1661) -> ("Ramp Pattern"=w1664:dbl[])  [unwired: 6 in, 2 out]
            n849 = call-poly <vilib>:"Ramp Pattern.vi"("start"=w1663, "end"=w1662, "delta"=w1661) -> ("Ramp Pattern"=w1660:dbl[])  [unwired: 6 in, 2 out]
            n850 = global write "Results_plotter_Global.vi" "Raw Interpolation"(w1658) -> ()
            n851 = Transpose 2D Array(2D array=w1686) -> (transposed array=→"Intensity Graph":dbl[][])
            n852 = Build Array(w1660) -> (w1668:dbl[][])
            n853 = Build Array(w1664) -> (w1669:dbl[][])
            n854 = local write "Resolution"(w1661) -> ()
            n855 = call-poly <vilib>:"Plot Helper.vi"("z matrix"=w1658, "y matrix"=w1668, "x matrix"=w1669) -> ("3D Plot lvclass Array out"=→"3D Surface":refnum<class "3D Plot Datatype.lvclass">[])  [unwired: 3 in, 5 out]
          }
          frame #7 {
            n856 = Unbundle By Name(w1698) -> ("X Max"=w1697:dbl, "Y Max"=w1696:dbl, "X Scale"=w1695:cluster{"Xo":dbl, "delta X":dbl}, "Y Scale"=w1694:cluster{"Xo":dbl, "delta X":dbl}, "X Values"=w1693:dbl[], "Y Values"=w1692:dbl[], "Z Max"=w1691:dbl, "Z Min"=w1690:dbl)
            n857 = global write "Results_plotter_Global.vi" "X Max"(w1697) -> ()
            n858 = global write "Results_plotter_Global.vi" "Y Max"(w1696) -> ()
            n859 = global write "Results_plotter_Global.vi" "X Scale"(w1695) -> ()
            n860 = global write "Results_plotter_Global.vi" "Y Scale"(w1694) -> ()
            n861 = global write "Results_plotter_Global.vi" "X Values"(w1693) -> ()
            n862 = global write "Results_plotter_Global.vi" "Y Values"(w1692) -> ()
            n863 = global write "Results_plotter_Global.vi" "Z Max"(w1691) -> ()
            n864 = global write "Results_plotter_Global.vi" "Z Min"(w1690) -> ()
          }
          frame #8 {
            n865 = global read "Results_plotter_Global.vi" "X Scale"() -> (w1710:cluster{"Xo":dbl, "delta X":dbl})
            n866 = global read "Results_plotter_Global.vi" "Y Scale"() -> (w1706:cluster{"Xo":dbl, "delta X":dbl})
            n867 = global read "Results_plotter_Global.vi" "Y Max"() -> (w1707:dbl)
            n868 = global read "Results_plotter_Global.vi" "X Max"() -> (w1708:dbl)
            n869 = Unbundle By Name(w1706) -> ("Xo"=w1705:dbl)
            n870 = Subtract(x=w1707, y=w1705) -> (x-y=w1711:dbl)
            n871 = Unbundle By Name(w1710) -> ("Xo"=w1709:dbl)
            n872 = Subtract(x=w1708, y=w1709) -> (x-y=w1720:dbl)
            n873 = Array Max & Min(array=w1701) -> (max value=w1699:dbl, min value=w1700:dbl)  [unwired: 2 out]
            n874 = Greater?(x=w1711, y=5.0) -> (0:w1713:bool)
            n875 = property on="3D Stem" class="3D Stem (strict)"("Axis:Active Axis"=enum16{"X-axis", "Y-axis", "Z-axis"}."Z-axis", "Axis:Range Maximum"=w1699, "Axis:Range Minimum"=w1700) -> ()  [unwired: 2 in, 2 out]
            n876 = Greater?(x=w1720, y=5.0) -> (0:w1718:bool)
            n877 = Select(t=u8 0 ("Write Attribute"), s=w1713, f=u8 3) -> (s? t:f=w1703:u8)
            n878 = Select(t=u8 0 ("Write Attribute"), s=w1718, f=u8 3) -> (s? t:f=w1704:u8)
            n879 = property on="Intensity Graph" class="IntGraph (strict)"("X Scale.Offset and Multiplier"=w1710, "X Scale.Range:Maximum"=w1708, "Y Scale.Offset and Multiplier"=w1706, "Y Scale.Range:Maximum"=w1707, "X Scale.Format & Precision:Precision"=w1704, "Y Scale.Format & Precision:Precision"=w1703) -> ()  [unwired: 2 in, 2 out]
          }
          frame #9 {
            n880 = Less Than 0?(x=w1724) -> (x < 0?=w1723:bool)
            n881 = Greater Than 0?(x=w1725) -> (x > 0?=w1722:bool)
            n882 = And(x=w1722, y=w1723) -> (x .and. y?=w1721:bool)
            n883 = case shown="False" w1721 {
              tunnel: w1725 -> [w1754 w1767]
              tunnel: [w1761 w1765] -> w1727
              tunnel: w1724 -> [w1750 w1762]
              frame True {
                (unwired) u32 3743
                (unwired) u32 16721152
                n884 = Absolute Value(x=w1754) -> (abs(x)=w1756:dbl)
                n885 = Absolute Value(x=w1750) -> (abs(x)=w1728:dbl)
                n886 = Max & Min(x=w1756, y=w1728) -> (max(x,y)=w1752:dbl)  [unwired: 1 out]
                n887 = Divide(x=w1728, y=w1752) -> (x/y=w1744:dbl)
                n888 = Divide(x=w1754, y=w1752) -> (x/y=w1748:dbl)
                n889 = Subtract(x=1.0, y=w1744) -> (x-y=w1743:dbl)
                n890 = Subtract(x=1.0, y=w1748) -> (x-y=w1746:dbl)
                n891 = Multiply(x=w1743, y=u32 255) -> (x*y=w1749:dbl)
                n892 = Multiply(x=w1746, y=u32 255) -> (x*y=w1742:dbl)
                n893 = To Unsigned Long Integer(number=w1749) -> (unsigned 32bit integer=w1733:u32)
                n894 = To Unsigned Long Integer(number=w1742) -> (unsigned 32bit integer=w1729:u32)
                n895 = Multiply(x=w1733, y=u32 256) -> (x*y=w1735:u32)
                n896 = Multiply(x=u32 65536, y=w1733) -> (x*y=w1732:u32)
                n897 = Multiply(x=w1729, y=u32 256) -> (x*y=w1739:u32)
                n898 = Compound Arithmetic op=ADD(w1732, w1735, u32 255) -> (w1731:u32)
                n899 = Bundle("min Z value"=w1750, w1731) -> (w1758:cluster{"min Z value":dbl, u32})  [unwired: 1 out]
                n900 = Compound Arithmetic op=ADD(w1729, w1739, u32 16711680) -> (w1730:u32)
                n901 = Bundle("max Z value"=w1754, w1730) -> (w1760:cluster{"max Z value":dbl, u32})  [unwired: 1 out]
                n902 = Bundle("max Z value"=0.0, u32 16777215) -> (w1757:cluster{"max Z value":dbl, u32})  [unwired: 1 out]
                n903 = Build Array(w1760, w1758) -> (w1759:cluster{"min Z value":dbl, u32}[])
                n904 = Build Array (concatenate)(w1759, w1757) -> (w1761:cluster{"max Z value":dbl, u32}[])
              }
              frame False {
                n905 = Bundle("max Z value"=w1767, u32 16721152) -> (w1764:cluster{"max Z value":dbl, u32})  [unwired: 1 out]
                n906 = Bundle("min Z value"=w1762, u32 16448250) -> (w1763:cluster{"min Z value":dbl, u32})  [unwired: 1 out]
                n907 = Build Array(w1764, w1763) -> (w1765:cluster{"min Z value":dbl, u32}[])
              }
            }
            n908 = property on="Intensity Graph" class="IntGraph (strict)"("Ignore Array"=FALSE ("Write Attribute"), "Z Scale.Marker Values[]"=w1727) -> ()  [unwired: 2 in, 2 out]
          }
          frame #10 {
            n909 = local read "Filter Array"() -> (w1791:u16[])
            n910 = Index Array(array=w1791, index=w1792) -> (element=w1790:u16)
            n911 = Decrement(x=w1790) -> (x-1=w1781:u16)
            n912 = Decrement(x=w1781) -> (x-1=w1788:u16)
            n913 = local read "Multi Ordinate"() -> (w1787:i32[])
            n914 = Index Array(array=w1783, index=w1789) -> (element=w1771:string)
            n915 = Index Array(array=w1783, index=w1788) -> (element=w1772:string)
            n916 = Index Array(array=w1787, index=0) -> (element=w1785:i32)
            n917 = Swap Values(12:w1772, 13:w1773, 14:w1771) -> (1:w1770:string, 3:w1769:string)
            n918 = Index Array(array=w1782, index=w1785) -> (element=w1784:string)
            n919 = global read "Results_plotter_Global.vi" "Value plotted Name"() -> (w1774:string)
            n920 = global write "Results_plotter_Global.vi" "Value plotted Name"(w1784) -> ()
            n921 = property on="Intensity Graph" class="IntGraph (strict)"("Y Scale.Name Label.Text"=w1770, "XScale.NameLbl.Text"=w1769) -> ()  [unwired: 2 in, 2 out]
            n922 = global write "Results_plotter_Global.vi" "X Axis Name"(w1770) -> ()
            n923 = global write "Results_plotter_Global.vi" "Y Axis Name"(w1769) -> ()
            n924 = property on="3D Stem" class="3D Stem (strict)"("Axis:Active Axis"=enum16{"X-axis", "Y-axis", "Z-axis"}."X-axis", "Axis:Name Label Text"=w1770, "Axis:Active Axis"=enum16{"X-axis", "Y-axis", "Z-axis"}."Y-axis", "Axis:Name Label Text"=w1769, "Axis:Active Axis"=enum16{"X-axis", "Y-axis", "Z-axis"}."Z-axis", "Axis:Name Label Text"=w1774) -> ()  [unwired: 2 in, 2 out]
            n925 = property on="3D Surface" class="3D Surface (strict)"("Axis:Active Axis"=enum16{"X-axis", "Y-axis", "Z-axis"}."Y-axis", "Axis:Name Label Text"=w1769, "Axis:Active Axis"=enum16{"X-axis", "Y-axis", "Z-axis"}."X-axis", "Axis:Name Label Text"=w1770, "Axis:Active Axis"=enum16{"X-axis", "Y-axis", "Z-axis"}."Z-axis", "Axis:Name Label Text"=w1774) -> ()  [unwired: 2 in, 2 out]
          }
          frame #11 {
            n926 = property on="Intensity Graph" class="IntGraph (strict)"() -> ("Color Table"=w1794:u32[])  [unwired: 2 in, 2 out]
            n927 = Increment(x="No of Contours") -> (x+1=w1795:i32)
            n928 = Divide(x=255, y=w1795) -> (x/y=w1798:dbl)
            n929 = To Long Integer(number=w1798) -> (32bit integer=w1797:i32)
            n930 = for {
              tunnel: w1797 -> [w1805]
              tunnel: [w1802] -> w1793 mode=indexing
              tunnel: w1794 -> [w1801] mode=indexing
              i -> [w1806]
              n931 = Increment(x=w1806) -> (x+1=w1803:i32)
              n932 = Quotient & Remainder(x=w1803, y=w1805) -> (x-y*floor(x/y)=w1804:i32)  [unwired: 1 out]
              n933 = case shown="0" w1804 {
                tunnel: [w1807 w1808] -> w1802
                tunnel: w1801 -> [_ w1808]
                frame 0 {
                  w1807 = u32 6316128  # contour colour
                }
                frame 1, Default {
                }
              }
            }
            n934 = property on="Intensity Graph" class="IntGraph (strict)"("Ignore Array"=TRUE ("Write Attribute"), "Color Table"=w1793) -> ()  [unwired: 2 in, 2 out]
          }
          frame #12 {
            n935 = global read "Results_plotter_Global.vi" "Raw Interpolation"() -> (w1810:dbl[][])
            n936 = Array Size(array=w1810) -> (size(s)=w1817:i32[])
            n937 = Decrement(x=w1817) -> (x-1=w1815:i32[])
            n938 = Index Array(array=w1815) -> (element #1=w1816:i32, element #2=w1809:i32)  [unwired: 2 in]
            n939 = for {
              N: w1816 -> [_]
              tunnel: w1810 -> [w1825]
              tunnel: w1809 -> [w1824]
              shift-right: [w1820] -> w1812
              shift-left: 0.0 -> [w1821]
              shift-right: [w1819] -> w1811
              shift-left: 0 -> [w1818]
              i -> [w1823]
              n940 = Increment(x=w1823) -> (x+1=w1822:i32)
              n941 = for {
                N: w1824 -> [_]
                tunnel: w1825 -> [w1834]
                tunnel: w1823 -> [w1839]
                tunnel: w1822 -> [w1837]
                shift-right: [w1830] -> w1820
                shift-left: w1821 -> [w1829]
                shift-right: [w1826] -> w1819
                shift-left: w1818 -> [w1827]
                i -> [w1838]
                n942 = Increment(x=w1838) -> (x+1=w1836:i32)
                n943 = Index Array(array=w1834, index (row)=w1839, index (col)=w1836) -> (element=w1835:dbl)
                n944 = Index Array(array=w1834, index (row)=w1837, index (col)=w1836) -> (element=w1832:dbl)
                n945 = Index Array(array=w1834, index (row)=w1839, index (col)=w1838) -> (element=w1840:dbl)
                n946 = Index Array(array=w1834, index (row)=w1837, index (col)=w1838) -> (element=w1833:dbl)
                n947 = Compound Arithmetic op=ADD(w1840, w1835, w1833, w1832) -> (w1828:dbl)
                n948 = Not A Number/Path/Refnum?(number/path/refnum=w1828) -> (NaN/Path/Refnum?=w1831:bool)
                n949 = case shown="False" w1831 {
                  tunnel: [w1844 w1848] -> w1830
                  tunnel: w1829 -> [w1846 w1848]
                  tunnel: w1828 -> [w1845 _]
                  tunnel: [w1843 w1847] -> w1826
                  tunnel: w1827 -> [w1842 w1847]
                  frame False {
                    n950 = Add(x=1, y=w1842) -> (x+y=w1843:i32)
                    n951 = Add(x=w1845, y=w1846) -> (x+y=w1844:dbl)
                  }
                  frame True {
                  }
                }
              }
            }
          }
          frame #13 {
            n952 = Divide(x=w1858, y=4.0) -> (x/y=w1856:dbl)
            n953 = local read "Resolution"() -> (w1860:dbl)
            n954 = Square(x=w1860) -> (x^2=w1852:dbl)
            n955 = Multiply(x=w1856, y=w1852) -> (x*y=w1850:dbl)
            "Surface Integral" <- w1850
            n956 = Multiply(x=w1852, y=w1859) -> (x*y=w1853:dbl)
            "Surface Area" <- w1853
            n957 = Divide(x=16666667, y=w1850) -> (x/y=→"Uadvec":dbl)
            n958 = Divide(x=w1850, y=w1853) -> (x/y=→"Surface Average":dbl)
            n959 = global write "Results_plotter_Global.vi" "Surface Area"(w1853) -> ()
            n960 = global write "Results_plotter_Global.vi" "Surface Integral"(w1850) -> ()
          }
        }
      }
      frame "3Dvectors" {
        # "Ought to provide explicit Model/ Tunnel coordinate control. Need to pull vector production up a level."
        n961 = local read "worldRef"() -> (w1885:refnum<vi>)
        n962 = global read "Results_plotter_Global.vi" "Ordinate Strings"() -> (w1892:string[])
        n963 = call "startWorld.vi"("axisLength"="axesLength", "SceneObjectIn"=w1885) -> ("error out"=w1872:errorcluster, "axesOut"=→"axesRef":refnum<vi>, "SceneObject out"=w1873:refnum<vi>)  [unwired: 7 in]
        n964 = Index Array(array=w1892) -> (element=→"scalar":string)  [unwired: 1 in]
        n965 = local read "Multi Ordinate"() -> (w1882:i32[])
        n966 = local read "Plotted Series"() -> (w1883:bool[][])
        n967 = call "addChangeVectors.vi"("keySettings"="keySettings", "vectorDims"="vectorDims", "channelValues"=w1884, "error in (no error)"=w1872, "Multi Ordinate"=w1882, "Plotted Series"=w1883, "parentObjectIn"=w1873) -> ("error out"=w1889:errorcluster, "colourRampVals"=w1875:cluster{"value":dbl, "colour":u32}[], "STLs"=w1869:T26, "parentObjectOut"=w1890:refnum<vi>, "whitePoint"=w1876:dbl)
        n968 = local read "Job Directory"() -> (w1886:path)
        n969 = property on="Key" class="ColRmp (strict)"("Scale.MarkerVals[]"=w1875, "Scale.FormatString"="%#_4g" ("Scale.Format String"), "Scale.High Color"=u32 16699913, "Scale.Low Color"=u32 50432, "Value"=w1876) -> ()  [unwired: 2 in, 2 out]
        n970 = call "addChangeSTLs.vi"("error in (no error)"=w1889, "Job Directory"=w1886, "STLs"=w1869, "parentObjectIn"=w1890) -> ("parentObjectOut"=w1861:refnum<vi>, "tunstlBits"=→"tunnelSTLbits":refnum<vi>[], "TTstlBits"=→"TTstlBits":refnum<vi>[], "tunnelRef"=w1865:refnum<vi>, "turntableRef"=w1867:refnum<vi>)  [unwired: 2 in, 1 out]
        "worldRef" <- w1861
        n971 = call "plainPaint.vi"("colourSpec"="Turntable", "reference"=w1867) -> ("reference out"=w1868:refnum<vi>)  [unwired: 8 in, 1 out]
        n972 = call "setTransforms.vi"("transform"="TTshift", "SceneObject in"=w1868) -> ("SceneObject out"=→"TTref":refnum<vi>)  [unwired: 8 in, 1 out]
        n973 = call "plainPaint.vi"("colourSpec"="Tunnel", "reference"=w1865) -> ("reference out"=→"tunnelRef":refnum<vi>)  [unwired: 8 in, 1 out]
        n974 = local write "3D Picture"(w1861) -> ()
      }
      frame "3Dpopout" {
        n975 = global read "Results_plotter_Global.vi" "Filter 2 Strings"() -> (w1902:string[])
        n976 = global read "Results_plotter_Global.vi" "Filter 1 Strings"() -> (w1904:string[])
        n977 = local read "Job Directory"() -> (w1906:path)
        n978 = call "filterStringsToString.vi"("filterStrings"=w1902) -> ("flatString"=w1901:string)  [unwired: 10 in]
        n979 = call "filterStringsToString.vi"("filterStrings"=w1904) -> ("flatString"=w1903:string)  [unwired: 10 in]
        n980 = local read "Template"() -> (w1907:path)
        n981 = Concatenate Strings(w1903, "-" ("string"), w1901) -> (w1899:string)
        n982 = Build Path(base path=w1906, name or relative path="3Dplot") -> (appended path=w1898:path)
        n983 = Build Path(base path=w1898, name or relative path=w1899) -> (appended path=w1897:path)
        n984 = call "3Dlauncher.vi"("dataFilePath"=w1897, "Data"=w1909, "Template Filename"=w1907, "Channel Names"=w1913) -> ()  [unwired: 1 in]
        n985 = local write "3Dplotter"(FALSE ("Vector Plot?")) -> ()
      }
      frame "Analyse Plot Space" {
        n986 = case shown="True" "Show Plot Space Analysis" {
          tunnel: w1917 -> [_ w1925]
          tunnel: w1915 -> [_ w1920]
          frame False {
          }
          frame True {
            w1922 = TRUE  # Summarise All
            n987 = global read "Results_plotter_Global.vi" "Plotted Row Numbers"() -> (w1921:i32[])
            n988 = for {
              tunnel: w1921 -> [w1928] mode=indexing
              tunnel: w1920 -> [w1927]
              tunnel: [w1926] -> w1923 mode=indexing
              n989 = Index Array(array=w1927, index (row)=w1928) -> (element=w1926:string[])  [unwired: 1 in]
            }
            n990 = call "Summarise.vi"("Channel Names"=w1925, "Data"=w1923, "Summarise All"=w1922) -> ("Summary"=w1924:string[][])  [unwired: 2 in]
            n991 = call "Plot_Space_Analysis.vi"("Table"=w1924) -> ()
          }
        }
      }
      frame "Vector Plot" {
        n992 = local read "Job Directory"() -> (w1931:path)
        n993 = local read "Template"() -> (w1932:path)
        n994 = Build Path(base path=w1931, name or relative path="Vectors") -> (appended path=w1930:path)
        n995 = call "Vector_Plotting.vi"("JobVectorDirectory"=w1930, "Data"=w1934, "Template Filename"=w1932, "Channel Names"=w1938) -> ()  [unwired: 1 in]
        n996 = local write "Vector Plot?"(FALSE ("Vector Plot?")) -> ()
      }
      frame "Coloured Dot Plot" {
        n997 = local read "Job Directory"() -> (w1941:path)
        n998 = local read "Template"() -> (w1942:path)
        n999 = Build Path(base path=w1941, name or relative path="Dot_Plot") -> (appended path=w1940:path)
        n1000 = call "Coloured_Dot_Plotting.vi"("JobVectorDirectory"=w1940, "Data"=w1944, "Template Filename"=w1942, "Channel Names"=w1948) -> ()  [unwired: 1 in]
        n1001 = local write "Dot Plot?"(FALSE ("Vector Plot?")) -> ()
      }
      frame "Add or Edit Metadata" {
        n1002 = local read "Result files to read"() -> (w1957:path[])
        n1003 = call "Edit_Channel_Panel.vi"("All Channel names"=w1953, "Result files to read"=w1957) -> ("New Values Out"=w1967:string[], "New Chs Out"=w1968:string[], "Cancelled"=w1963:bool, "Edit Raw Data Header Info Out"=w1961:bool, "Plotted rows only?"=w1966:bool, "ptUnderCursor"=w1950:bool, "Edit Raw data files?"=w1959:bool, "Raw data files in Orig Positions?"=w1958:bool, "Mode"=w1965:T10)  [unwired: 5 out]
        "Edit Raw Data Header Info" <- w1961
        n1004 = local write "Raw DF in Orig Pos?"(w1958) -> ()
        n1005 = local write "Edit Raw Data Files?"(w1959) -> ()
        n1006 = local write "Plotted rows only?"(w1966) -> ()
        n1007 = local write "Mode"(w1965) -> ()
        n1008 = local write "justCursorPt"(w1950) -> ()
        n1009 = Build Array(w1967) -> (w1969:string[][])
        n1010 = Array Size(array=w1968) -> (size(s)=w1964:i32)
        n1011 = Greater Than 0?(x=w1964) -> (x > 0?=w1962:bool)
        n1012 = Or(x=w1961, y=w1962) -> (x .or. y?=w1960:bool)
        n1013 = local write "Add /Edit metadata"(FALSE ("Add /Edit metadata")) -> ()
        n1014 = global write "Results_plotter_Global.vi" "New Values In"(w1969) -> ()
        n1015 = Compound Arithmetic op=AND(invert w1963, w1960) -> (w1949:bool)
        n1016 = global write "Results_plotter_Global.vi" "New Chs In"(w1968) -> ()
        n1017 = local write "reloadPending"(w1949) -> ()
        n1018 = Select(t="Full Res file manipulator", s=w1949, f="What to do next?") -> (s? t:f=w1954:string)
      }
      frame "Time to save setup?" {
        n1019 = stacked-sequence {
          seq-local: [w1978 _] -> [_ w2020]
          tunnel: [_ w2021] -> w1976
          tunnel: w1975 -> [w1979 _]
          tunnel: w1973 -> [_ _]
          frame #0 {
            n1020 = while {
              shift-right: [w2009] -> _
              shift-left: _ -> [w2007]
              shift-right: [w1996] -> _
              shift-left: _ -> [w2004]
              tunnel: [w1996] -> w1984
              tunnel: [w1995] -> w1983
              shift-right: [w1997] -> _
              shift-left: _ -> [w2003]
              tunnel: [w2001] -> w1980
              tunnel: w1979 -> [w1992]
              shift-right: [w1988] -> _
              shift-left: _ -> [w1989]
              stop <- FALSE continue-if-true
              n1021 = Get Date/Time In Seconds() -> (seconds since 1Jan1904=w2005:timestamp)
              n1022 = local read "Show Results Space Analysis"() -> (w1996:bool)
              n1023 = To Double Precision Float(number=w2005) -> (double precision float=w2008:dbl)
              n1024 = local read "Template Last Mod"() -> (w1988:timestamp)
              n1025 = Greater?(x=w1992, y=300) -> (0:w1987:bool)
              n1026 = Subtract(x=w2008, y=w2007) -> (x-y=w2010:dbl)
              n1027 = Greater?(x=w2010, y="Save Setup Interval (s)") -> (0:w1993:bool)
              n1028 = local read "Show Plot Space Analysis"() -> (w1997:bool)
              n1029 = And(x=w1993, y=w1987) -> (x .and. y?=w1990:bool)
              "Time to Save Setup?" <- w1990
              n1030 = Not Equal?(x=w1989, y=w1988) -> (x != y?=w1986:bool)
              n1031 = Not Equal?(x=w1997, y=w2003) -> (x != y?=w1998:bool)
              n1032 = Not Equal?(x=w1996, y=w2004) -> (x != y?=w1995:bool)
              n1033 = Compound Arithmetic op=OR(invert w1987, w1986) -> (w1985:bool)
              n1034 = case shown="True" w1990 {
                tunnel: [w2014 w2017] -> w2009
                tunnel: w2008 -> [w2012 w2017]
                tunnel: w2007 -> [w2011 _]
                tunnel: ["Update Template file log" "Save Setup"] -> w2000
                tunnel: w1985 -> [w2013 _]
                frame False {
                  n1035 = Select(t=w2012, s=w2013, f=w2011) -> (s? t:f=w2014:dbl)
                }
                frame True {
                }
              }
              n1036 = And(x=w1997, y=w1998) -> (x .and. y?=w2002:bool)
              n1037 = Select(t="Analyse Plot Space", s=w2002, f=w2000) -> (s? t:f=w2001:string)
            }
            n1038 = And(x=w1984, y=w1983) -> (x .and. y?=w1982:bool)
            n1039 = Select(t="What is present?", s=w1982, f=w1980) -> (s? t:f=w1978:string)
          }
          frame #1 {
            n1040 = local read "Template"() -> (w2018:path)
            n1041 = Empty String/Path?(string/path=w2018) -> (empty?=w2019:bool)
            n1042 = case shown="False" w2019 {
              tunnel: w2018 -> [w2028 _]
              tunnel: [w2025 w2029] -> w2021
              tunnel: w2020 -> [w2023 w2029]
              frame False {
                n1043 = local read "Template Last Mod"() -> (w2026:timestamp)
                n1044 = File/Directory Info(path=w2028) -> (last mod=w2027:timestamp)  [unwired: 1 in, 6 out]
                n1045 = Not Equal?(x=w2026, y=w2027) -> (x != y?=w2022:bool)
                "Template Changed?" <- w2022
                n1046 = Select(t="Save Setup", s=w2022, f=w2023) -> (s? t:f=w2025:string)
              }
              frame True {
              }
            }
          }
        }
      }
      frame "Update Template file log" {
        n1047 = local read "Template"() -> (w2032:path)
        n1048 = global read "Results_plotter_Global.vi" "Raw Data Filename index"() -> (w2030:i32)
        n1049 = feedback #1() -> (w2037:timestamp)  [unwired: 1 in]
        n1050 = File/Directory Info(path=w2032) -> (last mod=w2036:timestamp)  [unwired: 1 in, 6 out]
        n1051 = feedback-in #1(w2036) -> ()
        n1052 = feedback #2() -> (w2038:path)  [unwired: 1 in]
        n1053 = feedback-in #2(w2032) -> ()
        n1054 = Equal?(x=w2036, y=w2037) -> (x = y?=w2035:bool)
        n1055 = Equal?(x=w2032, y=w2038) -> (x = y?=w2034:bool)
        n1056 = And(x=w2034, y=w2035) -> (x .and. y?=w2033:bool)
        n1057 = case shown="False" w2033 {
          tunnel: w2032 -> [w2049 _]
          tunnel: w2031 -> [w2044 _]
          tunnel: w2030 -> [w2043 _]
          frame False {
            n1058 = Index Array(array=w2044, index (col)=w2043) -> (element=w2048:string[])  [unwired: 1 in]
            n1059 = for {
              tunnel: w2048 -> [w2061] mode=indexing
              tunnel: [w2060] -> w2047 mode=indexing
              n1060 = call "String_to_Pathname.vi"("Input String"=w2061) -> ("path"=w2059:path)
              n1061 = call "Get Raw Data Folder.vi"("Raw data file"=w2059) -> ("Main Raw Data Folder"=w2058:path)
              n1062 = for {
                N: 3 -> [_]
                shift-right: [w2064] -> w2060
                shift-left: w2058 -> [w2063]
                n1063 = Strip Path(path=w2063) -> (stripped path=w2064:path)  [unwired: 1 out]
              }
            }
            n1064 = for {
              tunnel: w2047 -> [w2050] mode=indexing
              shift-right: [w2051] -> w2045
              shift-left: path[] [] -> [w2052]
              n1065 = Search 1D Array(1D array=w2052, element=w2050) -> (index of element=w2053:i32)  [unwired: 1 in]
              n1066 = case shown="-1" w2053 {
                tunnel: w2050 -> [_ w2055]
                tunnel: w2052 -> [w2054 w2057]
                tunnel: [w2054 w2056] -> w2051
                frame 0, Default {
                }
                frame -1 {
                  n1067 = Build Array (concatenate)(w2057, w2055) -> (w2056:path[])
                }
              }
            }
            "RD_Folders" <- w2045
            n1068 = for {
              tunnel: w2045 -> [w2066] mode=indexing
              tunnel: w2049 -> [w2065]
              n1069 = Strip Path(path=w2065) -> (name=w2067:string)  [unwired: 1 out]
              n1070 = Build Path(base path=w2066, name or relative path="Logs") -> (appended path=w2073:path)
              n1071 = Build Path(base path=w2073, name or relative path="Results_File_Plotter_Templates") -> (appended path=w2068:path)
              n1072 = Build Path(base path=w2068, name or relative path="Current") -> (appended path=w2069:path)
              n1073 = Build Path(base path=w2069, name or relative path=w2067) -> (appended path=w2075:path)
              n1074 = call "Does_file_exist_(simple).vi"("Pathname"=w2075) -> ("exists?"=w2074:bool)
              n1075 = case shown="True" w2074 {
                tunnel: w2065 -> [w2079 w2085]
                tunnel: w2075 -> [w2077 w2086]
                tunnel: w2068 -> [_ w2088]
                tunnel: w2067 -> [_ w2087]
                frame False {
                  n1076 = Strip Path(path=w2077) -> (stripped path=w2078:path)  [unwired: 1 out]
                  n1077 = call <vilib>:"Create Directory Recursive.vi"("directory"=w2078) -> ("error out"=w2076:errorcluster)  [unwired: 4 in, 2 out]
                  n1078 = Copy(8:w2076, 10:w2077, 11:w2079) -> ()  [unwired: 2 in, 3 out]
                }
                frame True {
                  n1079 = File/Directory Info(path=w2086) -> (last mod=w2081:timestamp, error out=w2080:errorcluster)  [unwired: 1 in, 5 out]
                  n1080 = Unbundle By Name(w2080) -> ("status"=w2083:bool)
                  n1081 = File/Directory Info(path=w2085) -> (last mod=w2089:timestamp)  [unwired: 1 in, 6 out]
                  n1082 = Not Equal?(x=w2081, y=w2089) -> (x != y?=w2084:bool)
                  n1083 = Compound Arithmetic op=AND(invert w2083, w2084) -> (w2082:bool)
                  n1084 = case shown="True" w2082 {
                    tunnel: w2088 -> [_ w2101]
                    tunnel: w2087 -> [_ w2099]
                    tunnel: w2086 -> [_ w2093]
                    tunnel: w2085 -> [_ w2094]
                    tunnel: w2080 -> [_ w2090]
                    frame False {
                    }
                    frame True {
                      n1085 = Build Path(base path=w2101, name or relative path="History") -> (appended path=w2100:path)
                      n1086 = Build Path(base path=w2100, name or relative path=w2099) -> (appended path=w2098:path)
                      n1087 = Build Path(base path=w2098, name or relative path=w2099) -> (appended path=w2095:path)
                      n1088 = call "Does_file_exist_(simple).vi"("Pathname"=w2095) -> ("exists?"=w2097:bool)
                      n1089 = case shown="False" w2097 {
                        tunnel: [w2104 w2108] -> w2096
                        tunnel: w2095 -> [w2104 w2107]
                        tunnel: [w2103 w2106] -> w2091
                        tunnel: w2090 -> [_ w2106]
                        frame False {
                          n1090 = Strip Path(path=w2104) -> (stripped path=w2105:path)  [unwired: 1 out]
                          n1091 = call <vilib>:"Create Directory Recursive.vi"("directory"=w2105) -> ("error out"=w2103:errorcluster)  [unwired: 4 in, 2 out]
                        }
                        frame True {
                          n1092 = call "Find_Unique_Filename.vi"("Path In"=w2107, "Max Length (31)"=50) -> ("Unique Path Out"=w2108:path)  [unwired: 1 in]
                        }
                      }
                      n1093 = Move(source path=w2093, error in=w2091, 10:w2096) -> (error out=w2092:errorcluster)  [unwired: 2 in, 2 out]
                      n1094 = Copy(8:w2092, 10:w2093, 11:w2094) -> ()  [unwired: 2 in, 3 out]
                    }
                  }
                }
              }
            }
          }
          frame True {
          }
        }
      }
      frame "Check modification dates?" {
        n1095 = while {
          shift-right: [w2129] -> _
          shift-left: _ -> [w2127]
          tunnel: [w2126] -> w2119
          stop <- FALSE continue-if-true
          n1096 = Get Date/Time In Seconds() -> (seconds since 1Jan1904=w2124:timestamp)
          n1097 = To Double Precision Float(number=w2124) -> (double precision float=w2128:dbl)
          n1098 = Subtract(x=w2128, y=w2127) -> (x-y=w2131:dbl)
          n1099 = Greater?(x=w2131, y="Reload Interval (s)") -> (0:w2130:bool)
          n1100 = case shown="True" w2130 {
            tunnel: [w2133 w2136] -> w2129
            tunnel: w2128 -> [_ w2136]
            tunnel: w2127 -> [w2133 _]
            tunnel: [FALSE w2134] -> w2126
            frame False {
            }
            frame True {
              n1101 = global read "Results_plotter_Global.vi" "First Loop"() -> (w2135:bool)
              n1102 = Not(x=w2135) -> (.not. x?=w2134:bool)
            }
          }
        }
        n1103 = Equal?(x="Tab Control", y=enum32{"Load ", "Plot ", "Save ", "Cursor"}."Cursor" ("Tab Control")) -> (x = y?=w2115:bool)
        n1104 = Select(t="Read Cursor", s=w2115, f="Ordinate Selector Type") -> (s? t:f=w2113:string)
        n1105 = Select(t="Files Modified?", s=w2119, f=w2113) -> (s? t:f=w2118:string)
      }
      frame "Files Modified?" {
        n1106 = local read "nRows"() -> (w2137:i32)
        n1107 = Less?(x=w2137, y=w2141) -> (x < y?=w2139:bool)
        n1108 = case shown="True" w2139 {
          tunnel: [w2146 w2152] -> w2142
          tunnel: "Ordinate Selector Type" -> [w2146 w2147]
          frame False {
          }
          frame True {
            n1109 = local read "Result files to read"() -> (w2151:path[])
            n1110 = for {
              tunnel: w2151 -> [w2154] mode=indexing
              tunnel: [w2153] -> w2150 mode=indexing
              n1111 = call "File_Modified_Since_Check.vi"("File Path"=w2154) -> ("modifiedSinceCheck"=w2153:bool)  [unwired: 7 in, 1 out]
            }
            n1112 = Or Array Elements(Boolean array=w2150) -> (logical OR=w2149:bool)
            n1113 = Select(t="Initialise", s=w2149, f=w2147) -> (s? t:f=w2152:string)
          }
        }
      }
      frame "Read Cursor" {
        n1114 = global read "Plot_Values_Global.vi" "XY Graph Cluster"() -> (w2159:cluster{dbl[], dbl[]}[])
        n1115 = property on="XY Plot" class="XYGraph (strict)"() -> ("Cursor.Cursor X"=w2163:dbl, "Cursor.Cursor Y"=w2164:dbl)  [unwired: 2 in, 2 out]
        n1116 = local read "graphPaneTab"() -> (w2155:T7)
        n1117 = for {
          tunnel: w2163 -> [w2210]
          tunnel: w2164 -> [w2209]
          tunnel: [w2216] -> w2162 mode=concatenating
          tunnel: w2159 -> [w2215] mode=indexing
          workers-P: _ -> [_]
          n1118 = Unbundle(w2215) -> (w2208:dbl[], w2207:dbl[])
          n1119 = Subtract(x=w2210, y=w2208) -> (x-y=w2214:dbl[])
          n1120 = Subtract(x=w2209, y=w2207) -> (x-y=w2213:dbl[])
          n1121 = Square(x=w2214) -> (x^2=w2211:dbl[])
          n1122 = Square(x=w2213) -> (x^2=w2212:dbl[])
          n1123 = Add(x=w2211, y=w2212) -> (x+y=w2216:dbl[])
        }
        n1124 = global read "Results_plotter_Global.vi" "Plotted Row Numbers"() -> (w2160:i32[])
        n1125 = Array Max & Min(array=w2162) -> (min index (indices)=w2161:i32)  [unwired: 3 out]
        n1126 = Index Array(array=w2160, index=w2161) -> (element=w2157:i32)
        "Cursor index" <- w2157
        n1127 = Index Array(array=w2165, index (row)=w2157) -> (element=w2158:string[])  [unwired: 1 in]
        n1128 = for {
          tunnel: w2168 -> [w2192] mode=indexing
          tunnel: w2158 -> [w2185] mode=indexing
          tunnel: [w2191] -> w2156 mode=indexing
          n1129 = while {
            shift-right: [w2204] -> _
            shift-left: w2185 -> [w2205]
            tunnel: [w2201] -> w2189
            tunnel: [w2200] -> w2187 mode=indexing
            i -> [w2201]
            stop <- w2202 continue-if-true
            n1130 = Match Pattern(string=w2205, regular expression=":") -> (before substring=w2200:string, after substring=w2204:string, offset past match=w2203:i32)  [unwired: 2 out]
            n1131 = Greater Than 0?(x=w2203) -> (x > 0?=w2202:bool)
          }
          n1132 = Reverse 1D Array(array=w2187) -> (reversed array=w2186:string[])
          n1133 = Greater?(x=w2189, y=2) -> (0:w2188:bool)
          n1134 = case shown="False" w2188 {
            tunnel: w2192 -> [w2195 w2199]
            tunnel: [w2193 w2198] -> w2191
            tunnel: w2186 -> [_ w2197]
            tunnel: w2185 -> [w2194 w2196]
            frame False {
              n1135 = Build Array(w2195, w2194) -> (w2193:string[])
            }
            frame True {
              n1136 = Build Array (concatenate)(w2199, w2197, w2196) -> (w2198:string[])
            }
          }
        }
        "dataTable" <- w2156
        n1137 = case shown="\"XY\"" w2155 {
          tunnel: w2156 -> [w2178 _]
          frame "XY" {
            n1138 = case shown="\"Scrub\", Default" "picMode" {
              tunnel: [FALSE ("cursorDrag") w2183] -> w2179
              frame "Scrub", Default {
              }
              frame "Jump" {
                n1139 = local read "cursorDrag"() -> (w2183:bool)
              }
            }
            n1140 = Index Array(array=w2178, index (col) #1=0 ("disabled index (col)")) -> (element #1=w2177:string[], element #2=w2175:string[])  [unwired: 3 in]
            n1141 = Search 1D Array(1D array=w2177, element="Raw Data Filename") -> (index of element=w2174:i32)  [unwired: 1 in]
            n1142 = Index Array(array=w2175, index=w2174) -> (element=w2172:string)
            n1143 = call "String 2 Path memory.vi"("Input String"=w2172) -> ("path"=w2171:path)  [unwired: 1 in]
            n1144 = Compound Arithmetic op=AND("ShowPix", invert w2179) -> (w2180:bool)
            n1145 = case shown="True" w2180 {
              tunnel: w2171 -> [_ w2184]
              frame False {
              }
              frame True {
                n1146 = call "DigUpPixAsync.vi"("File Path"=w2184) -> ()  [unwired: 11 in]
              }
            }
          }
          frame "Contour", Default {
          }
        }
      }
      frame "Process Cursor Point" {
        n1147 = stacked-sequence {
          tunnel: ["What to do next?" ("t") _] -> w2222
          tunnel: w2219 -> [w2230 _]
          tunnel: w2218 -> [w2226 _]
          frame #0 {
            n1148 = local read "Cursor index"() -> (w2229:i32)
            n1149 = local read "Template"() -> (w2223:path)
            n1150 = local read "Result files to read"() -> (w2228:path[])
            n1151 = call "getRDfilepath.vi"("templatePath"=w2223, "rowIndex"=w2229, "Result files to read"=w2228) -> ("selectedRowNum"=w2225:i32, "rawDataPath"=w2227:path)  [unwired: 6 in, 1 out]
            "Selected Row" <- w2225
            n1152 = Index Array(array=w2226, index (row)=w2225) -> (element=w2224:string[])  [unwired: 1 in]
            n1153 = call "Post_Process_Measurement.vi"("Channel Values"=w2224, "Raw data file"=w2227, "Channel Names"=w2230) -> ()  [unwired: 3 in]
          }
          frame #1 {
            n1154 = case shown="True" "Choose\nPlug ins" {
              frame False {
              }
              frame True {
                n1155 = call "Plug_in_Directories.vi"() -> ("Per Block"=w2236:path)  [unwired: 2 in, 4 out]
                n1156 = List Folder(path=w2236) -> (filenames=w2234:string[])  [unwired: 3 in, 3 out]
                n1157 = local read "Per Block Plug Ins Extra"() -> (w2233:string[])
                n1158 = call "Select_Strings.vi"("Available Ch names"=w2234, "Message"="Please select the Desired Extras Per Block Plug Ins", "Selector mode"=T12."Zero or more", "Desired Ch names (in)"=w2233) -> ("Selected Channel Names"=w2237:string[])  [unwired: 2 in, 2 out]
                n1159 = local write "Per Block Plug Ins Extra"(w2237) -> ()
                n1160 = for {
                  tunnel: w2237 -> [w2251] mode=indexing
                  tunnel: w2236 -> [w2250]
                  n1161 = Build Path(base path=w2250, name or relative path=w2251) -> (appended path=w2252:path)
                  n1162 = Open VI Reference(vi path=w2252) -> (vi reference=w2247:refnum<vi>, error out=w2246:errorcluster)  [unwired: 1 in, 4 out]
                  n1163 = invoke class="VI" method="FP.Open"(reference=w2247, error in=w2246, "Activate"=FALSE ("Activate?"), "State"=T14."Standard") -> (reference out=w2245:refnum<vi>, error out=w2244:errorcluster)  [unwired: 1 in, 3 out]
                  n1164 = invoke class="VI" method="Run VI"(reference=w2245, error in=w2244, "Wait until done"=TRUE, "Auto Dispose Ref"=FALSE) -> (reference out=w2243:refnum<vi>, error out=w2242:errorcluster)  [unwired: 1 in, 3 out]
                  n1165 = Close Reference(reference=w2243, error in (no error)=w2242) -> ()  [unwired: 1 out]
                }
                n1166 = local write "Choose\nPlug ins"(FALSE ("Choose\nPlug ins")) -> ()
              }
            }
          }
        }
        n1167 = local write "Process Point"(FALSE ("Kill Point")) -> ()
      }
      frame "Kill Point" {
        # "Not now used- mark Killed points in Omit channel"
        n1168 = local read "Cursor index"() -> (w2265:i32)
        n1169 = local read "Template"() -> (w2253:path)
        n1170 = local read "Result files to read"() -> (w2264:path[])
        n1171 = call "getRDfilepath.vi"("templatePath"=w2253, "rowIndex"=w2265, "Result files to read"=w2264) -> ("selectedRowNum"=w2254:i32, "rawDataPath"=w2262:path, "Results file"=w2263:path)  [unwired: 6 in]
        n1172 = Strip Path(path=w2263) -> (name=w2256:string)  [unwired: 1 out]
        n1173 = Strip Path(path=w2262) -> (name=w2255:string)  [unwired: 1 out]
        n1174 = Format Into String(format string="Are you sure you want to remove the row in the results file \"%s\" generated from the raw data filename \"%s\"?", w2256, w2255) -> (resulting string=w2258:string)  [unwired: 2 in, 1 out]
        n1175 = Two Button Dialog(message=w2258) -> (T button?=w2257:bool)  [unwired: 2 out]
        n1176 = case shown="True" w2257 {
          tunnel: w2263 -> [_ w2271]
          tunnel: w2254 -> [_ w2270]
          frame False {
          }
          frame True {
            n1177 = Build Array(w2270) -> (w2272:i32[])
            n1178 = call "Delete_unwanted_rows.vi"("Selected Rows"=w2272, "Filename"=w2271) -> ()  [unwired: 1 out]
          }
        }
        n1179 = local write "Selected Row"(w2254) -> ()
        n1180 = local write "Kill Point"(FALSE ("Kill Point")) -> ()
      }
      frame "Edit template file" {
        n1181 = local read "Template"() -> (w2280:path)
        n1182 = local read "Result files to read"() -> (w2281:path[])
        n1183 = call "Valid_Path.vi"("Filename"=w2280) -> ("Valid Path?"=w2279:bool)
        n1184 = Select(t=T15."Edit Existing Template File" ("Mode"), s=w2279, f=T15."Create New Template File" ("Mode")) -> (s? t:f=w2277:T15)
        n1185 = call "Edit_Template_File.vi"("Mode"=w2277, "Template Filename"=w2280, "Data Files"=w2281) -> ("Cancelled"=w2275:bool, "Template Filename Out"=w2274:path)  [unwired: 11 out]
        n1186 = flat-sequence {
          tunnel: w2274 -> [_]
          frame #0 {
            n1187 = Current VI's Path() -> (path=w2288:path)
            n1188 = call "Open_Close_Front_Panel.ph.vi"("openWindow (T)"=TRUE ("Front Panel Window:Open"), "VI path"=w2288) -> ()  [unwired: 1 in, 1 out]
            n1189 = local write "Edit Template File"(FALSE ("Edit Template File")) -> ()
          }
        }
        n1190 = case shown="False" w2275 {
          tunnel: w2274 -> [w2289 _]
          tunnel: ["Initialise" "What to do next?"] -> w2273
          frame False {
            n1191 = local write "Template"(w2289) -> ()
            n1192 = File/Directory Info(path=w2289) -> (last mod=w2291:timestamp)  [unwired: 1 in, 6 out]
            n1193 = local write "Template Last Mod"(w2291) -> ()
            n1194 = global write "Results_plotter_Global.vi" "Template"(w2289) -> ()
          }
          frame True {
          }
        }
      }
      frame "Save Plot Data" {
        n1195 = global read "Plot_Values_Global.vi" "XY Graph Cluster"() -> (w2295:cluster{dbl[], dbl[]}[])
        n1196 = local read "Multi Ordinate"() -> (w2300:i32[])
        n1197 = local read "Tolerances"() -> (w2303:dbl[])
        n1198 = local read "Transpose"() -> (w2301:bool)
        n1199 = global read "Results_plotter_Global.vi" "Precision"() -> (w2297:string[])
        n1200 = local read "Absisca"() -> (w2302:u16)
        n1201 = stacked-sequence {
          seq-local: [w2314 _ _ _ _ _ _ _ _] -> [_ w2339 _ w2380 _ _ _ _ _]
          seq-local: [_ w2335 _ _ _ _ _ _ _] -> [_ _ _ _ _ _ _ w2503 _]
          seq-local: [_ _ _ _ _ w2432 _ _ _] -> [_ _ _ _ _ _ _ w2502 _]
          seq-local: [_ _ _ _ _ w2434 _ _ _] -> [_ _ _ _ _ _ w2470 _ _]
          seq-local: [_ _ _ w2378 _ _ _ _ _] -> [_ _ _ _ _ _ w2471 _ _]
          seq-local: [_ _ _ _ w2401 _ _ _ _] -> [_ _ _ _ _ w2428 _ _ _]
          seq-local: [w2311 _ _ _ _ _ _ _ _] -> [_ _ _ _ _ _ _ _ w2508]
          seq-local: [w2310 _ _ _ _ _ _ _ _] -> [_ w2327 _ _ _ _ _ _ _]
          seq-local: [_ _ w2360 _ _ _ _ _ _] -> [_ _ _ w2379 _ _ w2472 _ _]
          seq-local: [_ _ _ _ _ _ w2468 _ _] -> [_ _ _ _ _ _ _ w2500 _]
          tunnel: [_ _ _ _ _ _ _ _ w2506] -> w2306
          tunnel: w2305 -> [w2308 w2332 _ _ _ w2433 _ _ _]
          tunnel: [w2308 _ _ _ _ _ _ _ _] -> w2304
          tunnel: w2303 -> [w2316 _ _ _ w2406 w2431 _ _ _]
          tunnel: w2295 -> [w2315 _ _ w2382 _ _ _ _ _]
          tunnel: w2302 -> [w2313 w2349 _ _ w2408 _ _ _ _]
          tunnel: w2301 -> [w2312 _ _ w2381 _ _ _ _ _]
          tunnel: w2300 -> [_ _ _ _ w2405 _ _ _ _]
          tunnel: [w2309 _ _ _ _ _ _ _ _] -> w2299
          tunnel: w2298 -> [w2309 _ w2362 w2376 _ _ _ _ _]
          tunnel: w2297 -> [_ _ _ w2375 _ w2427 _ _ _]
          tunnel: w2296 -> [w2307 _ _ _ _ w2426 _ _ _]
          tunnel: [w2307 _ _ _ _ _ _ _ _] -> w2294
          frame #0 {
            n1202 = local read "Save Surface Fit"() -> (w2311:bool)
            n1203 = Not(x=w2312) -> (.not. x?=w2319:bool)
            n1204 = Index Array(array=w2316, index=w2313) -> (element=w2310:dbl)
            n1205 = for {
              tunnel: w2315 -> [w2326] mode=indexing
              tunnel: w2319 -> [w2323]
              shift-right: [w2321] -> w2317
              shift-left: dbl[] [] -> [w2322]
              n1206 = Unbundle(w2326) -> (w2325:dbl[], w2324:dbl[])
              n1207 = Select(t=w2325, s=w2323, f=w2324) -> (s? t:f=w2320:dbl[])
              n1208 = Build Array (concatenate)(w2322, w2320) -> (w2321:dbl[])
            }
            n1209 = call "Numeric_bins.vi"("Values"=w2317, "Tolerance"=w2310) -> ("Bin Centres"=w2314:dbl[])  [unwired: 2 out]
          }
          frame #1 {
            n1210 = Index Array(array=w2332, index=w2349) -> (element=w2352:string)
            n1211 = Match Pattern(string=w2352, regular expression=":") -> (before substring=w2351:string, after substring=w2350:string)  [unwired: 3 out]
            n1212 = Greater?(x=w2327, y=0.4) -> (0:w2347:bool)
            n1213 = Greater?(x=w2327, y=0.09) -> (0:w2342:bool)
            n1214 = Select(t=i16 0 ("precision (6)"), s=w2347, f=i16 2 ("precision (6)")) -> (s? t:f=w2343:i16)
            n1215 = Concatenate Strings(w2351, " ", w2350, " =:" ("regular expression")) -> (w2334:string)
            n1216 = Select(t=w2343, s=w2342, f=i16 3) -> (s? t:f=w2340:i16)
            n1217 = call <vilib>:"Trim Whitespace.vi"("string"=w2334) -> ("trimmed string"=w2333:string)  [unwired: 1 in]
            n1218 = Number To Fractional String(number=w2339, precision (6)=w2340) -> (F-format string=w2338:string[])  [unwired: 2 out]
            n1219 = for {
              tunnel: w2333 -> [w2355]
              tunnel: w2338 -> [w2353] mode=indexing
              tunnel: [w2354] -> w2337 mode=indexing
              n1220 = Concatenate Strings(w2355, w2353) -> (w2354:string)
            }
            n1221 = Build Array (concatenate)("Plot:Legend:" ("Input Element"), w2337, "End of:Plot Series:" ("Input Element")) -> (w2335:string[])
          }
          frame #2 {
            n1222 = local read "Multi Ordinate"() -> (w2359:i32[])
            n1223 = global read "Results_plotter_Global.vi" "Legend"() -> (w2361:string[])
            n1224 = Array Size(array=w2359) -> (size(s)=w2358:i32)
            n1225 = Greater?(x=w2358, y=1) -> (0:w2356:bool)
            n1226 = case shown="False" w2356 {
              tunnel: w2362 -> [w2367 _]
              tunnel: [w2364 w2374] -> w2360
              tunnel: w2361 -> [w2366 w2374]
              tunnel: w2359 -> [w2363 _]
              frame False {
                n1227 = Index Array(array=w2363, index=0 ("Index")) -> (element=w2368:i32)
                n1228 = Index Array(array=w2367, index=w2368) -> (element=w2365:string)
                n1229 = for {
                  tunnel: w2366 -> [w2373] mode=indexing
                  tunnel: w2365 -> [w2372]
                  tunnel: [w2370] -> w2364 mode=indexing
                  n1230 = Format Into String(format string="; %s", initial string=w2372, w2373) -> (resulting string=w2370:string)  [unwired: 1 in, 1 out]
                }
              }
              frame True {
              }
            }
          }
          frame #3 {
            n1231 = call "Grid_Data.vi"("Transpose"=w2381, "XY Graph"=w2382, "Bin Centres"=w2380) -> ("Grided data"=w2377:dbl[][])  [unwired: 1 out]
            n1232 = for {
              tunnel: w2379 -> [w2389] mode=indexing
              tunnel: [w2391] -> w2378 mode=indexing
              tunnel: w2377 -> [w2390] mode=indexing
              tunnel: w2376 -> [w2385]
              tunnel: w2375 -> [w2384]
              n1233 = Match Pattern(string=w2389, regular expression=";") -> (before substring=w2386:string)  [unwired: 4 out]
              n1234 = Search 1D Array(1D array=w2385, element=w2386) -> (index of element=w2387:i32)  [unwired: 1 out]
              n1235 = Index Array(array=w2384, index=w2387) -> (element=w2383:string)
              n1236 = for {
                tunnel: w2383 -> [w2396]
                tunnel: [w2395] -> w2392 mode=indexing
                tunnel: w2390 -> [w2393] mode=indexing
                n1237 = Not A Number/Path/Refnum?(number/path/refnum=w2393) -> (NaN/Path/Refnum?=w2394:bool)
                n1238 = case shown="False" w2394 {
                  tunnel: w2396 -> [w2399 _]
                  tunnel: [w2398 ""] -> w2395
                  tunnel: w2393 -> [w2397 _]
                  frame False {
                    n1239 = call "Number_2_string.vi"("precision"=w2399, "number"=w2397) -> ("String"=w2398:string)
                  }
                  frame True {
                  }
                }
              }
              n1240 = Build Array (concatenate)(w2389, w2392) -> (w2391:string[])
            }
          }
          frame #4 {
            n1241 = global read "Results_plotter_Global.vi" "Summarise"() -> (w2402:string[])
            n1242 = Index Array(array=w2405, index=0 ("Index")) -> (element=w2403:i32)
            n1243 = for {
              shift-right: [w2417] -> w2401
              shift-left: i32[] [] -> [w2418]
              tunnel: w2408 -> [w2421]
              tunnel: w2403 -> [w2420]
              tunnel: w2406 -> [w2415] mode=indexing
              tunnel: w2402 -> [w2414] mode=indexing
              i -> [w2416]
              n1244 = Equal?(x=w2420, y=w2416) -> (x = y?=w2409:bool)
              n1245 = Not A Number/Path/Refnum?(number/path/refnum=w2415) -> (NaN/Path/Refnum?=w2411:bool)
              n1246 = Equal?(x=w2421, y=w2416) -> (x = y?=w2410:bool)
              n1247 = Equal?(x="FALSE", y=w2414) -> (x = y?=w2412:bool)
              n1248 = Compound Arithmetic op=OR(w2411, w2410, w2409, w2412) -> (w2419:bool)
              n1249 = case shown="False" w2419 {
                tunnel: w2418 -> [w2424 w2425]
                tunnel: [w2423 w2425] -> w2417
                tunnel: w2416 -> [w2422 _]
                frame False {
                  n1250 = Build Array (concatenate)(w2424, w2422) -> (w2423:i32[])
                }
                frame True {
                }
              }
            }
          }
          frame #5 {
            n1251 = local read "Plotted Series"() -> (w2430:bool[][])
            n1252 = for {
              tunnel: w2431 -> [w2445]
              tunnel: [w2444] -> w2434 mode=indexing
              tunnel: w2428 -> [w2443]
              tunnel: w2426 -> [w2442]
              tunnel: w2430 -> [w2441] mode=indexing
              tunnel: i32[] [] -> [w2439]
              tunnel: w2427 -> [w2438]
              n1253 = for {
                shift-right: [w2447] -> w2440
                shift-left: w2439 -> [w2448]
                tunnel: w2441 -> [w2446] mode=indexing
                i -> [w2449]
                n1254 = case shown="True" w2446 {
                  tunnel: w2449 -> [_ w2453]
                  tunnel: w2448 -> [w2450 w2452]
                  tunnel: [w2450 w2451] -> w2447
                  frame False {
                  }
                  frame True {
                    n1255 = Build Array (concatenate)(w2452, w2453) -> (w2451:i32[])
                  }
                }
              }
              n1256 = for {
                tunnel: w2445 -> [w2461]
                tunnel: [w2462] -> w2444 mode=indexing
                tunnel: w2443 -> [w2456] mode=indexing
                tunnel: w2442 -> [w2459]
                tunnel: w2440 -> [w2458]
                tunnel: w2438 -> [w2455]
                n1257 = for {
                  tunnel: w2458 -> [w2467] mode=indexing
                  tunnel: [w2466] -> w2463 mode=indexing
                  tunnel: w2456 -> [w2465]
                  tunnel: w2459 -> [w2464]
                  n1258 = Index Array(array=w2464, index (row)=w2467, index (col)=w2465) -> (element=w2466:string)
                }
                n1259 = Index Array(array=w2455, index=w2456) -> (element=w2457:string)
                n1260 = Index Array(array=w2461, index=w2456) -> (element=w2460:dbl)
                n1261 = call "Value_Occurence_Analysis.vi"("Average Numeric Values?"=FALSE, "Tolerance"=w2460, "Precision (3)"=w2457, "String Array"=w2463) -> ("Output String"=w2462:string)  [unwired: 2 out]
              }
            }
            n1262 = for {
              tunnel: w2428 -> [w2437] mode=indexing
              tunnel: w2433 -> [w2436]
              tunnel: [w2435] -> w2432 mode=indexing
              n1263 = Index Array(array=w2436, index=w2437) -> (element=w2435:string)
            }
          }
          frame #6 {
            n1264 = for {
              shift-right: [w2486] -> w2468
              shift-left: string[][] [] -> [w2487]
              shift-right: [w2482] -> _
              shift-left: _ -> [w2483]
              tunnel: w2472 -> [w2484] mode=indexing
              tunnel: w2471 -> [w2476] mode=indexing
              tunnel: w2470 -> [w2475] mode=indexing
              i -> [w2481]
              n1265 = Build Array (concatenate)(w2476, "", w2475) -> (w2474:string[])
              n1266 = Match Pattern(string=w2484, regular expression="; ") -> (before substring=w2482:string)  [unwired: 4 out]
              n1267 = Equal?(x=w2483, y=w2482) -> (x = y?=w2479:bool)
              n1268 = Greater Than 0?(x=w2481) -> (x > 0?=w2480:bool)
              n1269 = Compound Arithmetic op=AND(w2480, invert w2479) -> (w2478:bool)
              n1270 = case shown="False" w2478 {
                tunnel: w2487 -> [w2491 w2494]
                tunnel: [w2490 w2493] -> w2486
                tunnel: w2474 -> [w2489 w2492]
                tunnel: string[] [] ("array") -> [w2488 _]
                frame True {
                  n1271 = Build Array (concatenate)(w2491, w2488, w2489) -> (w2490:string[][])
                }
                frame False {
                  n1272 = Build Array (concatenate)(w2494, w2492) -> (w2493:string[][])
                }
              }
            }
          }
          frame #7 {
            w2499 = TRUE  # Simple Save?
            n1273 = Build Array (concatenate)(w2503, w2502) -> (w2501:string[])
            n1274 = local read "Header"() -> (w2496:string)
            n1275 = call "Write_output_file.vi"("Output filename"="Output Filename", "Header"=w2496, "Channel Names"=w2501, "Data"=w2500, "Simple Save?"=w2499, "Summarise mode"=T16."No data summary") -> ("Output filename Out"=w2497:path)  [unwired: 6 in, 3 out]
            n1276 = local write "Output Filename"(w2497) -> ()
          }
          frame #8 {
            n1277 = local write "Header"("") -> ()
            n1278 = local write "Save Plot data"(FALSE ("Save Plot data")) -> ()
            n1279 = Select(t="Save Surface Fit data", s=w2508, f="Create Selectors") -> (s? t:f=w2506:string)
          }
        }
      }
      frame "What type of row averaging?" {
        n1280 = Two Button Dialog(message="Do you want to Combine rows with identical positions together?", 1:"Average Points in Series" ("F button name (\"Cancel\")"), 2:"Combine rows" ("T button name (\"OK\")")) -> (T button?=w2514:bool)
        n1281 = Select(t="Combine rows" ("T button name (\"OK\")"), s=w2514, f="Average Rows together") -> (s? t:f=w2511:string)
      }
      frame "Combine rows" {
        w2528 = TRUE  # Show panel ?
        n1282 = local read "Output Filename"() -> (w2527:path)
        n1283 = call "Combined_file_Panel.vi"("Show panel ?"=w2528, "Output filename"=w2527) -> ("Only Plotted data?"=w2529:bool, "Include Empty Rows? Out"=w2530:bool, "Give Audit Channels Out"=w2531:bool, "Output filename Out"=w2526:path)  [unwired: 5 out]
        n1284 = case shown="True" w2529 {
          tunnel: w2525 -> [w2538 w2541]
          tunnel: [w2538 w2540] -> w2532
          frame False {
          }
          frame True {
            n1285 = global read "Results_plotter_Global.vi" "Plotted Row Numbers"() -> (w2539:i32[])
            n1286 = for {
              tunnel: w2541 -> [w2544]
              tunnel: [w2543] -> w2540 mode=indexing
              tunnel: w2539 -> [w2542] mode=indexing
              n1287 = Index Array(array=w2544, index (row)=w2542) -> (element=w2543:string[])  [unwired: 1 in]
            }
          }
        }
        n1288 = global read "Results_plotter_Global.vi" "3D Ch Selectors"() -> (w2523:i32[])
        n1289 = local write "Save Averaged rows"(FALSE ("Save Plot data")) -> ()
        n1290 = Index Array(array=w2523) -> (element #1=w2524:i32, element #2=w2522:i32, element #3=w2521:i32)  [unwired: 3 in]
        n1291 = call "Find_Rows_to_Combine.vi"("Include Empty Rows?"=w2530, "file path (dialog if empty)"=w2526, "Give Audit Channels"=w2531, "Full Channel Names"=w2535, "Data"=w2532, "Z Column Index"=w2521, "Y Column Index"=w2522, "X Column Index"=w2524) -> ()  [unwired: 4 out]
        n1292 = local write "Output Filename"(w2526) -> ()
      }
      frame "Average Rows together" {
        n1293 = global read "Plot_Values_Global.vi" "XY Graph Cluster"() -> (w2547:cluster{dbl[], dbl[]}[])
        n1294 = global read "Results_plotter_Global.vi" "Summarise"() -> (w2552:string[])
        n1295 = local read "Tolerances"() -> (w2550:dbl[])
        n1296 = local read "Transpose"() -> (w2554:bool)
        n1297 = local read "Absisca"() -> (w2549:u16)
        n1298 = stacked-sequence {
          seq-local: [_ w2578 _ _] -> [_ _ w2601 _]
          seq-local: [w2561 _ _ _] -> [_ _ w2600 _]
          tunnel: [_ _ _ "Create Selectors"] -> w2557
          tunnel: w2556 -> [w2559 _ _ _]
          tunnel: [w2559 _ _ _] -> w2555
          tunnel: w2547 -> [_ w2582 _ _]
          tunnel: w2554 -> [_ w2581 _ _]
          tunnel: w2553 -> [w2560 _ _ _]
          tunnel: w2552 -> [w2562 _ _ _]
          tunnel: [w2560 _ _ _] -> w2551
          tunnel: w2550 -> [_ w2580 _ _]
          tunnel: w2549 -> [_ w2579 _ _]
          tunnel: w2548 -> [w2558 w2575 _ _]
          tunnel: [w2558 _ _ _] -> w2545
          frame #0 {
            n1299 = for {
              tunnel: w2562 -> [w2567] mode=indexing
              shift-right: [w2563] -> w2561
              shift-left: w2559 -> [w2564]
              tunnel: w2559 -> [w2565] mode=indexing
              n1300 = Equal?(x="TRUE", y=w2567) -> (x = y?=w2566:bool)
              n1301 = case shown="False" w2566 {
                tunnel: w2565 -> [w2573 _]
                tunnel: w2564 -> [w2570 w2574]
                tunnel: [w2569 w2574] -> w2563
                frame False {
                  n1302 = Concatenate Strings(w2573, "St Dev") -> (w2571:string)
                  n1303 = Build Array (concatenate)(w2570, w2571) -> (w2569:string[])
                }
                frame True {
                }
              }
            }
          }
          frame #1 {
            n1304 = Not(x=w2581) -> (.not. x?=w2583:bool)
            n1305 = global read "Results_plotter_Global.vi" "Plotted Row Numbers"() -> (w2576:i32[])
            n1306 = for {
              tunnel: w2582 -> [w2597] mode=indexing
              tunnel: w2583 -> [w2594]
              tunnel: w2575 -> [w2593]
              tunnel: w2580 -> [w2592]
              tunnel: w2579 -> [w2591]
              tunnel: [w2590] -> w2578 mode=concatenating
              shift-right: [w2587] -> _
              shift-left: 0 -> [w2585]
              tunnel: w2576 -> [w2589]
              n1307 = Unbundle(w2597) -> (w2596:dbl[], w2595:dbl[])
              n1308 = Select(t=w2596, s=w2594, f=w2595) -> (s? t:f=w2588:dbl[])
              n1309 = Array Subset(array=w2589, index=w2585) -> (w2584:i32[])  [unwired: 1 in]
              n1310 = Array Size(array=w2588) -> (size(s)=w2586:i32)
              n1311 = call "Produce_averaged_Rows.vi"("Absisca"=w2591, "Row numbers"=w2584, "Tolerances"=w2592, "Array in"=w2588, "Data"=w2593) -> ("Array out"=w2590:string[][])  [unwired: 6 in]
              n1312 = Add(x=w2586, y=w2585) -> (x+y=w2587:i32)
            }
          }
          frame #2 {
            n1313 = local read "Output Filename"() -> (w2599:path)
            n1314 = call "Does_file_exist_(simple).vi"("Pathname"=w2599) -> ("exists?"=w2598:bool)
            n1315 = case shown="True" w2598 {
              tunnel: w2601 -> [w2604 w2612]
              tunnel: w2600 -> [w2607 w2613]
              tunnel: w2599 -> [w2605 w2614]
              frame False {
                w2608 = FALSE  # Save Plotted rows only?
                w2610 = TRUE  # Simple Save?
                n1316 = Build Array (concatenate)(string[] [] ("array"), w2604) -> (w2603:string[][])
                n1317 = local read "Template"() -> (w2609:path)
                n1318 = call "Write_output_file.vi"("Output filename"=w2605, "Template Filename"=w2609, "Channel Names"=w2607, "Data"=w2603, "Simple Save?"=w2610, "Save Plotted rows only?"=w2608, "Summarise mode"=T16."No data summary") -> ("Output filename Out"=w2611:path)  [unwired: 5 in, 3 out]
                n1319 = local write "Output Filename"(w2611) -> ()
              }
              frame True {
                w2617 = FALSE  # Present Channels only
                w2619 = TRUE  # exists?
                n1320 = call "Check_and_rewrite_file.vi"("Filename"=w2614, "Present Channels only"=w2617, "Present Channels"=w2613) -> ("Merged Channels"=w2618:string[], "Merged?"=w2616:bool)  [unwired: 1 in, 10 out]
                n1321 = case shown="True" w2616 {
                  tunnel: w2612 -> [w2620 w2622]
                  tunnel: w2613 -> [_ w2623]
                  tunnel: [w2620 w2621] -> w2615
                  tunnel: w2618 -> [_ w2624]
                  frame False {
                  }
                  frame True {
                    n1322 = call "Merge_2D_values.vi"("Values In"=w2622, "Present Channels"=w2623, "Desired Channels"=w2624) -> ("Values Out"=w2621:string[][])
                  }
                }
                n1323 = call "Write_Ch_data_file.vi"("exists?"=w2619, "Channel Values"=w2615, "Channel names"=w2618, "Filename"=w2614) -> ()  [unwired: 4 in, 4 out]
              }
            }
          }
          frame #3 {
            n1324 = local write "Save Averaged rows"(FALSE ("Save Plot data")) -> ()
          }
        }
      }
      frame "Save Surface Fit data" {
        n1325 = local read "Tolerances"() -> (w2636:dbl[])
        n1326 = local read "Transpose"() -> (w2630:bool)
        n1327 = global read "Results_plotter_Global.vi" "Precision"() -> (w2632:string[])
        n1328 = local read "Absisca"() -> (w2635:u16)
        n1329 = stacked-sequence {
          seq-local: [w2644 _ _ _ _ _] -> [_ w2663 _ _ _ _]
          seq-local: [_ w2660 _ _ _ _] -> [_ _ _ _ w2745 _]
          seq-local: [_ _ w2686 _ _ _] -> [_ _ _ _ w2764 _]
          seq-local: [w2645 _ _ _ _ _] -> [_ _ w2687 _ _ _]
          seq-local: [_ _ w2682 _ _ _] -> [_ _ _ _ w2748 _]
          seq-local: [_ _ w2681 _ _ _] -> [_ _ _ w2717 _ _]
          seq-local: [_ _ _ w2712 _ _] -> [_ _ _ _ w2746 _]
          tunnel: [_ _ _ _ _ "Create Selectors"] -> w2638
          tunnel: w2637 -> [w2640 w2648 _ _ _ _]
          tunnel: w2636 -> [_ w2674 _ _ _ _]
          tunnel: w2635 -> [_ w2675 _ _ _ _]
          tunnel: [w2641 _ _ _ _ _] -> w2634
          tunnel: w2633 -> [w2641 w2651 w2692 _ _ _]
          tunnel: w2632 -> [_ _ w2688 _ _ _]
          tunnel: [w2640 _ _ _ _ _] -> w2631
          tunnel: w2630 -> [_ _ _ w2711 _ _]
          tunnel: [w2639 _ _ _ _ _] -> w2628
          tunnel: w2629 -> [w2639 _ _ _ _ _]
          frame #0 {
            n1330 = global read "Results_plotter_Global.vi" "Raw Interpolation"() -> (w2642:dbl[][])
            n1331 = global read "Results_plotter_Global.vi" "X Values"() -> (w2644:dbl[])
            n1332 = global read "Results_plotter_Global.vi" "Y Values"() -> (w2643:dbl[])
            n1333 = Insert Into Array(array=w2642, index (col)=0 ("disabled index (col)"), new element=w2643) -> (w2645:dbl[][])  [unwired: 1 in]
          }
          frame #1 {
            n1334 = global read "Results_plotter_Global.vi" "Y Axis Name"() -> (w2650:string)
            n1335 = Index Array(array=w2674, index=w2675) -> (element=w2665:dbl)
            n1336 = Greater?(x=w2665, y=0.9) -> (0:w2672:bool)
            n1337 = Greater?(x=w2665, y=0.09) -> (0:w2667:bool)
            n1338 = Search 1D Array(1D array=w2651, element=w2650) -> (index of element=w2649:i32)  [unwired: 1 out]
            n1339 = Select(t=i16 0 ("precision (6)"), s=w2672, f=i16 2 ("precision (6)")) -> (s? t:f=w2668:i16)
            n1340 = Index Array(array=w2648, index=w2649) -> (element=w2647:string)
            n1341 = Select(t=w2668, s=w2667, f=i16 3) -> (s? t:f=w2664:i16)
            n1342 = Number To Fractional String(number=w2663, precision (6)=w2664) -> (F-format string=w2662:string[])  [unwired: 2 out]
            n1343 = Match Pattern(string=w2647, regular expression=":") -> (before substring=w2677:string, after substring=w2676:string)  [unwired: 3 out]
            n1344 = Concatenate Strings(w2677, " ", w2676, " =:" ("regular expression")) -> (w2659:string)
            n1345 = call <vilib>:"Trim Whitespace.vi"("string"=w2659) -> ("trimmed string"=w2658:string)  [unwired: 1 in]
            n1346 = for {
              tunnel: w2658 -> [w2680]
              tunnel: w2662 -> [w2678] mode=indexing
              tunnel: [w2679] -> w2653 mode=indexing
              n1347 = Concatenate Strings(w2680, w2678) -> (w2679:string)
            }
            n1348 = Build Array (concatenate)("Channel:Values:Plotted" ("Input Element"), "Axis:Name:" ("Input Element"), "Axis:Values:" ("Input Element"), w2653) -> (w2660:string[])
          }
          frame #2 {
            n1349 = local read "Multi Ordinate"() -> (w2691:i32[])
            n1350 = Index Array(array=w2691, index=0 ("Index")) -> (element=w2689:i32)
            n1351 = Index Array(array=w2692, index=w2689) -> (element=w2682:string)
            n1352 = Index Array(array=w2688, index=w2689) -> (element=w2681:string)
            n1353 = global read "Results_plotter_Global.vi" "X Axis Name"() -> (w2685:string)
            n1354 = Concatenate Strings(w2685, " =" ("string")) -> (w2683:string)
            n1355 = for {
              tunnel: w2682 -> [w2694]
              tunnel: [w2697] -> w2686 mode=indexing
              tunnel: w2681 -> [w2696]
              tunnel: w2687 -> [w2695] mode=indexing
              tunnel: w2683 -> [w2693]
              n1356 = for {
                tunnel: w2695 -> [w2700] mode=indexing
                tunnel: [w2699] -> w2698 mode=indexing
                tunnel: w2696 -> [w2702]
                n1357 = Not A Number/Path/Refnum?(number/path/refnum=w2700) -> (NaN/Path/Refnum?=w2701:bool)
                n1358 = case shown="False" w2701 {
                  tunnel: w2702 -> [w2705 _]
                  tunnel: w2700 -> [w2704 _]
                  tunnel: [w2703 ""] -> w2699
                  frame False {
                    n1359 = call "Number_2_string.vi"("precision"=w2705, "number"=w2704) -> ("String"=w2703:string)
                  }
                  frame True {
                  }
                }
              }
              n1360 = Build Array (concatenate)(w2694, w2693, w2698) -> (w2697:string[])
            }
          }
          frame #3 {
            w2716 = "\t"
            n1361 = global read "Results_plotter_Global.vi" "X Axis Name"() -> (w2709:string)
            n1362 = global read "Results_plotter_Global.vi" "Y Axis Name"() -> (w2708:string)
            n1363 = global read "Results_plotter_Global.vi" "Value plotted Name"() -> (w2715:string)
            n1364 = global read "Results_plotter_Global.vi" "Intensity Plot data in rows"() -> (w2718:dbl[][])
            n1365 = case shown="False" w2711 {
              tunnel: [w2719 w2722] -> w2710
              tunnel: w2709 -> [w2720 w2722]
              tunnel: w2708 -> [w2719 w2721]
              tunnel: [w2720 w2721] -> w2707
              frame False {
              }
              frame True {
              }
            }
            n1366 = Concatenate Strings(w2710, w2716, w2707, w2716, w2715, "\n") -> (w2713:string)
            n1367 = for {
              tunnel: w2718 -> [w2728] mode=indexing
              tunnel: w2717 -> [w2731]
              shift-right: [w2727] -> w2712
              shift-left: w2713 -> [w2730]
              n1368 = Index Array(array=w2728, index #1=0 ("index")) -> (element #1=w2725:dbl, element #2=w2724:dbl, element #3=w2723:dbl)  [unwired: 2 in]
              n1369 = Not A Number/Path/Refnum?(number/path/refnum=w2723) -> (NaN/Path/Refnum?=w2726:bool)
              n1370 = case shown="False" w2726 {
                tunnel: w2731 -> [w2742 _]
                tunnel: w2730 -> [w2741 w2743]
                tunnel: w2723 -> [w2740 _]
                tunnel: [w2739 w2743] -> w2727
                tunnel: w2725 -> [w2738 _]
                tunnel: w2724 -> [w2737 _]
                frame False {
                  w2733 = "\t"
                  n1371 = call "Number_2_string.vi"("number"=w2738) -> ("String"=w2736:string)  [unwired: 1 in]
                  n1372 = call "Number_2_string.vi"("number"=w2737) -> ("String"=w2735:string)  [unwired: 1 in]
                  n1373 = call "Number_2_string.vi"("precision"=w2742, "number"=w2740) -> ("String"=w2734:string)
                  n1374 = Concatenate Strings(w2741, w2736, w2733, w2735, w2733, w2734, "\n") -> (w2739:string)
                }
                frame True {
                }
              }
            }
          }
          frame #4 {
            w2760 = TRUE  # append to file? (new file:F)
            n1375 = global read "Results_plotter_Global.vi" "Surface Integral"() -> (w2759:dbl)
            n1376 = global read "Results_plotter_Global.vi" "Surface Area"() -> (w2758:dbl)
            n1377 = Divide(x=w2759, y=w2758) -> (x/y=w2757:dbl)
            n1378 = call "Value_to_string.vi"("Value"=w2759, "Label for value"="Surface Integral") -> ("Output string"=w2754:string)  [unwired: 1 in]
            n1379 = call "Value_to_string.vi"("Value"=w2757, "Label for value"="Surface Average") -> ("Output string"=w2753:string)  [unwired: 1 in]
            n1380 = call "Value_to_string.vi"("Value"=w2758, "Label for value"="Surface Area") -> ("Output string"=w2755:string)  [unwired: 1 in]
            n1381 = Concatenate Strings(w2755, w2754, w2753) -> (w2750:string)
            n1382 = Initialize Array("", 10 ("Dimension Size")) -> (w2769:string[])
            n1383 = call "Asterisk_header.vi"("Channel names"=w2769) -> ("Header string"=w2747:string)
            n1384 = call "Ch_names_to_rows.vi"("Channel Names"=w2745) -> ("3 Row names"=w2744:string[][])
            n1385 = local read "Output Filename"() -> (w2761:path)
            n1386 = Build Array (concatenate)(w2744, w2764) -> (w2762:string[][])
            n1387 = Array To Spreadsheet String(array=w2762, 3:"%s" ("format string")) -> (spreadsheet string=w2749:string)  [unwired: 1 out]
            n1388 = Format Into String(format string="\n%s\n\n%s\n%s\n\n\nInterpolated Surface of %s\n%s\n%s\n%s\n\n\n%s", w2747, w2746, w2747, w2748, w2747, w2749, w2747, w2750) -> (resulting string=w2752:string)  [unwired: 2 in, 1 out]
            n1389 = call "Write_Characters_To_File.vi"("file path (dialog if empty)"=w2761, "character string"=w2752, "append to file? (new file:F)"=w2760) -> ()  [unwired: 2 in, 4 out]
          }
          frame #5 {
            n1390 = local write "Save Surface Fit"(FALSE ("Save Plot data")) -> ()
          }
        }
      }
      frame "Save Data in Rows" {
        w2784 = TRUE  # Show panel ?
        n1391 = local read "Output Filename"() -> (w2772:path)
        n1392 = call "Output_file_Panel.vi"("Output filename"=w2772, "Header"="Header", "Channel Names"=w2781, "Show panel ?"=w2784) -> ("Cancelled"=w2773:bool, "Save Full Res Data?"=w2774:bool, "Output filename Out"=w2787:path, "Header Out"=w2783:string, "Desired Columns"=w2785:i32[], "Summarise mode"=w2782:T16, "Grouping info"=w2778:T27[], "Channels to Tabulate in header Out"=w2776:i32[], "Save Plotted rows only?"=w2775:bool)  [unwired: 3 in]
        n1393 = case shown="False" w2773 {
          tunnel: w2787 -> [w2802 _]
          tunnel: w2785 -> [w2801 _]
          tunnel: w2783 -> [w2800 _]
          tunnel: w2782 -> [w2799 _]
          tunnel: w2781 -> [w2798 _]
          tunnel: [w2797 w2820] -> w2780
          tunnel: [w2796 "Create Selectors"] -> w2779
          tunnel: w2778 -> [w2795 _]
          tunnel: w2777 -> [w2794 _]
          tunnel: w2776 -> [w2793 _]
          tunnel: w2775 -> [w2792 _]
          tunnel: w2774 -> [w2791 _]
          tunnel: w2772 -> [_ w2820]
          frame False {
            n1394 = case shown="False" w2791 {
              tunnel: w2802 -> [w2815 w2817]
              tunnel: w2801 -> [w2814 _]
              tunnel: w2800 -> [w2813 _]
              tunnel: w2792 -> [w2812 _]
              tunnel: w2799 -> [w2811 _]
              tunnel: w2798 -> [w2810 _]
              tunnel: [w2809 w2817] -> w2797
              tunnel: ["Create Selectors" "Is Filename Empty?"] -> w2796
              tunnel: w2793 -> [w2804 _]
              tunnel: w2795 -> [w2803 _]
              tunnel: w2794 -> [w2805 _]
              frame False {
                w2807 = FALSE  # Simple Save?
                n1395 = local read "Template"() -> (w2808:path)
                n1396 = call "Write_output_file.vi"("Output filename"=w2815, "Header"=w2813, "Template Filename"=w2808, "Channel Names"=w2810, "Data"=w2805, "Desired Columns"=w2814, "Simple Save?"=w2807, "Save Plotted rows only?"=w2812, "Summarise mode"=w2811, "Grouping info"=w2803, "Channels to Tabulate in header"=w2804) -> ("Output filename Out"=w2809:path)  [unwired: 1 in, 3 out]
              }
              frame True {
                "Mode" <- Plotter_Mode."Save file" ("Mode")
              }
            }
            "Plotted rows only?" <- w2792
          }
          frame True {
            # "User punted from Output Panel"
          }
        }
        n1397 = local write "Save Data in Rows"(FALSE ("Save All data")) -> ()
        n1398 = local write "Output Filename"(w2780) -> ()
      }
      frame "Is Filename Empty?" {
        n1399 = call "File Dialog"("start path"="Full_Res_Results_Folder", "prompt"="Please select a new or existing folder to save the results files in") -> ("selected path"=w2827:path, "cancelled"=w2821:bool)  [unwired: 5 in, 7 out]
        n1400 = local write "Full_Res_Results_Folder"(w2827) -> ()
        n1401 = Select(t="Create Selectors", s=w2821, f="Full Res file manipulator") -> (s? t:f=w2822:string)
      }
      frame "Check for overwrite or append" {
        n1402 = local read "Output Filename"() -> (w2840:path)
        n1403 = Format Into String(format string="Do you want to append to the result file\n\"%s\"" ("message"), w2840) -> (resulting string=w2835:string)  [unwired: 2 in, 1 out]
        n1404 = call <vilib>:"Three Button Dialog.vi"("Window Title (\"\")"="Output File Dialog" ("Window Title (\"\")"), "Right Button Text (\"Cancel\")"="Cancel" ("Button 3 Name"), "Center Button Text (\"No\")"="Overwrite" ("F button name (\"Cancel\")"), "Left Button Text (\"Yes\")"="Append" ("T button name (\"OK\")"), "message"=w2835) -> ("Which Button?"=w2834:T19)  [unwired: 6 out]
        n1405 = case shown="\"Right Button\", Default" w2834 {
          tunnel: w2840 -> [_ w2846 _]
          tunnel: ["Full Res file manipulator" "Full Res file manipulator" "Create Selectors" ("t")] -> w2833
          frame "Left Button" {
          }
          frame "Center Button" {
            n1406 = call "Delete_with_Check.vi"("FilePath"=w2846) -> ()  [unwired: 1 out]
          }
          frame "Right Button", Default {
          }
        }
      }
      frame "Create Plot summary" {
        w2852 = i32[] []
        w2864 = TRUE  # Summarise All
        n1407 = global read "Results_plotter_Global.vi" "Row Reference"() -> (w2859:i32[][])
        n1408 = global read "Results_plotter_Global.vi" "Plotted Row Numbers"() -> (w2850:i32[])
        n1409 = Index Array(array=w2859, index (col)=0 ("disabled index (col)")) -> (element=w2858:i32[])  [unwired: 1 in]
        n1410 = for {
          tunnel: w2849 -> [w2885]
          tunnel: [w2884] -> w2865 mode=indexing if=w2875
          tunnel: w2850 -> [w2874] mode=indexing
          tunnel: w2858 -> [w2883]
          shift-right: [w2880] -> w2857
          shift-left: w2852 -> [w2881]
          shift-right: [w2877] -> _
          shift-left: w2852 -> [w2876]
          n1411 = Index Array(array=w2883, index=w2874) -> (element=w2879:i32)
          n1412 = Index Array(array=w2885, index (row)=w2874) -> (element=w2884:string[])  [unwired: 1 in]
          n1413 = Search 1D Array(1D array=w2876, element=w2874) -> (index of element=w2878:i32)  [unwired: 1 out]
          n1414 = Search 1D Array(1D array=w2881, element=w2879) -> (index of element=w2882:i32)  [unwired: 1 out]
          n1415 = case shown="-1" w2878 {
            tunnel: w2874 -> [_ w2891]
            tunnel: w2876 -> [w2887 w2890]
            tunnel: [w2887 w2889] -> w2877
            tunnel: [FALSE TRUE] -> w2875
            frame 0, Default {
            }
            frame -1 {
              n1416 = Build Array (concatenate)(w2890, w2891) -> (w2889:i32[])
            }
          }
          n1417 = case shown="-1" w2882 {
            tunnel: w2879 -> [_ w2895]
            tunnel: w2881 -> [w2892 w2894]
            tunnel: [w2892 w2893] -> w2880
            frame 0, Default {
            }
            frame -1 {
              n1418 = Build Array (concatenate)(w2894, w2895) -> (w2893:i32[])
            }
          }
        }
        n1419 = global write "RFP_Table_Global.vi" "RFP Table"(w2849) -> ()
        n1420 = local read "Result files to read"() -> (w2856:path[])
        n1421 = for {
          tunnel: w2857 -> [w2873] mode=indexing
          tunnel: w2856 -> [w2872]
          tunnel: [w2869] -> w2854 mode=indexing
          n1422 = Index Array(array=w2872, index=w2873) -> (element=w2871:path)
          n1423 = Strip Path(path=w2871) -> (name=w2870:string)  [unwired: 1 out]
          n1424 = call "Add_filename_suffix.vi"("Filename"=w2870) -> ("Base name"=w2869:string)  [unwired: 1 in, 3 out]
        }
        n1425 = call "Summarise.vi"("Channel Names"=w2851, "Data"=w2865, "Summarise All"=w2864) -> ("Summary"=w2867:string[][])  [unwired: 2 in]
        n1426 = global write "Results_plotter_Global.vi" "Plot Summary"(w2867) -> ()
        n1427 = local read "Intensity Plot?"() -> (w2863:bool)
        n1428 = call "Value_Occurence_Analysis.vi"("String Array"=w2854) -> ("Output String"=w2853:string)  [unwired: 3 in, 2 out]
        n1429 = global write "Results_plotter_Global.vi" "Current Data Filenames"(w2853) -> ()
        n1430 = Select(t="Save Intensity plot as jpg", s=w2863, f="Save XY plot as jpg") -> (s? t:f=w2855:string)
      }
      frame "Save Intensity plot as jpg" {
        n1431 = global read "Constants_global.vi" "EnFlo SW Folder"() -> (w2905:path)
        n1432 = local read "Job Directory"() -> (w2903:path)
        n1433 = Build Path(base path=w2905, name or relative path=path "Anemometry/Anemometry Sub Vis/Data_plotting_vis/Intensity Plot Vis") -> (appended path=w2899:path)
        n1434 = call "Remote_call_prep.vi"("Vi Name in"="Create picture Vi Name", "Job Directory In"=w2903, "VI Directory"=w2899) -> ("Vi Name out"=w2901:string, "Job Directory out"=w2898:path, "cancelled"=w2897:bool)
        n1435 = local write "Create picture Vi Name"(w2901) -> ()
        n1436 = local write "Job Directory"(w2898) -> ()
        n1437 = Build Path(base path=w2899, name or relative path=w2901) -> (appended path=w2900:path)
        n1438 = case shown="False" w2897 {
          tunnel: w2900 -> [w2913 _]
          tunnel: w2898 -> [w2912 _]
          frame False {
            n1439 = Open VI Reference(type specifier VI Refnum (for type only)="type specifier", vi path=w2913) -> (vi reference=w2918:refnum<vi>, error out=w2917:errorcluster)  [unwired: 2 in, 2 out]
            n1440 = property class="VI Interface Type 8"(reference=w2918, error in=w2917, "Front Panel Window:Open"=TRUE) -> (reference out=w2914:refnum<vi>, error out=w2915:errorcluster)
            n1441 = local read "Intensity Graph"() -> (w2921:dbl[][])
            n1442 = local read "No of Contours"() -> (w2911:i32)
            n1443 = call-by-ref "?"(reference=w2914, error in=w2915, "No of Contours"=w2911, "Job Directory"=w2912, "Intensity Graph"=w2921) -> (reference out=w2920:refnum<vi>, error out=w2919:errorcluster)  [unwired: 3 in]
            n1444 = Close Reference(reference=w2920, error in (no error)=w2919) -> ()  [unwired: 1 out]
          }
          frame True {
          }
        }
        n1445 = local write "passToPictureVI"(FALSE ("Save All data")) -> ()
      }
      frame "Run Calculation Routine" {
        n1446 = stacked-sequence {
          seq-local: [w2931 _ _] -> [_ w2938 _]
          seq-local: [w2930 _ _] -> [_ w2939 _]
          tunnel: [_ w2937 _] -> w2925
          tunnel: w2923 -> [w2929 _ _]
          frame #0 {
            n1447 = local read "Job Directory"() -> (w2933:path)
            n1448 = call "Remote_call_prep.vi"("Vi Name in"="...using routine", "Job Directory In"=w2933, "VI Directory"=w2929) -> ("Vi Name out"=w2934:string, "Job Directory out"=w2932:path, "cancelled"=w2931:bool)
            n1449 = local write "...using routine"(w2934) -> ()
            n1450 = local write "Job Directory"(w2932) -> ()
            n1451 = Build Path(base path=w2929, name or relative path=w2934) -> (appended path=w2930:path)
          }
          frame #1 {
            n1452 = case shown="False" w2938 {
              tunnel: w2939 -> [w2947 _]
              tunnel: [w2943 w2960] -> w2937
              tunnel: "What to do next?" -> [w2942 w2960]
              frame False {
                n1453 = Open VI Reference(type specifier VI Refnum (for type only)="VI Refnum Calculation", vi path=w2947) -> (vi reference=w2953:refnum<vi>, error out=w2952:errorcluster)  [unwired: 1 in, 3 out]
                n1454 = property class="VI Interface Type 9"(reference=w2953, error in=w2952, "Front Panel Window:Open"=TRUE) -> (reference out=w2949:refnum<vi>, error out=w2950:errorcluster)
                n1455 = call-by-ref "?"(reference=w2949, error in=w2950) -> (reference out=w2955:refnum<vi>, error out=w2954:errorcluster, "New Values In"=w2940:string[][], "New Chs In"=w2948:string[])  [unwired: 2 in]
                n1456 = global write "Results_plotter_Global.vi" "New Values In"(w2940) -> ()
                n1457 = for {
                  tunnel: w2948 -> [w2958] mode=indexing
                  tunnel: [w2957] -> w2941 mode=indexing
                  n1458 = call "Check_Ch_Name_colons.vi"("No of Colons"=2, "Ch Name in"=w2958) -> ("Ch Name out"=w2957:string)
                }
                n1459 = Empty String/Path?(string/path=w2941) -> (empty?=w2945:bool[])
                n1460 = Close Reference(reference=w2955, error in (no error)=w2954) -> ()  [unwired: 1 out]
                n1461 = Or Array Elements(Boolean array=w2945) -> (logical OR=w2944:bool)
                n1462 = global write "Results_plotter_Global.vi" "New Chs In"(w2941) -> ()
                n1463 = Select(t=w2942, s=w2944, f="Input calculated values") -> (s? t:f=w2943:string)
              }
              frame True {
              }
            }
          }
          frame #2 {
            n1464 = local write "Edit Raw Data Header Info"(FALSE ("Raw DF in Orig Pos?")) -> ()
            n1465 = local write "Calculate new metadata"(FALSE ("Save All data")) -> ()
            n1466 = local write "Plotted rows only?"(TRUE ("Plotted rows only?")) -> ()
            n1467 = local write "Mode"(Plotter_Mode."Edit values per row" ("Mode")) -> ()
          }
        }
      }
      frame "Input calculated values" {
        n1468 = local read "Result files to read"() -> (w2969:path[])
        n1469 = stacked-sequence {
          seq-local: [w2976 _ _ _] -> [_ w2989 w2999 _]
          seq-local: [_ w2986 _ _] -> [_ _ w3000 _]
          tunnel: [_ _ _ w3047] -> w2971
          tunnel: w2969 -> [_ _ w3001 _]
          tunnel: "Raw DF in Orig Pos?" -> [_ _ w2998 _]
          tunnel: w2967 -> [_ _ _ w3055]
          frame #0 {
            n1470 = global read "Results_plotter_Global.vi" "New Values Row index"() -> (w2973:i32[])
            n1471 = Array Size(array=w2973) -> (size(s)=w2975:i32)
            n1472 = Greater Than 0?(x=w2975) -> (x > 0?=w2974:bool)
            n1473 = case shown="False" w2974 {
              tunnel: [w2980 w2981] -> w2977
              tunnel: w2973 -> [_ w2981]
              frame False {
                n1474 = global read "Results_plotter_Global.vi" "Plotted Row Numbers"() -> (w2980:i32[])
              }
              frame True {
              }
            }
            n1475 = local write "Delete Plotted data from file"(FALSE ("Save All data")) -> ()
            n1476 = global read "Results_plotter_Global.vi" "Row Reference"() -> (w2978:i32[][])
            n1477 = for {
              tunnel: w2978 -> [w2984]
              tunnel: w2977 -> [w2983] mode=indexing
              tunnel: [w2982] -> w2976 mode=indexing
              n1478 = Index Array(array=w2984, index (row)=w2983) -> (element=w2982:i32[])  [unwired: 1 in]
            }
          }
          frame #1 {
            n1479 = Index Array(array=w2989, index (col)=0 ("disabled index (col)")) -> (element=w2985:i32[])  [unwired: 1 in]
            n1480 = for {
              shift-right: [w2991] -> w2986
              shift-left: i32[] [] -> [w2992]
              tunnel: w2985 -> [w2990] mode=indexing
              n1481 = Search 1D Array(1D array=w2992, element=w2990) -> (index of element=w2993:i32)  [unwired: 1 out]
              n1482 = case shown="-1" w2993 {
                tunnel: w2992 -> [w2994 w2997]
                tunnel: [w2994 w2996] -> w2991
                tunnel: w2990 -> [_ w2995]
                frame 0, Default {
                }
                frame -1 {
                  n1483 = Build Array (concatenate)(w2997, w2995) -> (w2996:i32[])
                }
              }
            }
          }
          frame #2 {
            n1484 = for {
              tunnel: w3001 -> [w3006]
              tunnel: w3000 -> [w3003] mode=indexing
              tunnel: w2999 -> [w3004]
              tunnel: w2998 -> [w3002]
              # "Row in file"
              n1485 = Index Array(array=w3006, index=w3003) -> (element=w3005:path)
              n1486 = stacked-sequence {
                seq-local: [w3011 _] -> [_ w3045]
                seq-local: [w3009 _] -> [_ w3041]
                tunnel: w3005 -> [_ w3046]
                tunnel: w3004 -> [w3013 _]
                tunnel: w3003 -> [w3012 _]
                tunnel: w3002 -> [_ w3044]
                frame #0 {
                  n1487 = global read "Results_plotter_Global.vi" "New Values In"() -> (w3007:string[][])
                  n1488 = for {
                    tunnel: w3012 -> [w3024]
                    tunnel: w3013 -> [w3020] mode=indexing
                    shift-right: [w3018] -> w3011
                    shift-left: i32[] [] -> [w3019]
                    shift-right: [w3017] -> w3009
                    shift-left: string[][] [] -> [w3016]
                    tunnel: w3007 -> [w3015]
                    i -> [w3014]
                    n1489 = Index Array(array=w3020, index=0) -> (element=w3022:i32)
                    n1490 = Equal?(x=w3022, y=w3024) -> (x = y?=w3021:bool)
                    n1491 = case shown="True" w3021 {
                      tunnel: w3020 -> [_ w3030]
                      tunnel: w3019 -> [w3026 w3035]
                      tunnel: [w3026 w3033] -> w3018
                      tunnel: w3016 -> [w3025 w3031]
                      tunnel: [w3025 w3032] -> w3017
                      tunnel: w3015 -> [_ w3028]
                      tunnel: w3014 -> [_ w3027]
                      frame False {
                      }
                      frame True {
                        n1492 = Index Array(array=w3028, index (row)=w3027) -> (element=w3029:string[])  [unwired: 1 in]
                        n1493 = Build Array (concatenate)(w3031, w3029) -> (w3032:string[][])
                        n1494 = Index Array(array=w3030, index=1) -> (element=w3034:i32)
                        n1495 = Build Array (concatenate)(w3035, w3034) -> (w3033:i32[])
                      }
                    }
                  }
                }
                frame #1 {
                  w3040 = FALSE  # Edit all Rows?
                  w3042 = FALSE  # Edit Raw Data Header Info
                  w3043 = FALSE  # Value  Constant?
                  n1496 = local read "Edit Raw Data Files?"() -> (w3037:bool)
                  n1497 = local read "Job Directory"() -> (w3039:path)
                  n1498 = global read "Results_plotter_Global.vi" "New Chs In"() -> (w3038:string[])
                  n1499 = call "Add_Update_Values.vi"("Filename"=w3046, "Value  Constant?"=w3043, "Edit Raw data files?"=w3037, "New Chs In"=w3038, "Edit Raw Data Header Info"=w3042, "New Values In"=w3041, "Selected Rows"=w3045, "Edit all Rows?"=w3040, "Raw DF in Orig Pos?"=w3044, "Job Directory"=w3039) -> ()  [unwired: 1 in, 5 out]
                }
              }
            }
          }
          frame #3 {
            n1500 = global write "Results_plotter_Global.vi" "New Values Row index"(i32[] [] ("New Values Row index")) -> ()
            n1501 = Current VI's Path() -> (path=w3056:path)
            n1502 = global write "Results_plotter_Global.vi" "New Chs In"(string[] [] ("New Chs In")) -> ()
            n1503 = global write "Results_plotter_Global.vi" "New Values In"(string[][] [] ("New Values In")) -> ()
            n1504 = call "Bring_to_front.vi"("path"=w3056) -> ()
            n1505 = local read "nRows"() -> (w3051:i32)
            n1506 = Less?(x=w3051, y=w3055) -> (x < y?=w3050:bool)
            n1507 = Select(t="Initialise", s=w3050, f="Create Selectors") -> (s? t:f=w3047:string)
          }
        }
      }
      frame "Save XY plot as jpg" {
        n1508 = local read "Create picture Vi Name"() -> (w3064:string)
        n1509 = local read "Job Directory"() -> (w3066:path)
        n1510 = call "Remote_call_prep.vi"("Vi Name in"=w3064, "Job Directory In"=w3066, "VI Directory"=w3058) -> ("Vi Name out"=w3065:string, "Job Directory out"=w3062:path, "cancelled"=w3061:bool)
        n1511 = Build Path(base path=w3058, name or relative path=w3065) -> (appended path=w3063:path)
        n1512 = local write "Create picture Vi Name"(w3065) -> ()
        n1513 = case shown="False" w3061 {
          tunnel: [w3098 FALSE ("Saved Automatically?")] -> w3069
          tunnel: [w3097 path "" ("Plot data file")] -> w3068
          tunnel: [w3096 "" ("Tex Info String")] -> w3067
          tunnel: w3063 -> [w3094 _]
          tunnel: w3062 -> [w3095 _]
          tunnel: [w3093 errorcluster {"status"=TRUE, "code"=0, "source"=""} ("error out")] -> w3057
          frame False {
            n1514 = Open VI Reference(type specifier VI Refnum (for type only)="type specifier2", vi path=w3094) -> (vi reference=w3104:refnum<vi>, error out=w3103:errorcluster)  [unwired: 1 in, 3 out]
            n1515 = property class="VI Interface Type 10"(reference=w3104, error in=w3103, "Front Panel Window:Open"=TRUE) -> (reference out=w3100:refnum<vi>, error out=w3101:errorcluster)
            n1516 = call-by-ref "?"(reference=w3100, error in=w3101, "Job Directory"=w3095) -> (reference out=w3106:refnum<vi>, error out=w3105:errorcluster, "Saved Automatically?"=w3098:bool, "gnuplotScript"=w3096:string, "Plot data file"=w3097:path)  [unwired: 1 in]
            n1517 = Close Reference(reference=w3106, error in (no error)=w3105) -> (error out=w3093:errorcluster)
          }
          frame True {
          }
        }
        n1518 = disable-structure shown="Disabled" {
          disable-tunnel: w3057 -> [w3076 _]
          frame Disabled {
            n1519 = call "Stall Data Flow.vim"("value in"=w3076, "milliseconds to wait"=u32 600) -> ("value out"=w3074:errorcluster)  [unwired: 1 out]
            n1520 = case shown="No Error" w3074 {
              frame No Error {
                n1521 = while {
                  stop <- w3080 stop-if-true
                  n1522 = control-ref of="This VI"() -> (w3081:refnum<vi>)
                  n1523 = Wait (ms)(milliseconds to wait=u32 50) -> ()  [unwired: 1 out]
                  n1524 = call <vilib>:"Set Busy.vi"() -> ()  [unwired: 10 in, 2 out]
                  n1525 = property class="VI"(reference=w3081) -> ("Front Panel.IsFrontmost"=w3080:bool)  [unwired: 1 in, 2 out]
                  n1526 = property on="Create picture Vi Name" class="CmbBox"() -> ("Strings[]"=w3079:string[])  [unwired: 2 in, 2 out]
                  n1527 = case shown="True" w3080 {
                    tunnel: w3079 -> [_ w3084]
                    tunnel: "Stop Button" ("Control Name") -> [_ w3082]
                    frame False {
                    }
                    frame True {
                      n1528 = for {
                        tunnel: w3084 -> [w3091] mode=indexing
                        tunnel: [w3088] -> w3083 mode=indexing
                        tunnel: w3082 -> [w3086]
                        stop <- w3085 continue-if-true
                        n1529 = Open VI Reference(vi path=w3091) -> (vi reference=w3092:refnum<vi>, error out=w3089:errorcluster)  [unwired: 5 in]
                        n1530 = invoke class="VI" method="Ctrl Val.Set"(reference=w3092, error in=w3089, "Control Name"=w3086, "Value"=TRUE) -> (reference out=w3090:refnum<vi>, error out=w3085:errorcluster)  [unwired: 1 in, 3 out]
                        n1531 = Close Reference(reference=w3090, error in (no error)=w3085) -> (error out=w3088:errorcluster)
                      }
                      "Array" <- w3083
                    }
                  }
                }
              }
              frame Error {
              }
            }
          }
          frame Enabled {
          }
        }
        n1532 = local write "Job Directory"(w3062) -> ()
        n1533 = case shown="False" w3069 {
          tunnel: w3068 -> [_ w3119]
          tunnel: [w3111 "Save Plot Data"] -> w3060
          tunnel: w3067 -> [_ w3117]
          frame False {
            n1534 = global read "Results_plotter_Global.vi" "New Chs In"() -> (w3116:string[])
            n1535 = Array Size(array=w3116) -> (size(s)=w3115:i32)
            n1536 = Greater Than 0?(x=w3115) -> (x > 0?=w3114:bool)
            n1537 = Select(t="Input calculated values", s=w3114, f="Create Selectors") -> (s? t:f=w3111:string)
          }
          frame True {
            n1538 = local write "Output Filename"(w3119) -> ()
            n1539 = local write "Header"(w3117) -> ()
          }
        }
        n1540 = local write "passToPictureVI"(FALSE ("Save All data")) -> ()
      }
      frame "Full Res file manipulator" {
        n1541 = local read "Result files to read"() -> (w3135:path[])
        n1542 = local read "Output Filename"() -> (w3133:path)
        n1543 = local read "Full_Res_Results_Folder"() -> (w3127:path)
        n1544 = local read "Mode"() -> (w3134:T10)
        n1545 = global read "Results_plotter_Global.vi" "New Values In"() -> (w3130:string[][])
        n1546 = global read "Results_plotter_Global.vi" "New Chs In"() -> (w3131:string[])
        n1547 = local read "Raw DF in Orig Pos?"() -> (w3128:bool)
        n1548 = local read "Plotted rows only?"() -> (w3129:bool)
        n1549 = stacked-sequence {
          seq-local: [w3139 _ _ _ _] -> [_ w3168 w3223 _ _]
          seq-local: [_ w3167 _ _ _] -> [_ _ w3209 _ _]
          seq-local: [_ w3163 _ _ _] -> [_ _ w3217 _ _]
          seq-local: [_ _ w3215 _ _] -> [_ _ _ w3464 _]
          seq-local: [_ _ w3214 _ _] -> [_ _ _ w3463 _]
          seq-local: [_ _ w3210 _ _] -> [_ _ _ w3462 _]
          tunnel: [_ _ _ w3467 _] -> w3137
          tunnel: w3135 -> [_ _ w3224 _ _]
          tunnel: w3134 -> [_ w3165 w3222 w3465 _]
          tunnel: w3133 -> [_ _ w3221 _ _]
          tunnel: w3129 -> [w3138 _ w3220 _ _]
          tunnel: w3131 -> [_ _ w3219 _ _]
          tunnel: w3128 -> [_ _ w3218 _ _]
          tunnel: w3132 -> [_ _ _ w3466 _]
          tunnel: w3130 -> [_ _ w3212 _ _]
          tunnel: w3127 -> [_ _ w3207 _ _]
          tunnel: [_ _ w3206 _ _] -> w3125
          tunnel: w3126 -> [_ _ w3206 _ _]
          tunnel: [_ _ w3205 _ _] -> w3124
          tunnel: w3123 -> [_ _ w3205 w3461 _]
          tunnel: [_ _ w3204 _ _] -> w3122
          tunnel: w3121 -> [_ _ w3204 w3460 _]
          frame #0 {
            n1550 = call <vilib>:"Set Busy.vi"() -> ()  [unwired: 10 in, 2 out]
            n1551 = global read "Results_plotter_Global.vi" "Row Reference"() -> (w3140:i32[][])
            n1552 = case shown="True" w3138 {
              tunnel: w3140 -> [w3142 w3143]
              tunnel: [w3142 w3144] -> w3139
              frame False {
              }
              frame True {
                n1553 = local read "Plotted Series"() -> (w3146:bool[][])
                n1554 = for {
                  tunnel: w3146 -> [w3153]
                  shift-right: [w3147] -> w3144
                  shift-left: i32[][] [] -> [w3149]
                  tunnel: w3143 -> [w3148] mode=indexing
                  i -> [w3152]
                  n1555 = Index Array(array=w3153, index (col)=w3152) -> (element=w3151:bool[])  [unwired: 1 in]
                  n1556 = Or Array Elements(Boolean array=w3151) -> (logical OR=w3150:bool)
                  n1557 = case shown="True" w3150 {
                    tunnel: w3149 -> [w3154 w3157]
                    tunnel: w3148 -> [_ w3156]
                    tunnel: [w3154 w3155] -> w3147
                    frame False {
                    }
                    frame True {
                      n1558 = Build Array (concatenate)(w3157, w3156) -> (w3155:i32[][])
                    }
                  }
                }
              }
            }
            n1559 = local write "Delete Plotted data from file"(FALSE ("Save All data")) -> ()
          }
          frame #1 {
            n1560 = local read "Job Directory"() -> (w3164:path)
            n1561 = case shown="\"Post Process Plotted Rows\"" w3165 {
              tunnel: [FALSE FALSE FALSE w3186 w3189 w3192 w3195 w3198] -> w3166
              tunnel: [w3178 w3180 w3182 w3184 w3187 w3190 w3193 w3196] -> w3163
              tunnel: w3164 -> [w3178 w3180 w3182 w3185 w3188 w3191 w3194 w3197]
              tunnel: [w3178 w3180 w3182 w3184 w3187 w3190 w3193 w3196] -> w3162
              frame "Post Process Plotted Rows" {
                n1562 = global write "Plug_in_data_global.vi" "Plug_in Results Folder"(path "") -> ()
              }
              frame "Save file" {
              }
              frame "Plot EnFlo Tunnel Display" {
              }
              frame "Delete unwanted rows" {
                n1563 = call "Remote_call_prep.vi"("Job Directory In"=w3185) -> ("Job Directory out"=w3184:path)  [unwired: 2 in, 2 out]
                n1564 = local write "Job Directory"(w3184) -> ()
                n1565 = Not Equal?(x=w3185, y=w3184) -> (x != y?=w3186:bool)
              }
              frame "Add Inlet Temperature Offset" {
                n1566 = call "Remote_call_prep.vi"("Job Directory In"=w3188) -> ("Job Directory out"=w3187:path)  [unwired: 2 in, 2 out]
                n1567 = local write "Job Directory"(w3187) -> ()
                n1568 = Not Equal?(x=w3188, y=w3187) -> (x != y?=w3189:bool)
              }
              frame "Edit Values with constants" {
                n1569 = call "Remote_call_prep.vi"("Job Directory In"=w3191) -> ("Job Directory out"=w3190:path)  [unwired: 2 in, 2 out]
                n1570 = local write "Job Directory"(w3190) -> ()
                n1571 = Not Equal?(x=w3191, y=w3190) -> (x != y?=w3192:bool)
              }
              frame "Edit values per row" {
                n1572 = call "Remote_call_prep.vi"("Job Directory In"=w3194) -> ("Job Directory out"=w3193:path)  [unwired: 2 in, 2 out]
                n1573 = local write "Job Directory"(w3193) -> ()
                n1574 = Not Equal?(x=w3194, y=w3193) -> (x != y?=w3195:bool)
              }
              frame "Edit Raw Data file header" {
                n1575 = call "Remote_call_prep.vi"("Job Directory In"=w3197) -> ("Job Directory out"=w3196:path)  [unwired: 2 in, 2 out]
                n1576 = local write "Job Directory"(w3196) -> ()
                n1577 = Not Equal?(x=w3197, y=w3196) -> (x != y?=w3198:bool)
              }
            }
            n1578 = Index Array(array=w3168, index (col)=0 ("disabled index (col)")) -> (element=w3160:i32[])  [unwired: 1 in]
            n1579 = for {
              shift-right: [w3170] -> w3167
              shift-left: i32[] [] -> [w3171]
              tunnel: w3160 -> [w3169] mode=indexing
              n1580 = Search 1D Array(1D array=w3171, element=w3169) -> (index of element=w3172:i32)  [unwired: 1 out]
              n1581 = case shown="-1" w3172 {
                tunnel: w3171 -> [w3173 w3176]
                tunnel: [w3173 w3175] -> w3170
                tunnel: w3169 -> [_ w3174]
                frame 0, Default {
                }
                frame -1 {
                  n1582 = Build Array (concatenate)(w3176, w3174) -> (w3175:i32[])
                }
              }
            }
            n1583 = local read "Template"() -> (w3158:path)
            n1584 = case shown="True" w3166 {
              tunnel: w3162 -> [_ w3200]
              tunnel: w3158 -> [_ w3199]
              frame False {
              }
              frame True {
                n1585 = Path To String(path=w3200) -> (string=w3203:string)
                n1586 = call "Read_Write_Template.vi"("Template File"=w3199, "Mode"=Global_mode."Write Global to File", "Single Value In"=w3203, "Data type"="Log Folder Name" ("Variable name")) -> ()  [unwired: 4 in, 8 out]
              }
            }
            n1587 = global write "Meas_global.vi" "Template File"(w3158) -> ()
          }
          frame #2 {
            w3213 = path[] []
            n1588 = Array Size(array=w3209) -> (size(s)=w3208:i32)
            n1589 = for {
              tunnel: w3224 -> [w3248]
              tunnel: w3209 -> [w3245] mode=indexing
              tunnel: w3223 -> [w3246]
              tunnel: w3222 -> [w3244]
              tunnel: w3221 -> [w3243]
              tunnel: w3220 -> [w3242]
              tunnel: w3219 -> [w3241]
              tunnel: w3218 -> [w3240]
              tunnel: w3217 -> [w3239]
              shift-right: [w3238] -> _
              shift-left: FALSE -> [w3237]
              shift-right: [w3235] -> w3215
              shift-left: w3213 -> [w3236]
              shift-right: [w3233] -> w3214
              shift-left: w3213 -> [w3234]
              tunnel: w3212 -> [w3232]
              shift-right: [w3230] -> w3210
              shift-left: i32[] [] -> [w3231]
              tunnel: w3208 -> [w3228]
              tunnel: w3207 -> [w3227]
              tunnel: w3205 -> [w3226]
              tunnel: w3204 -> [w3225]
              i -> [w3229]
              # "Row No in file"
              # "Row No in plotter"
              n1590 = Index Array(array=w3248, index=w3245) -> (element=w3247:path)
              n1591 = stacked-sequence {
                seq-local: [w3253 _ _ _] -> [_ w3287 w3343 _]
                seq-local: [_ w3285 _ _] -> [_ _ w3342 _]
                seq-local: [w3249 _ _ _] -> [_ _ w3337 w3458]
                tunnel: w3247 -> [_ w3286 w3344 _]
                tunnel: w3246 -> [w3261 _ _ _]
                tunnel: w3245 -> [w3256 _ _ _]
                tunnel: w3244 -> [_ w3284 w3341 _]
                tunnel: w3243 -> [_ _ w3340 _]
                tunnel: w3242 -> [_ _ w3339 _]
                tunnel: w3241 -> [_ _ w3338 _]
                tunnel: w3240 -> [_ _ w3336 _]
                tunnel: w3239 -> [_ _ w3335 _]
                tunnel: [_ w3283 _ _] -> w3238
                tunnel: w3237 -> [_ w3282 _ _]
                tunnel: w3236 -> [_ _ w3334 _]
                tunnel: [_ _ w3333 _] -> w3235
                tunnel: w3234 -> [_ _ w3332 _]
                tunnel: [_ _ w3331 _] -> w3233
                tunnel: w3227 -> [_ _ w3330 _]
                tunnel: w3232 -> [_ _ w3329 _]
                tunnel: w3231 -> [_ _ _ w3459]
                tunnel: [_ _ _ w3457] -> w3230
                tunnel: w3229 -> [_ _ w3328 _]
                tunnel: w3228 -> [_ _ w3327 _]
                tunnel: w3226 -> [_ _ w3326 _]
                tunnel: w3225 -> [_ _ w3325 _]
                frame #0 {
                  w3260 = i32[] []
                  # "10/30/13\n#optimation"
                  n1592 = for {
                    tunnel: w3256 -> [w3270]
                    tunnel: w3261 -> [w3266] mode=indexing
                    shift-right: [w3264] -> w3254
                    shift-left: w3260 -> [w3265]
                    shift-right: [w3263] -> w3250
                    shift-left: w3260 -> [w3262]
                    n1593 = Index Array(array=w3266, index=0) -> (element=w3268:i32)
                    n1594 = Equal?(x=w3268, y=w3270) -> (x = y?=w3267:bool)
                    n1595 = case shown="True" w3267 {
                      tunnel: w3266 -> [_ w3274]
                      tunnel: w3265 -> [w3272 w3280]
                      tunnel: [w3272 w3278] -> w3264
                      tunnel: w3262 -> [w3271 w3276]
                      tunnel: [w3271 w3277] -> w3263
                      frame False {
                      }
                      frame True {
                        n1596 = Index Array(array=w3274, index=2) -> (element=w3273:i32)
                        n1597 = Build Array (concatenate)(w3276, w3273) -> (w3277:i32[])
                        n1598 = Index Array(array=w3274, index=1) -> (element=w3279:i32)
                        n1599 = Build Array (concatenate)(w3280, w3279) -> (w3278:i32[])
                      }
                    }
                  }
                  n1600 = global read "Results_plotter_Global.vi" "Row Reference"() -> (w3259:i32[][])
                  n1601 = local read "Cursor index"() -> (w3258:i32)
                  n1602 = Index Array(array=w3259, index (row)=w3258) -> (element=w3257:i32[])  [unwired: 1 in]
                  n1603 = Index Array(array=w3257) -> (element #2=w3255:i32)  [unwired: 2 in, 1 out]
                  n1604 = Build Array(w3255) -> (w3252:i32[])
                  n1605 = local read "justCursorPt"() -> (w3251:bool)
                  n1606 = Select(t=w3252, s=w3251, f=w3250) -> (s? t:f=w3249:i32[])
                  n1607 = Select(t=w3252, s=w3251, f=w3254) -> (s? t:f=w3253:i32[])
                }
                frame #1 {
                  n1608 = case shown="\"Post Process Plotted Rows\"" w3284 {
                    tunnel: w3287 -> [_ _ _ _ _ _ _ w3308]
                    tunnel: w3286 -> [_ _ _ _ _ _ _ w3306]
                    tunnel: [TRUE ("T button?") TRUE ("T button?") TRUE ("T button?") TRUE ("T button?") TRUE ("T button?") TRUE ("T button?") TRUE ("T button?") w3305] -> w3285
                    tunnel: [w3288 w3290 w3293 w3295 w3297 w3299 w3301 w3304] -> w3283
                    tunnel: w3282 -> [w3288 w3290 w3293 w3295 w3297 w3299 w3301 w3303]
                    frame "Save file" {
                    }
                    frame "Add Inlet Temperature Offset" {
                    }
                    frame "Plot EnFlo Tunnel Display" {
                      n1609 = local read "Index when last plotted"() -> (→"Index when last displayed":i32)
                    }
                    frame "Edit values per row" {
                    }
                    frame "Edit Values with constants" {
                    }
                    frame "Edit Raw Data file header" {
                    }
                    frame "Post Process Plotted Rows" {
                    }
                    frame "Delete unwanted rows" {
                      n1610 = Array Size(array=w3308) -> (size(s)=w3307:i32)
                      n1611 = case shown="False" w3303 {
                        tunnel: w3307 -> [w3317 _]
                        tunnel: w3306 -> [w3316 _]
                        tunnel: [w3311 w3324] -> w3305
                        tunnel: [w3310 w3324] -> w3304
                        frame False {
                          n1612 = Format Into String(format string="Remove %d rows from \"%s\"", w3317, w3316) -> (resulting string=w3314:string)  [unwired: 2 in, 1 out]
                          n1613 = call <vilib>:"Three Button Dialog.vi"("Allow user to close window? (TRUE)"=TRUE, "Right Button Text (\"Cancel\")"="Yes To All Files" ("Right Button Text (\"Cancel\")"), "message"=w3314) -> ("Which Button?"=w3312:T19)  [unwired: 3 in, 5 out]
                          n1614 = case shown="\"Center Button\"" w3312 {
                            tunnel: [TRUE TRUE w3322 w3323] -> w3311
                            tunnel: [FALSE TRUE w3322 w3323] -> w3310
                            frame "Left Button" {
                            }
                            frame "Right Button" {
                            }
                            frame "Center Button" {
                              w3322 = FALSE
                            }
                            frame "Window Close" {
                              w3323 = FALSE
                            }
                          }
                        }
                        frame True {
                          w3324 = TRUE
                        }
                      }
                    }
                  }
                }
                frame #2 {
                  n1615 = case shown="True" w3342 {
                    tunnel: w3344 -> [_ w3365]
                    tunnel: w3343 -> [_ w3364]
                    tunnel: w3341 -> [_ w3363]
                    tunnel: w3340 -> [_ w3362]
                    tunnel: w3339 -> [_ w3361]
                    tunnel: w3338 -> [_ w3360]
                    tunnel: w3337 -> [_ w3359]
                    tunnel: w3336 -> [_ w3358]
                    tunnel: w3335 -> [_ w3357]
                    tunnel: w3334 -> [w3346 w3356]
                    tunnel: [w3346 w3355] -> w3333
                    tunnel: w3332 -> [w3345 w3354]
                    tunnel: [w3345 w3353] -> w3331
                    tunnel: w3330 -> [_ w3352]
                    tunnel: w3329 -> [_ w3351]
                    tunnel: w3328 -> [_ w3350]
                    tunnel: w3327 -> [_ w3349]
                    tunnel: w3326 -> [_ w3348]
                    tunnel: w3325 -> [_ w3347]
                    frame False {
                    }
                    frame True {
                      n1616 = case shown="\"Edit Raw Data file header\", Default" w3363 {
                        tunnel: w3365 -> [w3371 w3379 w3394 w3401 w3408 w3428 w3445]
                        tunnel: w3364 -> [w3374 _ w3393 w3400 w3409 w3427 w3444]
                        tunnel: w3362 -> [_ _ _ _ _ _ _]
                        tunnel: w3361 -> [_ _ _ _ _ w3425 w3442]
                        tunnel: w3360 -> [_ _ _ _ _ w3423 w3440]
                        tunnel: w3359 -> [_ w3378 _ _ w3410 _ w3438]
                        tunnel: w3358 -> [_ _ _ _ _ w3422 w3436]
                        tunnel: w3357 -> [_ _ _ _ _ w3421 w3435]
                        tunnel: w3356 -> [w3373 w3383 w3392 w3403 w3412 w3419 w3433]
                        tunnel: [w3373 w3384 w3392 w3403 w3412 w3419 w3433] -> w3355
                        tunnel: w3354 -> [w3372 w3382 w3391 w3402 w3411 w3418 w3432]
                        tunnel: [w3372 w3380 w3391 w3402 w3411 w3418 w3432] -> w3353
                        tunnel: w3352 -> [w3370 _ _ _ _ _ _]
                        tunnel: w3351 -> [_ _ _ _ _ w3417 _]
                        tunnel: w3350 -> [_ _ _ w3396 _ _ _]
                        tunnel: w3349 -> [_ _ _ w3398 _ _ _]
                        tunnel: w3348 -> [_ _ _ _ w3405 _ w3430]
                        tunnel: w3347 -> [_ w3375 _ _ w3404 _ w3429]
                        frame "Save file" {
                          n1617 = Strip Path(path=w3371) -> (name=w3368:string)  [unwired: 1 out]
                          n1618 = call "Add_filename_suffix.vi"("Filename"=w3368, "Suffix to add"=".xls") -> ("Filename out"=w3366:string)  [unwired: 3 out]
                          n1619 = Build Path(base path=w3370, name or relative path=w3366) -> (appended path=w3369:path)
                          n1620 = call "Save_full_Res_rows.vi"("Selected Rows"=w3374, "Filename to write"=w3369, "Filename Orig"=w3371) -> ()  [unwired: 2 out]
                        }
                        frame "Edit Raw Data file header", Default {
                          n1621 = global read "Results_plotter_Global.vi" "Raw Data Filename index"() -> (w3377:i32)
                          n1622 = Index Array(array=w3375, index (col)=w3377) -> (element=w3376:string[])  [unwired: 1 in]
                          n1623 = for {
                            tunnel: w3376 -> [w3390]
                            tunnel: w3378 -> [w3386] mode=indexing
                            tunnel: [w3388] -> w3385 mode=indexing
                            tunnel: [w3387] -> w3381 mode=indexing
                            tunnel: w3379 -> [w3387]
                            n1624 = Index Array(array=w3390, index=w3386) -> (element=w3389:string)
                            n1625 = call "String_to_Pathname.vi"("Input String"=w3389) -> ("path"=w3388:path)
                          }
                          n1626 = Build Array (concatenate)(w3382, w3381) -> (w3380:path[])
                          n1627 = Build Array (concatenate)(w3383, w3385) -> (w3384:path[])
                        }
                        frame "Delete unwanted rows" {
                          n1628 = call "Delete_unwanted_rows.vi"("Selected Rows"=w3393, "Filename"=w3394) -> ()  [unwired: 1 out]
                        }
                        frame "Plot EnFlo Tunnel Display" {
                          n1629 = Decrement(x=w3398) -> (x-1=w3397:i32)
                          n1630 = Equal?(x=w3397, y=w3396) -> (x = y?=w3395:bool)
                          n1631 = Equal To 0?(x=w3396) -> (x = 0?=w3399:bool)
                          n1632 = call "Get_requested_rows_from_files.vi"("Last File"=w3395, "First file"=w3399, "Filename"=w3401, "Selected Rows"=w3400) -> ()  [unwired: 3 in]
                        }
                        frame "Add Inlet Temperature Offset" {
                          n1633 = for {
                            tunnel: w3410 -> [w3415] mode=indexing
                            tunnel: [w3414] -> w3407 mode=indexing
                            tunnel: w3404 -> [w3413]
                            n1634 = Index Array(array=w3413, index (row)=w3415) -> (element=w3414:string[])  [unwired: 1 in]
                          }
                          n1635 = local read "Job Directory"() -> (w3406:path)
                          n1636 = call "Get_Inlet_temps_from_files.vi"("Templated Plotted channels"=w3407, "Job Directory"=w3406, "Templated Channel Names"=w3405, "Filename"=w3408, "Selected Rows"=w3409) -> ()  [unwired: 7 in]
                        }
                        frame "Edit Values with constants" {
                          w3426 = TRUE  # Value  Constant?
                          n1637 = local read "Edit Raw Data Header Info"() -> (w3420:bool)
                          n1638 = Not(x=w3425) -> (.not. x?=w3424:bool)
                          n1639 = call "Add_Update_Values.vi"("Filename"=w3428, "Value  Constant?"=w3426, "Edit Raw data files?"="Edit Raw Data Files?", "New Chs In"=w3423, "Edit Raw Data Header Info"=w3420, "New Values In"=w3417, "Selected Rows"=w3427, "Edit all Rows?"=w3424, "Raw DF in Orig Pos?"=w3422, "Job Directory"=w3421) -> ()  [unwired: 1 in, 5 out]
                        }
                        frame "Edit values per row" {
                          n1640 = for {
                            tunnel: w3440 -> [w3456] mode=indexing
                            tunnel: w3430 -> [w3454]
                            tunnel: [w3455] -> w3439 mode=indexing
                            n1641 = Search 1D Array(1D array=w3454, element=w3456) -> (index of element=w3455:i32)  [unwired: 1 out]
                          }
                          n1642 = for {
                            tunnel: w3439 -> [w3450]
                            tunnel: w3438 -> [w3448] mode=indexing
                            tunnel: [w3447] -> w3437 mode=indexing
                            tunnel: w3429 -> [w3446]
                            n1643 = Index Array(array=w3446, index (row)=w3448) -> (element=w3449:string[])  [unwired: 1 in]
                            n1644 = for {
                              tunnel: w3450 -> [w3453] mode=indexing
                              tunnel: w3449 -> [w3452]
                              tunnel: [w3451] -> w3447 mode=indexing
                              n1645 = Index Array(array=w3452, index=w3453) -> (element=w3451:string)
                            }
                          }
                          n1646 = local read "Edit Raw Data Files?"() -> (w3431:bool)
                          n1647 = Not(x=w3442) -> (.not. x?=w3441:bool)
                          n1648 = call "Add_Update_Values.vi"("Filename"=w3445, "Value  Constant?"=FALSE, "Edit Raw data files?"=w3431, "New Chs In"=w3440, "Edit Raw Data Header Info"=FALSE, "New Values In"=w3437, "Selected Rows"=w3444, "Edit all Rows?"=w3441, "Raw DF in Orig Pos?"=w3436, "Job Directory"=w3435) -> ()  [unwired: 1 in, 5 out]
                        }
                      }
                    }
                  }
                }
                frame #3 {
                  n1649 = Build Array (concatenate)(w3459, w3458) -> (w3457:i32[])
                }
              }
            }
          }
          frame #3 {
            n1650 = case shown="\"Post Process Plotted Rows\"" w3465 {
              tunnel: ["Create Selectors" "Create Selectors" w3476 "Initialise" ("t") w3507 w3514 w3520 w3527] -> w3467
              tunnel: w3466 -> [_ _ _ _ w3512 w3513 w3519 w3526]
              tunnel: w3464 -> [w3468 _ w3475 _ _ _ _ _]
              tunnel: w3463 -> [_ _ w3474 _ _ _ _ _]
              tunnel: w3461 -> [_ _ w3473 _ _ _ _ _]
              tunnel: w3462 -> [_ _ w3472 _ _ _ _ _]
              tunnel: w3460 -> [_ _ w3471 _ _ _ _ _]
              frame "Edit Raw Data file header" {
                n1651 = call "Edit_Raw_DF_Header.vi"("Selected files"=w3468) -> ()  [unwired: 15 out]
              }
              frame "Plot EnFlo Tunnel Display" {
              }
              frame "Post Process Plotted Rows" {
                n1652 = stacked-sequence {
                  seq-local: [_ w3480 _] -> [_ _ w3501]
                  tunnel: [_ _ "Create Selectors"] -> w3476
                  tunnel: w3475 -> [_ _ w3504]
                  tunnel: w3474 -> [_ _ w3503]
                  tunnel: w3473 -> [_ _ w3502]
                  tunnel: w3472 -> [_ w3479 _]
                  tunnel: w3471 -> [_ w3478 _]
                  frame #0 {
                    n1653 = local write "Post Process Plotted Data"(FALSE ("Post Process Plotted Data")) -> ()
                  }
                  frame #1 {
                    n1654 = global read "Results_plotter_Global.vi" "Precision"() -> (w3481:string[])
                    n1655 = for {
                      tunnel: w3481 -> [w3486]
                      tunnel: [w3485] -> w3480 mode=indexing
                      tunnel: w3479 -> [w3484] mode=indexing
                      tunnel: w3478 -> [w3482] mode=indexing
                      n1656 = Index Array(array=w3482, index=w3484) -> (element=w3483:string)
                      n1657 = for {
                        tunnel: w3483 -> [w3488]
                        tunnel: w3486 -> [w3487] mode=indexing
                        tunnel: [w3490] -> w3485 mode=indexing
                        n1658 = Fract/Exp String To Number(string=w3488) -> (offset past number=w3494:i32, number=w3491:dbl)  [unwired: 3 out]
                        n1659 = String Length(string=w3488) -> (length=w3495:i32)
                        n1660 = Equal?(x=w3495, y=w3494) -> (x = y?=w3492:bool)
                        n1661 = Empty String/Path?(string/path=w3488) -> (empty?=w3493:bool)
                        n1662 = Compound Arithmetic op=AND(invert w3493, w3492) -> (w3489:bool)
                        n1663 = case shown="True" w3489 {
                          tunnel: w3487 -> [_ w3498]
                          tunnel: w3491 -> [_ w3499]
                          tunnel: [w3496 w3497] -> w3490
                          tunnel: w3488 -> [w3496 _]
                          frame False {
                          }
                          frame True {
                            n1664 = call "Number_2_string.vi"("precision"=w3498, "number"=w3499) -> ("String"=w3497:string)
                          }
                        }
                      }
                    }
                  }
                  frame #2 {
                    n1665 = call "Post_Process_Profile_Remote.vi"("Per Block Plug Ins Extra"="Per Block Plug Ins Extra", "Results Plotter Rows"=w3501, "Results Plotter Channel names"=w3502, "Current Results filenames"=w3503, "Raw Data files to PP"=w3504) -> ()  [unwired: 3 in]
                  }
                }
              }
              frame "Delete unwanted rows" {
              }
              frame "Edit Values with constants" {
                n1666 = local read "nRows"() -> (w3511:i32)
                n1667 = Less?(x=w3511, y=w3512) -> (x < y?=w3508:bool)
                n1668 = Select(t="Initialise", s=w3508, f="Create Selectors") -> (s? t:f=w3507:string)
              }
              frame "Edit values per row" {
                n1669 = local read "nRows"() -> (w3518:i32)
                n1670 = Less?(x=w3518, y=w3513) -> (x < y?=w3515:bool)
                n1671 = Select(t="Initialise", s=w3515, f="Create Selectors") -> (s? t:f=w3514:string)
              }
              frame "Add Inlet Temperature Offset" {
                n1672 = local read "nRows"() -> (w3524:i32)
                n1673 = Less?(x=w3524, y=w3519) -> (x < y?=w3523:bool)
                n1674 = Select(t="Initialise", s=w3523, f="Create Selectors") -> (s? t:f=w3520:string)
                n1675 = local write "Add Inlet Temperature offset"(FALSE ("Add Inlet Temperature offset")) -> ()
              }
              frame "Save file" {
                n1676 = local read "nRows"() -> (w3531:i32)
                n1677 = Less?(x=w3531, y=w3526) -> (x < y?=w3530:bool)
                n1678 = Select(t="Initialise", s=w3530, f="Create Selectors") -> (s? t:f=w3527:string)
              }
            }
          }
          frame #4 {
            n1679 = call <vilib>:"Unset Busy.vi"() -> ()  [unwired: 11 in, 1 out]
            n1680 = Current VI's Path() -> (path=w3535:path)
            n1681 = call "Bring_to_front.vi"("path"=w3535) -> ()
            n1682 = global write "Results_plotter_Global.vi" "New Values In"(string[][] [] ("New Values In")) -> ()
            n1683 = global write "Results_plotter_Global.vi" "New Chs In"(string[] [] ("New Chs In")) -> ()
            n1684 = local write "justCursorPt"(FALSE ("justCursorPt")) -> ()
          }
        }
        n1685 = local write "Kill Point"(FALSE ("Kill Point")) -> ()
      }
      frame "Empty Results file array" {
        n1686 = local write "flushFiles"(FALSE ("Empty")) -> ()
        n1687 = local read "Template"() -> (w3538:path)
        n1688 = call "Valid_Path.vi"("Filename"=w3538) -> ("Valid Path?"=w3537:bool)
        n1689 = local write "Result files to read"(path[] [] ("Result files to read")) -> ()
        n1690 = property on="Result files to read" class="Arr (strict)"("Index Values"=u32[] [0] ("Write Attribute")) -> ()  [unwired: 2 in, 2 out]
        n1691 = case shown="False" w3537 {
          tunnel: w3539 -> [w3547 _]
          frame False {
            n1692 = local write "Template"(w3547) -> ()
            n1693 = global write "Results_plotter_Global.vi" "Template"(w3547) -> ()
          }
          frame True {
          }
        }
      }
      frame "Save Setup" {
        n1694 = stacked-sequence {
          seq-local: [w3568 _] -> [_ w3597]
          tunnel: [w3562 _] -> w3557
          tunnel: w3556 -> [w3562 _]
          tunnel: [w3561 _] -> w3555
          tunnel: w3554 -> [w3561 _]
          tunnel: [_ w3595] -> w3553
          tunnel: w3552 -> [_ w3599]
          tunnel: [_ TRUE ("OK?")] -> w3551
          tunnel: [w3560 _] -> w3550
          tunnel: w3549 -> [w3560 _]
          tunnel: w3548 -> [w3559 _]
          frame #0 {
            n1695 = local read "Multi Ordinate"() -> (w3566:i32[])
            n1696 = local read "Filter Array"() -> (w3571:u16[])
            n1697 = Build Array (concatenate)(w3559, w3562) -> (w3569:string[])
            n1698 = local read "Create picture Vi Name"() -> (w3574:string)
            n1699 = local read "Absisca"() -> (w3565:u16)
            n1700 = for {
              tunnel: w3562 -> [w3583]
              tunnel: w3566 -> [w3582] mode=indexing
              tunnel: [w3581] -> w3567 mode=indexing
              n1701 = Index Array(array=w3583, index=w3582) -> (element=w3581:string)
            }
            n1702 = local read "Additional X Values"() -> (w3577:dbl[])
            n1703 = local read "Additional Y Values"() -> (w3576:dbl[])
            n1704 = local read "Result files to read"() -> (w3579:path[])
            n1705 = local read "Output Filename"() -> (w3575:path)
            n1706 = local read "Intensity Plot?"() -> (w3573:bool)
            n1707 = for {
              N: 6 -> [_]
              tunnel: w3569 -> [w3586]
              tunnel: w3571 -> [w3585] mode=indexing
              tunnel: [w3584] -> w3570 mode=indexing
              n1708 = Index Array(array=w3586, index=w3585) -> (element=w3584:string)
            }
            n1709 = local read "Transpose"() -> (w3578:bool)
            n1710 = local read "Template"() -> (w3572:path)
            n1711 = Index Array(array=w3562, index=w3565) -> (element=w3564:string)
            n1712 = local read "nRows"() -> (w3563:i32)
            n1713 = Bundle By Name(cluster=T17 {"Result files to read"=[], "Template"=path "", "Transpose"=FALSE, "Additional X Values"=[], "Additional Y Values"=[], "Output Filename"=path "", "Create Picture Vi Name"="Intensity plot jpg.vi", "Intensity Plot?"=FALSE, "Multi Ordinate"=[], "Abscissa String"="", "Filter Array"=["", "", "", "", "", ""], "Filter Bins 1 Strings"=[""], "Filter Bins 2 Strings"=[""], "Filters 3 onwards"=[], "nRows"=0} ("Cluster"), "nRows"=w3563, "Result files to read"=w3579, "Template"=w3572, "Transpose"=w3578, "Additional X Values"=w3577, "Additional Y Values"=w3576, "Abscissa String"=w3564, "Filter Array"=w3570, "Output Filename"=w3575, "Create Picture Vi Name"=w3574, "Intensity Plot?"=w3573, "Multi Ordinate"=w3567) -> (w3568:T17)
          }
          frame #1 {
            n1714 = local read "Time to Save Setup?"() -> (w3594:bool)
            n1715 = case shown="True" w3594 {
              tunnel: [TRUE w3610] -> w3604
              frame False {
              }
              frame True {
                # "Are we running a multirun?"
                n1716 = global read "Trav_pos_global.vi" "Estimated Completion time"() -> (w3611:string)
                n1717 = local write "Time to Save Setup?"(FALSE ("Time to Save Setup?")) -> ()
                n1718 = Empty String/Path?(string/path=w3611) -> (empty?=w3610:bool)
              }
            }
            n1719 = Bundle By Name(cluster=w3597, "Filter Bins 1 Strings"="Filter Bins 1 Strings", "Filter Bins 2 Strings"="Filter Bins 2 Strings", "Filters 3 onwards"="Filters 3 onwards") -> (w3596:T17)
            n1720 = local read "Template Changed?"() -> (w3593:bool)
            n1721 = local read "stop"() -> (w3606:bool)
            n1722 = call "Read_Write_Plot_Setup.vi"("Mode"=enum16{"Load", "Save"}."Save", "Setup filename"=w3599, "Cluster"=w3596) -> ()  [unwired: 6 in, 3 out]
            n1723 = Select(t="Initialise", s=w3593, f="Check modification dates?") -> (s? t:f=w3591:string)
            n1724 = Compound Arithmetic op=OR(w3606, invert w3604) -> (w3605:bool)
            n1725 = local read "Save Setup"() -> (w3607:bool)
            n1726 = Select(t="End", s=w3605, f=w3591) -> (s? t:f=w3603:string)
            n1727 = Select(t="Save to named setup file", s=w3607, f=w3603) -> (s? t:f=w3595:string)
          }
        }
      }
      frame "Save to named setup file" {
        n1728 = flat-sequence {
          tunnel: [w3618] -> w3612
          tunnel: w3612 -> [w3622]
          frame #0 {
            w3621 = TRUE  # Save New File?
            n1729 = local read "Job Directory"() -> (w3619:path)
            n1730 = call "Save_current_setup.vi"("Save New File?"=w3621, "jobDirectory"=w3619, "Setup File Type"=Setup_Filetype."Results File Plotter Setups") -> ("Saved filepath"=w3618:path)  [unwired: 2 out]
          }
          frame #1 {
            n1731 = local write "setupOrINI"(w3622) -> ()
            n1732 = local write "Save Setup"(FALSE ("Save Setup")) -> ()
          }
        }
      }
      frame "importSetup" {
        w3625 = TRUE ("importingSetup")
        n1733 = local read "Job Directory"() -> (w3631:path)
        n1734 = control-ref of="This VI"() -> (w3630:refnum<vi>)
        n1735 = call "INI-FP.vi"("Mode"=enum16{"Read", "Write"}."Read", "prompt"="Choose setup to load", "VIreference"=w3630, "INIfilepathIn"=w3631) -> ("INIfilepathOut"=→"setupOrINI":path)  [unwired: 6 in, 1 out]
        n1736 = local write "loadingSetup"(w3625) -> ()
        n1737 = local write "importSetup"(FALSE ("importSetup")) -> ()
        "importingSetup" <- w3625
      }
      frame "exportSetup" {
        n1738 = flat-sequence {
          tunnel: [w3644] -> w3636
          frame #0 {
            # "Dont save setup with the button pressed in!\nAnd put the tab on a useful page- else it'll always be Setups!"
            n1739 = local write "exportSetup"(FALSE ("exportSetup")) -> ()
            n1740 = local write "Tab Control"(T1."Load " ("Tab Control")) -> ()
          }
          frame #1 {
            n1741 = local read "Job Directory"() -> (w3648:path)
            n1742 = control-ref of="This VI"() -> (w3647:refnum<vi>)
            n1743 = call "INI-FP.vi"("Mode"=enum16{"Read", "Write"}."Write", "prompt"="Saving RFP setup", "VIreference"=w3647, "INIfilepathIn"=w3648) -> ("INIfilepathOut"=w3644:path)  [unwired: 6 in, 1 out]
          }
        }
        n1744 = local write "setupOrINI"(w3636) -> ()
      }
      frame "End" {
        w3649 = TRUE ("stop")
        # "to make the event case see it"
        n1745 = local read "flushFiles"() -> (w3656:bool)
        n1746 = local read "Template"() -> (w3655:path)
        n1747 = case shown="True" w3656 {
          frame False {
          }
          frame True {
            n1748 = property on="Result files to read" class="Arr (strict)"("Index Values"=u32[] [0] ("Write Attribute")) -> ()  [unwired: 2 in, 2 out]
            n1749 = local write "Result files to read"(path[] [] ("Result files to read")) -> ()
            n1750 = local write "flushFiles"(FALSE ("Empty")) -> ()
          }
        }
        n1751 = local read "closePressed"() -> (w3650:bool)
        n1752 = call "Valid_Path.vi"("Filename"=w3655) -> ("Valid Path?"=w3654:bool)
        n1753 = case shown="False" w3654 {
          tunnel: w3657 -> [w3666 _]
          frame False {
            n1754 = local write "Template"(w3666) -> ()
            n1755 = global write "Results_plotter_Global.vi" "Template"(w3666) -> ()
          }
          frame True {
          }
        }
        n1756 = case shown="True" w3650 {
          frame False {
          }
          frame True {
            n1757 = control-ref of="This VI"() -> (w3662:refnum<vi>)
            n1758 = invoke class="VI" method="FP.Close"(reference=w3662) -> (error out=w3661:errorcluster)  [unwired: 2 in, 2 out]
            n1759 = disable-structure shown="RUN_TIME_ENGINE==True" {
              disable-tunnel: w3661 -> [_ _]
              frame condition #0 {
                n1760 = Quit LabVIEW() -> ()  [unwired: 1 in]
              }
              frame condition #1 (active) {
              }
            }
          }
        }
        n1761 = global write "Results_plotter_Global.vi" "Plot EnFlo Tunnel Display"(FALSE ("Plot EnFlo Tunnel Display")) -> ()
        n1762 = local write "stop"(w3649) -> ()
        n1763 = property on="stop" class="Bool (strict)"("Val(Sgnl)"=w3649) -> ()  [unwired: 2 in, 2 out]
      }
      frame "No Match", Default {
        n1764 = call "Case not matched.vi"("Case Name not Matched"=w3667) -> ()
      }
    }
    "Current" <- w39
    "-1" <- w28
    "loop" <- w27
    "-2" <- w26
    "-3" <- w22
    "-4" <- w21
  }
  n1765 = while {
    tunnel: w13 -> [w3676]
    tunnel: w4 -> [w3675]
    tunnel: w2 -> [w3674]
    tunnel: w1 -> [w3673]
    stop <- w3678 stop-if-true
    # "Event structure wrapper"
    n1766 = event shown="[63] \"...using routine\": Value Change" {
      selector: _ -> [_ _ _ _ _ _ _ _ _ _ _ _ _ _ _ _ _ _ _ _ _ _ _ _ _ _ _ _ _ _ _ _ _ _ _ _ _ _ _ _ _ _ _ _ _ _ _ _ _ _ _ _ _ _ _ _ _ _ _ _ _ _ _ _]
      dyn-events: _ -> [_ _ _ _ _ _ _ _ _ _ _ _ _ _ _ _ _ _ _ _ _ _ _ _ _ _ _ _ _ _ _ _ _ _ _ _ _ _ _ _ _ _ _ _ _ _ _ _ _ _ _ _ _ _ _ _ _ _ _ _ _ _ _ _]
      timeout: 400 -> [_ _ _ _ _ _ _ _ _ _ _ _ _ _ _ _ _ _ _ _ _ _ _ _ _ _ _ _ _ _ _ _ _ _ _ _ _ _ _ _ _ _ _ _ _ _ _ _ _ _ _ _ _ _ _ _ _ _ _ _ _ _ _ _]
      tunnel: [_ _ _ _ _ _ _ _ _ _ _ _ _ _ _ _ _ _ _ _ _ _ _ _ _ _ _ _ _ _ _ _ _ _ _ _ _ _ _ _ _ FALSE ("NewVal") w3927 _ _ _ _ _ _ _ _ _ _ _ _ _ _ _ _ _ _ _ _ _] -> w3678
      tunnel: w3676 -> [_ _ _ _ _ _ _ _ _ _ _ _ _ _ _ _ _ _ _ _ _ _ _ _ _ _ _ _ _ _ _ _ _ _ _ _ _ _ _ _ _ _ _ _ _ _ _ _ _ _ _ _ _ _ _ _ w4013 _ _ _ _ _ _ _]
      tunnel: w3675 -> [_ _ _ _ _ _ _ _ _ _ _ _ _ _ w3830 _ _ _ _ _ _ _ _ _ _ _ _ _ _ _ _ _ _ _ _ _ _ _ _ _ _ w3921 _ _ _ _ _ _ _ _ _ _ _ _ _ _ _ _ _ _ _ _ _ _]
      tunnel: w3674 -> [_ _ w3762 _ _ _ _ _ _ _ _ _ _ _ _ _ _ _ _ _ _ _ _ _ _ _ _ _ _ _ _ _ _ _ _ _ _ _ _ _ _ _ _ _ _ _ _ _ _ _ _ _ _ _ _ _ _ _ _ _ _ _ _ _]
      tunnel: w3673 -> [_ _ w3761 _ _ _ _ _ _ _ _ _ _ _ _ _ _ _ _ _ _ _ _ _ _ _ _ _ _ _ _ _ _ _ _ _ _ _ _ _ _ _ _ _ _ _ _ _ _ _ _ _ _ _ _ _ _ _ _ _ _ _ _ w4123]
      event Timeout {
        # "Moved from \"What to do next 3rd\""
        # "finagle graph and legend size, to cope with change of legend"
        n1767 = event-data() -> ()  [unwired: 1 in, 3 out]
        n1768 = local read "Show Results Space Analysis"() -> (w3686:bool)
        n1769 = control-ref of="This VI"() -> (w3691:refnum<vi>)
        n1770 = local read "Show Plot Space Analysis"() -> (w3687:bool)
        n1771 = while {
          shift-right: [w3706] -> _
          shift-left: _ -> [w3705]
          shift-left: _ -> [w3704]
          shift-left: _ -> [w3703]
          tunnel: w3686 -> [w3706]
          shift-right: [w3711] -> _
          shift-left: _ -> [w3710]
          shift-left: _ -> [w3709]
          shift-left: _ -> [w3708]
          tunnel: w3687 -> [w3711]
          tunnel: [w3707] -> w3688
          tunnel: [w3702] -> w3689
          stop <- TRUE stop-if-true
          n1772 = Compound Arithmetic op=AND(w3706, w3705, w3704, w3703) -> (w3702:bool)
          n1773 = Compound Arithmetic op=AND(w3711, w3710, w3709, w3708) -> (w3707:bool)
        }
        n1774 = global write "Results_plotter_Global.vi" "Max no of filter options"("Max no of filter options") -> ()
        n1775 = property class="VI"(reference=w3691) -> ("Minimum Panel Size"=w3692:T22, "Front Panel.PanelBounds"=w3693:T23)  [unwired: 1 in, 2 out]
        n1776 = control-ref of="XY Plot"() -> (w3690:refnum<vi>)
        n1777 = case shown="True" w3689 {
          frame False {
          }
          frame True {
            n1778 = Open VI Reference(vi path="Results_Space_Analysis.vi" ("VI path")) -> (vi reference=w3717:refnum<vi>, error out=w3716:errorcluster)  [unwired: 1 in, 4 out]
            n1779 = property class="VI"(reference=w3717, error in=w3716) -> (reference out=w3715:refnum<vi>, error out=w3714:errorcluster, "Front Panel Window:Open"=w3712:bool)
            n1780 = local write "Show Results Space Analysis"(w3712) -> ()
            n1781 = Close Reference(reference=w3715, error in (no error)=w3714) -> ()  [unwired: 1 out]
          }
        }
        n1782 = case shown="True" w3688 {
          frame False {
          }
          frame True {
            n1783 = Open VI Reference(vi path="Plot_Space_Analysis.vi" ("VI path")) -> (vi reference=w3723:refnum<vi>, error out=w3722:errorcluster)  [unwired: 1 in, 4 out]
            n1784 = property class="VI"(reference=w3723, error in=w3722) -> (reference out=w3721:refnum<vi>, error out=w3720:errorcluster, "Front Panel Window:Open"=w3718:bool)
            n1785 = local write "Show Plot Space Analysis"(w3718) -> ()
            n1786 = Close Reference(reference=w3721, error in (no error)=w3720) -> ()  [unwired: 1 out]
          }
        }
        n1787 = call "makeGraphLegend.vi"("Point"=w3692, "Rect"=w3693, "XYGraph in"=w3690) -> ()  [unwired: 9 in]
        n1788 = local read "Index when last displayed"() -> (w3684:i32)
        n1789 = local read "Index when last plotted"() -> (w3683:i32)
        n1790 = global write "Results_plotter_Global.vi" "Plot EnFlo Tunnel Display"("Plot EnFlo Tunnel Display") -> ()
        n1791 = Not Equal?(x=w3683, y=w3684) -> (x != y?=w3682:bool)
        n1792 = And(x=w3682, y="Plot EnFlo Tunnel Display") -> (x .and. y?=w3681:bool)
        n1793 = case shown="False" w3681 {
          tunnel: [w3694 "Full Res file manipulator" ("t")] -> w3679
          frame False {
            n1794 = local read "whereNext"() -> (w3695:string)
            n1795 = Empty String/Path?(string/path=w3695) -> (empty?=w3697:bool)
            n1796 = Select(t="Time to save setup?", s=w3697, f=w3695) -> (s? t:f=w3694:string)
          }
          frame True {
            n1797 = local write "Plotted rows only?"(TRUE ("Plotted rows only?")) -> ()
            n1798 = local write "Mode"(Plotter_Mode."Plot EnFlo Tunnel Display" ("Mode")) -> ()
          }
        }
        n1799 = local write "whereNext"(w3679) -> ()
      }
      event Panel Resize {
        # "Code to resize the \"Red\" and Green Multiselects as window grows"
        # "Ajust the multi-selector sizes with the panel"
        n1800 = event-data() -> ("VIRef"=w3751:refnum<vi>, "NewBnds"=w3744:T23)  [unwired: 1 in, 6 out]
        n1801 = property class="VI"(reference=w3751) -> ("Minimum Panel Size"=w3743:T22)  [unwired: 1 in, 2 out]
        n1802 = control-ref of="XY Plot"() -> (w3745:refnum<vi>)
        n1803 = Unbundle By Name(w3744) -> ("Right"=w3750:i16, "Left"=w3749:i16, "Bottom"=w3742:i16, "Top"=w3741:i16)
        n1804 = Unbundle By Name(w3743) -> ("Horizontal"=w3756:i16, "Vertical"=w3739:i16)
        n1805 = Subtract(x=w3750, y=w3749) -> (x-y=w3748:i16)
        n1806 = Subtract(x=w3742, y=w3741) -> (x-y=w3740:i16)
        n1807 = call "makeGraphLegend.vi"("Point"=w3743, "Rect"=w3744, "XYGraph in"=w3745) -> ()  [unwired: 9 in]
        n1808 = Subtract(x=w3740, y=w3739) -> (x-y=w3728:i16)
        n1809 = Subtract(x=w3748, y=w3756) -> (x-y=w3729:i16)
        n1810 = Bundle(w3729, w3728) -> (w3726:cluster{i16, i16})  [unwired: 1 in]
        n1811 = Add(x=w3726, y=T28 {"Width"=749, "Height"=364} ("Content Bounds")) -> (x+y=w3727:T28)
        n1812 = property on="3D Picture" class="SceneGraphDisp (strict)"("ContentBounds"=w3727) -> ()  [unwired: 2 in, 2 out]
        n1813 = Add(x=364 ("Position:Left"), y=w3728) -> (x+y=w3725:i32)
        n1814 = expression code="x*2/3"(w3729) -> (w3747:i16)
        n1815 = expression code="x*1/3"(w3729) -> (w3746:i16)
        n1816 = property on="histOn" class="Bool (strict)"("Left"=448 ("Position:Left"), "Top"=w3725) -> ()  [unwired: 2 in, 2 out]
        n1817 = property on="color and symbol" class="Bool (strict)"("Left"=318 ("Position:Left"), "Top"=w3725) -> ()  [unwired: 2 in, 2 out]
        n1818 = Add(x=w3729, y=i16 98) -> (x+y=w3753:i16)
        n1819 = Add(x=w3728, y=337 ("Position:Left")) -> (x+y=w3731:i32)
        n1820 = property on="Single Series" class="LstBox (strict)"("Width"=w3753) -> ()  [unwired: 2 in, 2 out]
        n1821 = Add(x=w3746, y=i16 274) -> (x+y=w3757:i16)
        n1822 = Add(x=w3747, y=i16 302) -> (x+y=w3754:i16)
        n1823 = Add(x=w3746, y=281) -> (x+y=w3759:i32)
        n1824 = property on="Transpose" class="Bool (strict)"("Left"=247 ("Position:Left"), "Top"=w3731) -> ()  [unwired: 2 in, 2 out]
        n1825 = property on="forceY0" class="Bool (strict)"("Left"=318 ("Position:Left"), "Top"=w3731) -> ()  [unwired: 2 in, 2 out]
        n1826 = property on="forceX0" class="Bool (strict)"("Left"=357 ("Position:Left"), "Top"=w3731) -> ()  [unwired: 2 in, 2 out]
        n1827 = property on="refresh" class="Bool (strict)"("Left"=413 ("Position:Left"), "Top"=w3731) -> ()  [unwired: 2 in, 2 out]
        n1828 = property on="Filter Bins 2" class="LstBox (strict)"("Width"=w3754, "Left"=w3759) -> ()  [unwired: 2 in, 2 out]
        n1829 = property on="Filter Bins 1" class="LstBox (strict)"("Width"=w3757) -> ()  [unwired: 2 in, 2 out]
      }
      event "Tab Control": Value Change {
        n1830 = event-data() -> ("NewVal"=w3763:T1)  [unwired: 1 in, 5 out]
        n1831 = case shown="\"Edit\"" w3763 {
          tunnel: w3762 -> [_ _ _]
          tunnel: w3761 -> [_ _ w3765]
          frame "Load ", Default {
          }
          frame "Cursor" {
            n1832 = local write "whereNext"("Read Cursor" ("whereNext")) -> ()
          }
          frame "Edit" {
            n1833 = List Folder(path=w3765) -> (filenames=w3767:string[])  [unwired: 3 in, 3 out]
            n1834 = Empty Array?(array=w3767) -> (empty?=w3768:bool)
            n1835 = case shown="False" w3768 {
              tunnel: w3767 -> [w3772 _]
              tunnel: "Reveal Calculation VIs Folder" ("element") -> [w3769 _]
              frame False {
                n1836 = Build Array (concatenate)("", w3769, w3772) -> (w3771:string[])
                n1837 = property on="...using routine" class="CmbBox"("Strings[]"=w3771) -> ()  [unwired: 2 in, 2 out]
              }
              frame True {
              }
            }
          }
        }
      }
      event "graphPaneTab": Value Change {
        n1838 = event-data() -> ("OldVal"=w3774:T7, "NewVal"=w3773:T7)  [unwired: 1 in]
        n1839 = control-ref of="3D Picture"() -> (w3777:refnum<vi>)
        n1840 = case shown="\"3-D vector\"" w3774 {
          frame "XY", Default {
          }
          frame "Contour" {
          }
          frame "3-D graphs" {
          }
          frame "3-D vector" {
            # "Abort if leaving tab, to unfreeze stuff"
            n1841 = global write "Results_plotter_Global.vi" "3DgiveUp"(TRUE ("3DgiveUp")) -> ()
          }
          frame "Other Plots" {
          }
          frame "Storage" {
          }
          frame "debug" {
          }
        }
        n1842 = Close Reference(reference=w3777) -> (error out=w3776:errorcluster)  [unwired: 1 in]
        n1843 = case shown="\"3-D vector\"" w3773 {
          tunnel: w3776 -> [_ _ _ _ _]
          tunnel: [_ _ _ _ TRUE ("Visible")] -> w3775
          frame "Storage", Default {
          }
          frame "XY" {
            n1844 = property on="Intensity Plot?" class="Bool (strict)"("Val(Sgnl)"=FALSE ("Intensity Plot?")) -> ()  [unwired: 2 in, 2 out]
            n1845 = local write "whereNext"("Plot Data") -> ()
          }
          frame "Contour" {
            n1846 = property on="Intensity Plot?" class="Bool (strict)"("Val(Sgnl)"=TRUE ("Intensity Plot?")) -> ()  [unwired: 2 in, 2 out]
          }
          frame "3-D graphs" {
            n1847 = property on="Intensity Plot?" class="Bool (strict)"("Val(Sgnl)"=TRUE ("Intensity Plot?")) -> ()  [unwired: 2 in, 2 out]
          }
          frame "3-D vector" {
            n1848 = flat-sequence {
              frame #0 {
                n1849 = global write "Results_plotter_Global.vi" "3DgiveUp"(FALSE ("3DgiveUp")) -> ()
              }
              frame #1 {
                n1850 = local write "whereNext"("3Dvectors" ("whereNext")) -> ()
              }
            }
          }
        }
        n1851 = property on="FOV" class="Slide (strict)"("Visible"=w3775) -> ()  [unwired: 2 in, 2 out]
        n1852 = property on="underCursor" class="Str"("Visible"=w3775) -> ()  [unwired: 2 in, 2 out]
      }
      event "Filter Bins 1", "Filter Bins 2", "Filter 3", "Filter 4", "Filter 5", "Filters 3 onwards": Value Change {
        n1853 = event-data() -> ()  [unwired: 1 in, 1 out]
        n1854 = local write "whereNext"("Plot Data" ("whereNext")) -> ()
      }
      event "SearchY": Value Change {
        n1855 = event-data() -> ("NewVal"=w3788:string)  [unwired: 1 in]
        n1856 = Empty String/Path?(string/path=w3788) -> (empty?=w3787:bool)
        n1857 = case shown="False" w3787 {
          frame False {
            n1858 = property on="Multi Ordinate" class="LstBox (strict)"() -> ("Item Names"=w3790:string[])  [unwired: 2 in, 2 out]
            n1859 = for {
              tunnel: w3790 -> [w3797] mode=indexing
              tunnel: "SearchY" -> [w3796]
              i -> [w3795]
              stop <- w3793 stop-if-true
              n1860 = To Upper Case(1:w3797) -> (0:w3792:string)
              n1861 = To Upper Case(1:w3796) -> (0:w3791:string)
              n1862 = Match Pattern(string=w3792, regular expression=w3791) -> (offset past match=w3794:i32)  [unwired: 1 in, 3 out]
              n1863 = case shown="0, Default" w3794 {
                tunnel: w3795 -> [_ w3799]
                tunnel: [FALSE TRUE] -> w3793
                frame -1 {
                }
                frame 0, Default {
                  n1864 = Build Array(w3799) -> (w3801:i32[])
                  n1865 = property on="Multi Ordinate" class="LstBox (strict)"("Val(Sgnl)"=w3801, "Top Row"=w3799) -> ()  [unwired: 2 in, 2 out]
                }
              }
            }
          }
          frame True {
          }
        }
      }
      event "SearchX": Value Change {
        n1866 = event-data() -> ("NewVal"=w3803:string)  [unwired: 1 in]
        n1867 = Empty String/Path?(string/path=w3803) -> (empty?=w3802:bool)
        n1868 = case shown="False" w3802 {
          frame False {
            n1869 = property on="Absisca" class="Ring (strict)"() -> ("Strings []"=w3804:string[])  [unwired: 2 in, 2 out]
            n1870 = for {
              tunnel: w3804 -> [w3812] mode=indexing
              tunnel: "SearchX" -> [w3811]
              i -> [w3810]
              stop <- w3808 stop-if-true
              n1871 = To Upper Case(1:w3811) -> (0:w3806:string)
              n1872 = To Upper Case(1:w3812) -> (0:w3807:string)
              n1873 = Match Pattern(string=w3807, regular expression=w3806) -> (offset past match=w3809:i32)  [unwired: 1 in, 3 out]
              n1874 = case shown="0, Default" w3809 {
                tunnel: w3810 -> [_ w3814]
                tunnel: [FALSE TRUE] -> w3808
                frame -1 {
                }
                frame 0, Default {
                  n1875 = property on="Absisca" class="Ring (strict)"("Val(Sgnl)"=w3814, "RingText.Scroll Position"=w3814) -> ()  [unwired: 2 in, 2 out]
                }
              }
            }
          }
          frame True {
          }
        }
      }
      event "XY Plot": Cursor Move {
        n1876 = event-data() -> ()  [unwired: 1 in, 10 out]
        n1877 = local write "whereNext"("Read Cursor" ("whereNext")) -> ()
      }
      event "XY Plot": Plot Attribute Change {
        n1878 = event-data() -> ()  [unwired: 1 in, 8 out]
        n1879 = local read "histOn"() -> (w3817:bool)
        n1880 = case shown="True" w3817 {
          frame False {
          }
          frame True {
            n1881 = for {
              N: 10 -> [_]
              i -> [w3819]
              n1882 = property on="XY Plot" class="XYGraph (strict)"("Active Plot"=w3819) -> ("Plot.Visible?"=w3820:bool)  [unwired: 2 in, 2 out]
              n1883 = property on="Histogram" class="XYGraph (strict)"("Active Plot"=w3819, "Plot.Visible?"=w3820) -> ()  [unwired: 2 in, 2 out]
            }
          }
        }
      }
      event "XY Plot": Cursor Grab {
        n1884 = event-data() -> ()  [unwired: 1 in, 9 out]
        "cursorDrag" <- TRUE ("cursorDrag")
      }
      event "XY Plot": Cursor Release {
        n1885 = event-data() -> ()  [unwired: 1 in, 10 out]
        n1886 = flat-sequence {
          frame #0 {
            n1887 = local write "cursorDrag"(FALSE ("cursorDrag")) -> ()
          }
          frame #1 {
            n1888 = local write "whereNext"("Read Cursor" ("whereNext")) -> ()
          }
        }
      }
      event "XY Plot": Value Change {
        n1889 = event-data() -> ()  [unwired: 1 in, 6 out]
        n1890 = local write "whereNext"("Read Cursor" ("whereNext")) -> ()
      }
      event "forceY0", "forceX0", "histOn": Value Change {
        n1891 = event-data() -> ()  [unwired: 1 in, 6 out]
        n1892 = local write "whereNext"("Plot Data" ("whereNext")) -> ()
      }
      event "seriesColours", "brewSelect", "TinyPoints?", "InterpolationStyle": Value Change {
        n1893 = event-data() -> ()  [unwired: 1 in, 6 out]
        n1894 = local write "whereNext"("Plot Data" ("t")) -> ()
        n1895 = global write "Results_plotter_Global.vi" "InterpolationStyle"("InterpolationStyle") -> ()
        n1896 = global write "Results_plotter_Global.vi" "TinyPoints?"("TinyPoints?") -> ()
      }
      event "ShowPix": Value Change {
        n1897 = event-data() -> ("NewVal"=w3829:bool)  [unwired: 1 in, 5 out]
        n1898 = call "Open_Close_Front_Panel.ph.vi"("openWindow (T)"=w3829, "VI path"=w3830) -> ()  [unwired: 1 in, 1 out]
        n1899 = case shown="True" w3829 {
          tunnel: [T29."Disabled and Grayed Out" ("Disabled") T29."Enabled" ("Disabled")] -> w3831
          frame False {
          }
          frame True {
            n1900 = local write "cursorDrag"(FALSE ("cursorDrag")) -> ()
            n1901 = local write "whereNext"("Read Cursor" ("whereNext")) -> ()
          }
        }
        n1902 = property on="picMode" class="RadioBtnsControl (strict)"("DisabledEnum"=w3831) -> ()  [unwired: 2 in, 2 out]
      }
      event "Reload Files": Mouse Up; "Reload Interval (s)": Value Change {
        n1903 = event-data() -> ()  [unwired: 1 in, 4 out]
        n1904 = local read "Template"() -> (w3837:path)
        n1905 = global write "Results_plotter_Global.vi" "Template"(w3837) -> ()
        n1906 = local write "whereNext"("Initialise") -> ()
      }
      event "flushAll": Mouse Up {
        n1907 = event-data() -> ()  [unwired: 1 in, 1 out]
        n1908 = case shown="True" "flushAll" {
          tunnel: "flushAll" -> [_ w3841]
          frame False {
          }
          frame True {
            n1909 = local write "flushAll"(FALSE ("flush")) -> ()
            n1910 = property on="flushFiles" class="Bool (strict)"("Val(Sgnl)"=w3841) -> ()  [unwired: 2 in, 2 out]
            n1911 = local write "Template"(path "") -> ()
          }
        }
      }
      event "flushFiles": Value Change {
        n1912 = event-data() -> ()  [unwired: 1 in, 6 out]
        n1913 = local write "whereNext"("Empty Results file array" ("t")) -> ()
      }
      event "Add results file": Value Change {
        n1914 = event-data() -> ()  [unwired: 1 in, 6 out]
        n1915 = local write "whereNext"("More files options") -> ()
      }
      event "Edit Template File": Value Change {
        n1916 = event-data() -> ()  [unwired: 1 in, 6 out]
        n1917 = case shown="True" "Edit Template File" {
          tunnel: ["" "Edit template file" ("t")] -> w3844
          frame False {
          }
          frame True {
          }
        }
        n1918 = local write "whereNext"(w3844) -> ()
      }
      event "Choose\nPlug ins": Value Change {
        n1919 = event-data() -> ()  [unwired: 1 in, 6 out]
        n1920 = local write "whereNext"("Process Cursor Point" ("t")) -> ()
      }
      event "Save Averaged rows": Value Change {
        n1921 = event-data() -> ()  [unwired: 1 in, 6 out]
        n1922 = local write "whereNext"("What type of row averaging?" ("t")) -> ()
      }
      event "Save Data in Rows": Value Change; "Save Data in Rows": Mouse Up {
        n1923 = event-data() -> ()  [unwired: 1 in, 2 out]
        n1924 = case shown="True" "Save Data in Rows" {
          frame False {
          }
          frame True {
            n1925 = local write "whereNext"("Save Data in Rows") -> ()
          }
        }
      }
      event "Save Plot data", "Save Surface Fit": Value Change {
        n1926 = event-data() -> ()  [unwired: 1 in, 6 out]
        n1927 = local write "whereNext"("Save Plot Data") -> ()
      }
      event "passToPictureVI": Value Change {
        n1928 = event-data() -> ()  [unwired: 1 in, 6 out]
        n1929 = local write "whereNext"("Create Plot summary") -> ()
      }
      event "Show Results Space Analysis": Value Change {
        # "Moved from \"Time to save setup?\""
        n1930 = event-data() -> ("NewVal"=w3854:bool)  [unwired: 1 in, 5 out]
        n1931 = Open VI Reference(vi path="Results_Space_Analysis.vi" ("VI path")) -> (vi reference=w3856:refnum<vi>, error out=w3857:errorcluster)  [unwired: 1 in, 4 out]
        n1932 = property class="VI"(reference=w3856, error in=w3857, "Front Panel Window:Open"=w3854) -> (reference out=w3858:refnum<vi>, error out=w3859:errorcluster)
        n1933 = Close Reference(reference=w3858, error in (no error)=w3859) -> ()  [unwired: 1 out]
      }
      event "Show Plot Space Analysis": Value Change {
        # "Moved from \"Time to save setup?\""
        n1934 = event-data() -> ("NewVal"=w3862:bool)  [unwired: 1 in, 5 out]
        n1935 = Open VI Reference(vi path="Plot_Space_Analysis.vi" ("VI path")) -> (vi reference=w3861:refnum<vi>, error out=w3864:errorcluster)  [unwired: 1 in, 4 out]
        n1936 = property class="VI"(reference=w3861, error in=w3864, "Front Panel Window:Open"=w3862) -> (reference out=w3860:refnum<vi>, error out=w3865:errorcluster)
        n1937 = Close Reference(reference=w3860, error in (no error)=w3865) -> ()  [unwired: 1 out]
      }
      event "Process Point": Value Change {
        n1938 = event-data() -> ()  [unwired: 1 in, 6 out]
        n1939 = local write "whereNext"("Process cursor point" ("t")) -> ()
      }
      event "Kill Point": Value Change {
        w3867 = TRUE ("Plotted rows only?")
        n1940 = event-data() -> ()  [unwired: 1 in, 6 out]
        n1941 = local write "Plotted rows only?"(w3867) -> ()
        n1942 = Build Array(string[] ["PointKilled"] ("New Values In")) -> (w3869:string[][])
        n1943 = global write "Results_plotter_Global.vi" "New Chs In"(string[] ["Omit::"] ("New Chs In")) -> ()
        n1944 = global write "Results_plotter_Global.vi" "New Values In"(w3869) -> ()
        n1945 = local write "Mode"(Plotter_Mode."Edit Values with constants" ("Mode")) -> ()
        n1946 = local write "whereNext"("Full Res file manipulator" ("t")) -> ()
        "justCursorPt" <- w3867
      }
      event "Delete Plotted data from file": Value Change {
        n1947 = event-data() -> ()  [unwired: 1 in, 6 out]
        n1948 = case shown="True" "Delete Plotted data from file" {
          frame False {
          }
          frame True {
            n1949 = local write "Plotted rows only?"(TRUE ("Save Plotted rows only?")) -> ()
            n1950 = local write "Mode"(Plotter_Mode."Delete unwanted rows" ("Mode")) -> ()
            n1951 = local write "whereNext"("Full Res file manipulator" ("t")) -> ()
          }
        }
      }
      event "Post Process Plotted Data": Value Change {
        n1952 = event-data() -> ()  [unwired: 1 in, 6 out]
        n1953 = local write "Plotted rows only?"(TRUE ("Plotted rows only?")) -> ()
        n1954 = local write "Mode"(Plotter_Mode."Post Process Plotted Rows" ("Mode")) -> ()
        n1955 = local write "whereNext"("Full Res file manipulator" ("t")) -> ()
      }
      event "Add /Edit metadata": Value Change {
        n1956 = event-data() -> ()  [unwired: 1 in, 6 out]
        n1957 = local write "whereNext"("Add or Edit Metadata" ("t")) -> ()
      }
      event "Calculate new metadata": Value Change {
        n1958 = event-data() -> ()  [unwired: 1 in, 6 out]
        n1959 = local write "whereNext"("Run Calculation Routine" ("t")) -> ()
      }
      event "Add Inlet Temperature offset": Value Change {
        n1960 = event-data() -> ()  [unwired: 1 in, 6 out]
        n1961 = case shown="True" "Add Inlet Temperature offset" {
          frame False {
          }
          frame True {
            n1962 = local write "Plotted rows only?"(TRUE ("Plotted rows only?")) -> ()
            n1963 = local write "whereNext"("Full Res file manipulator" ("t")) -> ()
            n1964 = local write "Mode"(Plotter_Mode."Add Inlet Temperature Offset" ("Mode")) -> ()
          }
        }
      }
      event "Dot Plot?": Value Change {
        n1965 = event-data() -> ()  [unwired: 1 in, 6 out]
        n1966 = case shown="True" "Dot Plot?" {
          frame False {
          }
          frame True {
            n1967 = local write "whereNext"("Coloured Dot Plot" ("t")) -> ()
          }
        }
      }
      event "Vector Plot?": Value Change {
        n1968 = event-data() -> ()  [unwired: 1 in, 6 out]
        n1969 = local write "whereNext"("Vector Plot" ("t")) -> ()
      }
      event "MakeMovie": Value Change {
        # "Retrieve path for Raw Data File; use to retrieve matching webcam pictures"
        n1970 = event-data() -> ("NewVal"=w3889:bool)  [unwired: 1 in, 5 out]
        n1971 = case shown="True" w3889 {
          frame False {
          }
          frame True {
            w3896 = "-" ("string")
            n1972 = global read "Results_plotter_Global.vi" "Filters 3 onwards"() -> (w3897:string[])
            n1973 = global read "Results_plotter_Global.vi" "Filter 2 Strings"() -> (w3894:string[])
            n1974 = global read "Results_plotter_Global.vi" "Filter 1 Strings"() -> (w3892:string[])
            n1975 = Array To Spreadsheet String(delimiter (Tab)="-", array=w3897, 3:"%s" ("format string")) -> (spreadsheet string=w3900:string)
            n1976 = global read "Results_plotter_Global.vi" "Plot Metadata"() -> (w3890:T31[])
            n1977 = call "filterStringsToString.vi"("filterStrings"=w3894) -> ("flatString"=w3895:string)  [unwired: 10 in]
            n1978 = call "filterStringsToString.vi"("filterStrings"=w3892) -> ("flatString"=w3893:string)  [unwired: 10 in]
            n1979 = Search/Split String(string=w3900, search string/char (-)="\n") -> (substring before match=w3902:string)  [unwired: 1 in, 2 out]
            n1980 = Concatenate Strings(w3893, w3896, w3895, w3896, w3902) -> (w3891:string)
            n1981 = local read "Result files to read"() -> (w3905:path[])
            n1982 = local read "Job Directory"() -> (w3904:path)
            n1983 = local read "Template"() -> (w3903:path)
            n1984 = call "MakeProfileMovies.vi"("Plot Metadata"=w3890, "Job Directory"=w3904, "templatePath"=w3903, "Result files to read"=w3905, "suggestedName"=w3891) -> ()  [unwired: 5 in, 2 out]
          }
        }
      }
      event "axes": Value Change {
        n1985 = event-data() -> ("NewVal"=w3908:T3)  [unwired: 1 in, 5 out]
        n1986 = case shown="\"X log Y log\"" w3908 {
          tunnel: [w3909 w3910 1 0] -> w3907
          tunnel: [w3909 w3910 0 1] -> w3906
          frame "X lin Y lin", Default {
            w3909 = 0
          }
          frame "X log Y log" {
            w3910 = 1
          }
          frame "X log Y lin" {
          }
          frame "X lin Y log" {
          }
        }
        n1987 = property on="XY Plot" class="XYGraph (strict)"("XScale.Mapping Mode"=w3907, "YScale.Mapping Mode"=w3906) -> ()  [unwired: 2 in, 2 out]
      }
      event "graphBackground": Value Change {
        n1988 = event-data() -> ()  [unwired: 1 in, 6 out]
        n1989 = property on="XY Plot" class="XYGraph (strict)"("BG Color"="graphBackground") -> ()  [unwired: 2 in, 2 out]
      }
      event "Save Setup": Value Change {
        n1990 = event-data() -> ()  [unwired: 1 in, 6 out]
        n1991 = case shown="True" "Save Setup" {
          frame False {
          }
          frame True {
            n1992 = local write "whereNext"("Save Setup") -> ()
          }
        }
      }
      event "loadSetup": Value Change {
        n1993 = event-data() -> ()  [unwired: 1 in, 6 out]
        n1994 = case shown="True" "loadSetup" {
          frame False {
          }
          frame True {
            n1995 = local write "whereNext"("Choose Setup file" ("t")) -> ()
          }
        }
      }
      event Panel Close? {
        w3922 = TRUE ("stop")
        # "so the main loop knows a Window Close caused it"
        # "to make the event case see it"
        # "to make the button indicate it, and trigger main loop End"
        n1996 = event-data() -> ()  [unwired: 1 in, 4 out]
        n1997 = call "Open_Close_Front_Panel.ph.vi"("openWindow (T)"=FALSE, "VI path"=w3921) -> ()  [unwired: 1 in, 1 out]
        n1998 = property on="stop" class="Bool (strict)"("Val(Sgnl)"=w3922) -> ()  [unwired: 2 in, 2 out]
        n1999 = local write "stop"(w3922) -> ()
        n2000 = event-data("Discard?"=TRUE) -> ()  [unwired: 1 in, 1 out]
        "closePressed" <- w3922
      }
      event "stop": Value Change {
        n2001 = event-data() -> ("NewVal"=w3927:bool)  [unwired: 1 in, 5 out]
        n2002 = control-ref of="3D Picture"() -> (w3925:refnum<vi>)
        n2003 = local write "whereNext"("Save Setup" ("t")) -> ()
        n2004 = Close Reference(reference=w3925) -> ()  [unwired: 1 in, 1 out]
      }
      event "openJobDir": Mouse Up {
        n2005 = event-data() -> ()  [unwired: 1 in, 1 out]
        n2006 = local read "Job Directory"() -> (w3928:path)
        n2007 = call <vilib>:"Show in File System.vi"("file or directory path"=w3928) -> ()  [unwired: 10 in, 1 out]
      }
      event "revealOutputFile": Mouse Up {
        n2008 = event-data() -> ()  [unwired: 1 in, 1 out]
        n2009 = local read "Output Filename"() -> (w3929:path)
        n2010 = call <vilib>:"Show in File System.vi"("file or directory path"=w3929) -> ()  [unwired: 10 in, 1 out]
      }
      event "revealDataFiles": Mouse Up {
        n2011 = event-data() -> ()  [unwired: 1 in, 1 out]
        n2012 = local read "Result files to read"() -> (w3931:path[])
        n2013 = call "findSharedBasePath.vi"("arrayOfPaths"=w3931) -> ("commonRootPath"=w3930:path)  [unwired: 10 in]
        n2014 = call <vilib>:"Show in File System.vi"("file or directory path"=w3930) -> ()  [unwired: 10 in, 1 out]
      }
      event "Template": Value Change {
        n2015 = event-data() -> ()  [unwired: 1 in, 1 out]
        n2016 = local read "Template"() -> (w3933:path)
        n2017 = local write "whereNext"("Initialise") -> ()
        n2018 = global write "Results_plotter_Global.vi" "Template"(w3933) -> ()
      }
      event "printFP": Value Change {
        n2019 = event-data() -> ()  [unwired: 1 in, 1 out]
        n2020 = case shown="True" "printFP" {
          frame False {
          }
          frame True {
            n2021 = local read "Job Directory"() -> (w3943:path)
            n2022 = Build Path(base path=w3943, name or relative path="RFPprints") -> (appended path=w3937:path)
            n2023 = call <vilib>:"Create Directory Recursive.vi"("directory"=w3937) -> ("directory copy"=w3936:path)  [unwired: 4 in, 2 out]
            n2024 = Build Path(base path=w3936, name or relative path="RFP.png") -> (appended path=w3935:path)
            n2025 = call <vilib>:"Create File with Incrementing Suffix.vi"("file path"=w3935) -> ("error out"=w3938:errorcluster, "actual path"=w3940:path)  [unwired: 8 in, 1 out]
            n2026 = Current VI's Path() -> (path=w3944:path)
            n2027 = call "Save PNG Image of Front Panel.vi"("VI Path"=w3944, "File Path In"=w3940) -> ("File Path Out"=w3939:path)  [unwired: 8 in, 1 out]
            n2028 = call <vilib>:"Simple Error Handler.vi"("error in (no error)"=w3938) -> ()  [unwired: 4 in, 5 out]
            n2029 = call <vilib>:"Show in File System.vi"("file or directory path"=w3939) -> ()  [unwired: 10 in, 1 out]
          }
        }
      }
      event "importSetup": Value Change {
        n2030 = event-data() -> ()  [unwired: 1 in, 6 out]
        n2031 = case shown="True" "importSetup" {
          frame False {
          }
          frame True {
            n2032 = local write "whereNext"("importSetup") -> ()
          }
        }
      }
      event "exportSetup": Value Change {
        n2033 = event-data() -> ()  [unwired: 1 in, 6 out]
        n2034 = case shown="True" "exportSetup" {
          frame False {
          }
          frame True {
            n2035 = local write "whereNext"("exportSetup") -> ()
          }
        }
      }
      event "Filter Array": Value Change {
        n2036 = event-data() -> ()  [unwired: 1 in, 1 out]
        n2037 = local write "whereNext"("Create Selectors") -> ()
      }
      event "3Dplotter": Value Change {
        n2038 = event-data() -> ()  [unwired: 1 in, 1 out]
        n2039 = case shown="True" "3Dplotter" {
          frame False {
          }
          frame True {
            n2040 = local write "whereNext"("3Dpopout" ("t")) -> ()
          }
        }
      }
      event "3D Picture": Shortcut Menu Selection (User) {
        w3959 = sgl 1000.0 ("y")
        # "Prevents inside-out world!"
        n2041 = event-data() -> ("CtlRef"=w3953:refnum<vi>, "ItemTag"=w3954:string)  [unwired: 1 in, 6 out]
        n2042 = local read "depthClipping"() -> (w3958:cluster{sgl, sgl})
        n2043 = Unbundle(w3958) -> (w3960:sgl, w3961:sgl)
        n2044 = local read "3DrawDataPath"() -> (w3952:path)
        n2045 = Multiply(x=w3960, y=w3959) -> (x*y=w3962:sgl)
        n2046 = Multiply(x=w3961, y=w3959) -> (x*y=w3963:sgl)
        n2047 = local read "FOV"() -> (w3955:u8)
        n2048 = Max & Min(x=w3962, y=w3963) -> (max(x,y)=w3957:sgl, min(x,y)=w3956:sgl)
        n2049 = call "3DmenuHandler.vi"("nearClip"=w3956, "RawDataFile"=w3952, "farClip"=w3957, "FoV"=w3955, "ItemTag"=w3954, "3DpicRef"=w3953) -> ("error out"=w3964:errorcluster)  [unwired: 5 in]
        n2050 = invoke on="3D Picture" class="SceneGraphDisp (strict)" method="Redraw"(error in=w3964) -> ()  [unwired: 2 in, 3 out]
      }
      event "3D Picture": Mouse Move {
        w3972 = 0 ("disabled index (col)")
        n2051 = event-data() -> ("CtlRef"=w3975:refnum<vi>, "Coords"=w3976:T32)  [unwired: 1 in]
        n2052 = property on="Property Node" class="SceneGraphDisp (strict)"(reference=w3975) -> (reference out=w3979:refnum<vi>, "ContentPosition"=w3978:T32)  [unwired: 1 in, 1 out]
        n2053 = Subtract(x=w3976, y=w3978) -> (x-y=w3977:T32)
        n2054 = invoke on="Invoke Node" class="SceneGraphDisp (strict)" method="Pick Model"(reference=w3979, "Point"=w3977) -> ("Pick Model"=w3974:cluster{"Node Path":refnum<vi>[]}[])  [unwired: 2 in, 3 out]
        n2055 = for {
          tunnel: [w3987] -> _ mode=indexing
          tunnel: [w3985] -> w3973 mode=indexing
          tunnel: [w3984] -> _ mode=indexing
          tunnel: w3974 -> [w3983] mode=indexing
          n2056 = Unbundle(w3983) -> ("Node Path"=w3988:refnum<vi>[])
          n2057 = Reverse 1D Array(array=w3988) -> (reversed array=w3986:refnum<vi>[])
          n2058 = for {
            tunnel: [w3991] -> w3987 mode=indexing
            tunnel: w3986 -> [w3994] mode=indexing
            tunnel: [w3991] -> w3985 mode=indexing if=w3989
            tunnel: [w3990] -> w3984 mode=indexing if=w3989
            n2059 = property class="SceneObject"(reference=w3994) -> (reference out=w3990:refnum<vi>, "Name"=w3991:string, "Material.Ambient"=w3993:T33)  [unwired: 1 in, 1 out]
            n2060 = Unbundle By Name(w3993) -> ("Alpha"=w3992:sgl)
            n2061 = Not Equal To 0?(x=w3992) -> (x != 0?=w3989:bool)
          }
        }
        n2062 = Index Array(array=w3973, index (row)=w3972, index (col)=w3972) -> (element=w3971:string)
        n2063 = Search/Split String(string=w3971, search string/char (-)="<DATA_ROOT>") -> (substring before match=→"underCursor":string, match + rest of string=w3968:string)  [unwired: 1 in, 1 out]
        n2064 = call "String 2 Path memory.vi"("Input String"=w3968) -> ("path"=w3966:path)  [unwired: 1 in]
        "3DrawDataPath" <- w3966
        n2065 = local read "picMode"() -> (w3967:enum32{"Scrub", "Jump"})
        n2066 = local read "ShowPix"() -> (w3965:bool)
        n2067 = case shown="\"Scrub\", Default" w3967 {
          tunnel: w3965 -> [w3981 _]
          tunnel: w3966 -> [w3980 _]
          frame "Scrub", Default {
            n2068 = case shown="True" w3981 {
              tunnel: w3980 -> [_ w3982]
              frame False {
              }
              frame True {
                n2069 = call "DigUpPixAsync.vi"("File Path"=w3982) -> ()  [unwired: 11 in]
              }
            }
          }
          frame "Jump" {
          }
        }
      }
      event "3D Picture": Mouse Wheel {
        n2070 = event-data() -> ("Delta"=w4001:i32, "Orientation"=w3995:enum16{"Horizontal", "Vertical"}, "PlatMods"=w4000:T34)  [unwired: 1 in, 7 out]
        n2071 = Unbundle By Name(w4000) -> ("Shift"=w3999:bool)
        n2072 = Equal?(x=enum16{"Horizontal", "Vertical"}."Horizontal" ("Orientation"), y=w3995) -> (x = y?=w3997:bool)
        n2073 = Or(x=w3997, y=w3999) -> (x .or. y?=w3998:bool)
        n2074 = case shown="True" w3998 {
          tunnel: w4001 -> [w4003 _]
          frame False {
            # "Zoom lens in or out"
            n2075 = local read "FOV"() -> (w4002:u8)
            n2076 = Subtract(x=w4002, y=w4003) -> (x-y=w4004:i32)
            n2077 = In Range and Coerce(upper limit=sgl 110.0, x=w4004, lower limit=sgl 4.0) -> (coerced(x)=w4005:sgl)  [unwired: 1 out]
            n2078 = property on="FOV" class="Slide (strict)"("Val(Sgnl)"=w4005) -> ()  [unwired: 2 in, 2 out]
          }
          frame True {
            # "#Placeholder Once I work out how to retrieve the camera \"target\", use this case to update camera\nlocation along line from current location to target location"
            # "Dolly camera in or out"
            n2079 = invoke on="3D Picture" class="SceneGraphDisp (strict)" method="Redraw"() -> ()  [unwired: 3 in, 3 out]
          }
        }
      }
      event "3D Picture": Mouse Down {
        n2080 = event-data() -> ()  [unwired: 1 in, 1 out]
        n2081 = local read "3DrawDataPath"() -> (w4011:path)
        n2082 = local read "ShowPix"() -> (w4008:bool)
        n2083 = call <vilib>:"Is Path and Not Empty.vi"("path"=w4011) -> ("Is Path and Not Empty?"=w4009:bool)  [unwired: 4 in]
        n2084 = And(x=w4009, y=w4008) -> (x .and. y?=w4010:bool)
        n2085 = case shown="True" w4010 {
          tunnel: w4011 -> [_ w4012]
          frame False {
          }
          frame True {
            n2086 = call "DigUpPixAsync.vi"("File Path"=w4012) -> ()  [unwired: 11 in]
          }
        }
      }
      event "X Ch Name", "Y Ch Name", "Z Ch Name", "Wind Direction", "Coord System", "stl Filename", "Job Directory", "U Ch Name", "V Ch Name", "W Ch Name", "Xon", "Yon", "Zon", "Uon", "Von", "Won", "Point ID": Value Change {
        n2087 = event-data() -> ()  [unwired: 1 in, 6 out]
        n2088 = local read "Template"() -> (w4014:path)
        n2089 = stacked-sequence {
          tunnel: w4013 -> [_ w4036 _]
          tunnel: w4014 -> [_ w4032 w4062]
          frame #0 {
            n2090 = local read "graphPaneTab"() -> (w4015:T7)
            n2091 = case shown="\"3-D vector\"" w4015 {
              frame "XY", Default {
              }
              frame "Contour" {
              }
              frame "3-D graphs" {
              }
              frame "3-D vector" {
                # "Reverse tweek each time, so it doesn't accumulate!"
                # "Tweak size tiniest amount, to force redraw!"
                n2092 = local read "vectorDims"() -> (w4023:cluster{"vectorSize":sgl, "vectorScale":dbl})
                n2093 = Unbundle By Name(w4023) -> ("vectorSize"=w4022:sgl)
                n2094 = feedback #3(1e-05 ("nudger")) -> (w4018:dbl)
                n2095 = Negate(x=w4018) -> (-x=w4016:dbl)
                n2096 = feedback-in #3(w4016) -> ()
                n2097 = Compound Arithmetic op=ADD(w4022, w4016) -> (w4021:dbl)
                n2098 = Bundle By Name(cluster=w4023, "vectorSize"=w4021) -> (w4019:cluster{"vectorSize":sgl, "vectorScale":dbl})
                n2099 = call "Synchronize Data Flow.vim"("input 4"=w4019, "input 3"="What is present?" ("whereNext")) -> ("output 3"=w4020:string)  [unwired: 2 in, 3 out]
                n2100 = local write "vectorDims"(w4019) -> ()
                n2101 = local write "whereNext"(w4020) -> ()
              }
              frame "Other Plots" {
              }
              frame "Storage" {
              }
              frame "debug" {
              }
            }
          }
          frame #1 {
            n2102 = global read "Results_plotter_Global.vi" "All Template Ch Names"() -> (w4031:string[])
            n2103 = local read "Wind Direction"() -> (w4034:u16)
            n2104 = local read "Coord System"() -> (w4033:u16)
            n2105 = local read "stl Filename"() -> (w4028:u16)
            n2106 = local read "W Ch Name"() -> (w4025:u16)
            n2107 = local read "U Ch Name"() -> (w4027:u16)
            n2108 = local read "X Ch Name"() -> (w4046:u16)
            n2109 = local read "Y Ch Name"() -> (w4045:u16)
            n2110 = local read "Z Ch Name"() -> (w4044:u16)
            n2111 = local read "V Ch Name"() -> (w4026:u16)
            n2112 = Build Array(w4046, w4045, w4044, w4034, w4033, w4028, w4027, w4026, w4025) -> (w4043:u16[])
            n2113 = Build Array (concatenate)("None", w4031) -> (w4030:string[])
            n2114 = for {
              tunnel: w4030 -> [w4061]
              tunnel: w4043 -> [w4060] mode=indexing
              tunnel: [w4059] -> w4040 mode=indexing
              n2115 = Index Array(array=w4061, index=w4060) -> (element=w4059:string)
            }
            n2116 = local read "Template Single Values"() -> (w4039:string[])
            n2117 = call "Path_2_String.vi"("Real Path"="Job Directory") -> ("Path String"=w4041:string)
            n2118 = Build Array (concatenate)(w4040, w4041) -> (w4038:string[])
            n2119 = for {
              tunnel: Global_mode."Write Global to File" ("Mode") -> [w4054]
              tunnel: w4036 -> [w4052] mode=indexing
              tunnel: w4039 -> [w4048]
              tunnel: w4038 -> [w4051] mode=indexing
              tunnel: [w4051] -> w4035 mode=indexing
              tunnel: w4032 -> [w4050]
              i -> [w4049]
              n2120 = Index Array(array=w4048, index=w4049) -> (element=w4047:string)
              n2121 = Equal?(x=w4051, y=w4047) -> (x = y?=w4053:bool)
              n2122 = case shown="False" w4053 {
                tunnel: w4054 -> [w4058 _]
                tunnel: w4050 -> [w4057 _]
                tunnel: w4051 -> [w4056 _]
                tunnel: w4052 -> [w4055 _]
                frame False {
                  n2123 = call "Read_Write_Template.vi"("Template File"=w4057, "Mode"=w4058, "Single Value In"=w4056, "Data type"=w4055) -> ()  [unwired: 4 in, 8 out]
                }
                frame True {
                }
              }
            }
            n2124 = local write "Template Single Values"(w4035) -> ()
          }
          frame #2 {
            n2125 = File/Directory Info(path=w4062) -> (last mod=w4063:timestamp)  [unwired: 1 in, 6 out]
            n2126 = local write "Template Last Mod"(w4063) -> ()
          }
        }
      }
      event "vectorDims.vectorScale", "keySettings.clipPercentile", "keySettings.Centre Value", "vectorDims.vectorSize": Value Change {
        n2127 = event-data() -> ()  [unwired: 1 in, 1 out]
        n2128 = local write "whereNext"("3Dvectors" ("whereNext")) -> ()
      }
      event "FOV", "depthClipping", "lightPos", "Light State", "BGcolour": Value Change {
        w4083 = sgl 1000.0 ("y")
        # "Prevents inside-out world!"
        n2129 = event-data() -> ()  [unwired: 1 in, 1 out]
        n2130 = call <vilib>:"Color Change.vi"("Color"="BGcolour") -> ("RGBA"=w4068:cluster{"R":sgl, "G":sgl, "B":sgl, "A":sgl})  [unwired: 10 in]
        n2131 = property on="3D Picture" class="SceneGraphDisp (strict)"() -> ("Content Bounds.Width"=w4088:u32, "ContentBounds:Height"=w4089:u32)  [unwired: 2 in, 2 out]
        n2132 = property on="3D Picture" class="SceneGraphDisp (strict)"("Background Color"=w4068) -> (error out=w4067:errorcluster)  [unwired: 2 in, 1 out]
        n2133 = Unbundle("depthClipping") -> (w4085:sgl, w4084:sgl)
        n2134 = Multiply(x=w4085, y=w4083) -> (x*y=w4082:sgl)
        n2135 = Multiply(x=w4084, y=w4083) -> (x*y=w4081:sgl)
        n2136 = Divide(x=w4088, y=w4089) -> (x/y=w4087:dbl)
        n2137 = Max & Min(x=w4082, y=w4081) -> (max(x,y)=w4080:sgl, min(x,y)=w4079:sgl)
        n2138 = invoke on="3D Picture" class="SceneGraphDisp (strict)" method="Projection.Perspective"(error in=w4067, "Horizontal Field of View"="FOV", "Vertical Field of View"=w4087, "Near Clipping Plane"=w4079, "Far Clipping Plane"=w4080) -> (error out=w4066:errorcluster)  [unwired: 2 in, 6 out]
        n2139 = local read "worldRef"() -> (w4070:refnum<vi>)
        n2140 = call <vilib>:"New Light.vi"("error in (no error)"=w4066, "Light Number"=1) -> ("error out"=w4076:errorcluster, "New Light Refnum"=w4075:refnum<vi>)  [unwired: 8 in]
        n2141 = disable-structure shown="Disabled" {
          frame Disabled {
            n2142 = property class="SceneObject"("Blending.Bin"=T30."Transparent Bin" ("Blending:Bin")) -> ("Material.Color Mode"=w4092:T35, "Material.Shininess"=w4093:sgl)  [unwired: 2 in, 2 out]
          }
          frame Enabled {
          }
        }
        n2143 = Select(t=enum16{"Inherit Value", "Off", "On"}."On" ("Light State"), s="Light State", f=enum16{"Inherit Value", "Off", "On"}."Off" ("Light State")) -> (s? t:f=w4078:enum16{"Inherit Value", "Off", "On"})
        n2144 = call-poly <vilib>:"Set Light.vi"("Light State"=w4078, "error in (no error)"=w4076, "Position"="lightPos", "Light Refnum In"=w4075, "Scene Object In"=w4070) -> ("error out"=w4065:errorcluster)  [unwired: 5 in, 1 out]
        n2145 = invoke on="3D Picture" class="SceneGraphDisp (strict)" method="Redraw"(error in=w4065) -> ()  [unwired: 2 in, 3 out]
      }
      event "TTshift": Value Change {
        n2146 = event-data() -> ()  [unwired: 1 in, 1 out]
        n2147 = local read "TTshift"() -> (w4095:T9)
        n2148 = local read "TTref"() -> (w4096:refnum<vi>)
        n2149 = call "setTransforms.vi"("transform"=w4095, "SceneObject in"=w4096) -> ("error out"=w4094:errorcluster)  [unwired: 8 in, 1 out]
        n2150 = invoke on="3D Picture" class="SceneGraphDisp (strict)" method="Redraw"(error in=w4094) -> ()  [unwired: 2 in, 3 out]
      }
      event "axesLength": Value Change {
        n2151 = event-data() -> ()  [unwired: 1 in, 1 out]
        n2152 = local read "worldRef"() -> (w4110:refnum<vi>)
        n2153 = local read "axesRef"() -> (w4099:refnum<vi>)
        n2154 = local read "axesLength"() -> (w4097:dbl)
        n2155 = call <vilib>:"Color Change.vi"("Color"=u32 16764160) -> ("RGBA"=w4108:cluster{"R":sgl, "G":sgl, "B":sgl, "A":sgl})  [unwired: 10 in]
        n2156 = invoke class="SceneObject" method="Object.Remove Object"(reference=w4110, "Child"=w4099) -> (reference out=w4103:refnum<vi>, error out=w4098:errorcluster)  [unwired: 2 in, 2 out]
        n2157 = call <vilib>:"Create 3D Axis.vi"("Character Size"=sgl 20.0, "Axis label?"=TRUE, "Color"=w4108, "Radius"=sgl 4.0, "Length"=w4097, "Name"="tunnelAxes") -> ("New Object Refnum"=w4102:refnum<vi>)  [unwired: 4 in, 1 out]
        n2158 = Close Reference(reference=w4099, error in (no error)=w4098) -> ()  [unwired: 1 out]
        n2159 = call-poly <vilib>:"Add Object.vi"("New Object In"=w4102, "Scene Object In"=w4103) -> ("error out"=w4100:errorcluster, "New Object Out"=w4101:refnum<vi>)  [unwired: 7 in, 1 out]
        n2160 = local write "axesRef"(w4101) -> ()
        n2161 = invoke on="3D Picture" class="SceneGraphDisp (strict)" method="Redraw"(error in=w4100) -> ()  [unwired: 2 in, 3 out]
      }
      event "Turntable": Value Change {
        n2162 = event-data() -> ()  [unwired: 1 in, 1 out]
        n2163 = local read "TTstlBits"() -> (w4113:refnum<vi>[])
        n2164 = local read "Turntable"() -> (w4111:cluster{"colour":u32, "Alpha":sgl})
        n2165 = for {
          tunnel: w4113 -> [w4116] mode=indexing
          tunnel: [w4115] -> w4112
          tunnel: w4111 -> [w4114]
          n2166 = call "plainPaint.vi"("colourSpec"=w4114, "reference"=w4116) -> ("error out"=w4115:errorcluster)  [unwired: 8 in, 1 out]
        }
        n2167 = invoke on="3D Picture" class="SceneGraphDisp (strict)" method="Redraw"(error in=w4112) -> ()  [unwired: 2 in, 3 out]
      }
      event "Tunnel": Value Change {
        n2168 = event-data() -> ()  [unwired: 1 in, 1 out]
        n2169 = local read "tunnelSTLbits"() -> (w4119:refnum<vi>[])
        n2170 = local read "Tunnel"() -> (w4117:cluster{"colour":u32, "Alpha":sgl})
        n2171 = for {
          tunnel: w4119 -> [w4122] mode=indexing
          tunnel: [w4121] -> w4118
          tunnel: w4117 -> [w4120]
          n2172 = call "plainPaint.vi"("colourSpec"=w4120, "reference"=w4122) -> ("error out"=w4121:errorcluster)  [unwired: 8 in, 1 out]
        }
        n2173 = invoke on="3D Picture" class="SceneGraphDisp (strict)" method="Redraw"(error in=w4118) -> ()  [unwired: 2 in, 3 out]
      }
      event "...using routine": Value Change {
        n2174 = event-data() -> ("NewVal"=w4124:string)  [unwired: 1 in]
        n2175 = case shown="\"Reveal Calculation VIs Folder\"" w4124 {
          selector: w4124 -> [w4125 _]
          tunnel: w4123 -> [w4126 w4129]
          frame "False", Default {
            n2176 = Build Path(base path=w4126, name or relative path=w4125) -> (appended path=w4127:path)
            n2177 = call "Open_Close_Front_Panel.ph.vi"("openWindow (T)"=TRUE ("Front Panel Window:Open"), "VI path"=w4127) -> ()  [unwired: 1 in, 1 out]
          }
          frame "Reveal Calculation VIs Folder" {
            n2178 = call <vilib>:"Show in File System.vi"("file or directory path"=w4129) -> ()  [unwired: 10 in, 1 out]
          }
        }
      }
    }
  }
  n2179 = disable-structure shown="Disabled" {
    frame Disabled {
      n2180 = call "DigUpPixAsync.vi"() -> ()  [unwired: 12 in]
      n2181 = invoke on="3D Picture" class="SceneGraphDisp (strict)" method="Redraw"() -> ()  [unwired: 3 in, 3 out]
      n2182 = Unbundle() -> (w4139:T9, "STLscale"=w4140, "STLdTheta"=w4136, "Translation"=w4138)
      n2183 = Match Pattern(regular expression="TunFixed") -> (string=w4133:string, offset past match=w4130:i32)  [unwired: 1 in, 3 out]
      n2184 = invoke on="3D Picture" class="SceneGraphDisp (strict)" method="Reinit To Default"() -> ()  [unwired: 3 in, 3 out]
      n2185 = case shown="0, Default" w4130 {
        tunnel: [_ w4145] -> w4137
        tunnel: w4136 -> [w4142 w4144]
        tunnel: [w4142 w4143] -> w4135
        frame 0, Default {
        }
        frame -1 {
          n2186 = Add(x=w4145, y=w4144) -> (x+y=w4143:dbl)
        }
      }
      n2187 = Bundle(w4140, w4135, w4138) -> (w4134:cluster{void, dbl, void})  [unwired: 1 in]
      n2188 = call "loadSTL.vi"(6:w4134) -> ("STLname"=w4132:string, "Job Directory"=w4141:path)  [unwired: 7 in, 2 out]
      n2189 = local read "TTref"() -> ()  [unwired: 1 out]
    }
    frame Enabled {
    }
  }
